vi "Text control 2 v7.4.vi"() -> ()   [LabVIEW 2019]
panel:
  in  "Tab Control":enum32{"Main", "Other parameters"}(tab)
  out "Vdg vs time (Bias Stress)":cluster{"Y data in":dbl[], "X data in":dbl[]}[](graph)
  out "Vp vs Vg (FPP)":cluster{"Y data in":dbl[], "X data in":dbl[]}[](graph)
  out "Vp2":dbl format="%.2e"
  out "Vp1":dbl format="%.2e"
  out "Vp vs time (FPP Bias Stress)":cluster{"Y data in":dbl[], "X data in":dbl[]}[](graph)
  in  "Plot sample extrema vs time":bool
  out "Line running":i32
  out "Total lines":i32
  out "Path":path=path "C:/users/rlp38/09Apr2009LTtesting/test2.txt"
  out "I vs Vg":cluster{"Y data in":dbl[], "X data in":dbl[]}[](graph)
  out "Is max":dbl format="%.2e"
  out "Id max":dbl format="%.2e"
  out "Ig max":dbl format="%.2e"
  out "Imax vs time":cluster{"Y data in":dbl[], "X data in":dbl[]}[](graph)
  out "Imin vs time":cluster{"Y data in":dbl[], "X data in":dbl[]}[](graph)
  out "I vs Vd":cluster{"Y data in":dbl[], "X data in":dbl[]}[](graph)
  in  "Script":string="#pulsedstressV d 0.03 20 0 0.5 0.0827 5\n#\n#itime m\n#gaterangemode a\n#drainrangemode a\n#pulsed on 0.05 0 0.02\n#transfer d -10 40 1 5 40 35\n#transfer d -10 40 1 5 40 35\n#transfer d -10 40 1 5 40 35\n#output d 0 40 20 0 40 1\n#\n#\n#sample 1 0.008 221 6 0.003\n#samplei 400e-6 200 6 0.002 0.1\n#vsu2pulse -10 4\n#\n#stressV 0.016 0.03 2e-4 0.1e-3 11\n#stressI 220e-7 0.08 15\n#transfer s -1 1 0.5 -0.005 0.005 0.005\n#output s 0 0 0 -0.008 0.008 0.002"
  out "Command running:":string
  out "Serial port data":string
  out "Elapsed Time":dbl caption="Elapsed Time (s)"
  in  "Time Units":u16(ring)=1 items=["Seconds", "Minutes", "Hours"]
  in  "Time Offset":dbl caption="Set Start Time (s)"
  in  "Reset":bool
  in  "Auto Reset":bool
  in  "integration time":u32(slide) max=2 step=1 scale=0.0..2.0
  out "Is on":dbl format="%.2e"
  out "Id on":dbl format="%.2e"
  out "Ig on":dbl format="%.2e"
  out "Ion vs time":cluster{"Y data in":dbl[], "X data in":dbl[]}[](graph)
  out "Ioff vs time":cluster{"Y data in":dbl[], "X data in":dbl[]}[](graph)
  out "Ig min":dbl format="%.2e"
  out "Id min":dbl format="%.2e"
  out "Is min":dbl format="%.2e"
  out "Is off":dbl format="%.2e"
  out "Id off":dbl format="%.2e"
  out "Ig off":dbl format="%.2e"
  in  "Integration time (long)":dbl=0.32 min=0.04 max=2.0 step=0.02 format="%.2f"
  in  "Integration time (short)":dbl=0.0019 min=8e-05 max=0.0019 step=8e-05 format="%^.0e"
  in  "Drain: Compliance":dbl=0.001 format="%.8f"
  in  "Gate: Compliance":dbl=0.001 format="%.8f"
  in  "Interrupt scan":bool
  in  "Interrupt program":bool
  in  "Plot output curve extrema vs time":bool
  in  "Plot transfer curve extrema vs time":bool
  out "I vs time (Bias Stress)":cluster{"Y data in":dbl[], "X data in":dbl[]}[](graph)
  in  "Sample I - Probe 4 (Disabled)":u32(ring)=3 items=["SMU1  ", "SMU2  ", "SMU3  ", "SMU4  ", "SMU5  ", "SMU6  ", "VSU1  ", "VSU2  "]
  in  "Sample I - Source/Common":u32(ring) items=["SMU1  ", "SMU2  ", "SMU3  ", "SMU4  ", "SMU5  ", "SMU6  ", "VSU1  ", "VSU2  "]
  in  "Sample I - Probe 3 (Disabled)":u32(ring)=2 items=["SMU1  ", "SMU2  ", "SMU3  ", "SMU4  ", "SMU5  ", "SMU6  ", "VSU1  ", "VSU2  "]
  in  "Sample I - Drain/Gate":u32(ring)=1 items=["SMU1  ", "SMU2  ", "SMU3  ", "SMU4  ", "SMU5  ", "SMU6  ", "VSU1  ", "VSU2  "]
  in  "Sample - Probe 4":u32(ring)=3 items=["SMU1  ", "SMU2  ", "SMU3  ", "SMU4  ", "SMU5  ", "SMU6  ", "VSU1  ", "VSU2  "]
  in  "Sample - Source/Common":u32(ring) items=["SMU1  ", "SMU2  ", "SMU3  ", "SMU4  ", "SMU5  ", "SMU6  ", "VSU1  ", "VSU2  "]
  in  "Sample - Gate":u32(ring)=2 items=["SMU1  ", "SMU2  ", "SMU3  ", "SMU4  ", "SMU5  ", "SMU6  ", "VSU1  ", "VSU2  "]
  in  "Sample - Drain":u32(ring)=1 items=["SMU1  ", "SMU2  ", "SMU3  ", "SMU4  ", "SMU5  ", "SMU6  ", "VSU1  ", "VSU2  "]
  in  "Gate Range\nmode":u16(ring) items=["Auto", "Limited", "Fixed"]
  in  "Gate Range":u8(slide)=3 max=11 scale=0.0..11.0
  in  "Source/Drain\nRange mode":u16(ring) items=["Auto", "Limited", "Fixed"]
  in  "Source/Drain Range":u8(slide)=3 max=11 scale=0.0..11.0
  in  "Panel Controls":T1={"Emergency Stop"=refnum, "TransGraph Max"=1e-05, "Text/Graph (text=false)"=TRUE} {"TransGraph Max" format="%.2e"}
  in  "Panel Controls 2":T2={"Emergency Stop"=refnum, "TransGraph Max"=1e-05, "Text/Graph (text=false)"=TRUE, "TransGraph Min"=1e-11} {"TransGraph Min" format="%.2e"; "TransGraph Max" format="%.2e"}
  out "error out":errorcluster
  in  "Delay before read (ms)":u32=1000
  in  "byte count":u32=64
  in  "Serial End Mode for Reads":u16(ring)=2 items=["None", "LastBit", "TermChar"]
  in  "Timeout (ms)":u32=10000
  in  "Enable Termination\nChar (T)":bool=TRUE
  in  "Termination char\n(0xA = '\\n' = LF)\n(0xD = '\\r' = CR)":u8=13 format="%.0x"
  in  "flow control":u16(ring) items=["None"=0, "XON/XOFF"=1, "RTS/CTS"=2, "DTR/DSR"=4]
  in  "stop bits":u16(ring)=10 items=["1.0"=10, "1.5"=15, "2.0"=20]
  in  "parity":u16(ring) items=["None", "Odd", "Even", "Mark", "Space"]
  in  "data bits":u16=8 min=5 max=8 step=1
  in  "VISA resource name":refnum<visa-resource-name>="COM6"
  in  "baud rate":u32=9600
  out "Timings Indicator":T3
  in  "Timings (overwritten by the Front Panel)":T4={"integration time"=0, "Short/Long integration time"=0.00064, "hold time (sec)"=0.0, "delay time (sec)"=0.0, "Step Time (0 disables)"=0.0, "sweep method"=0, "Pulse period"=0.005, "Base voltage"=0.0, "Pulse width"=0.0005} {"Pulse width" min=0.0005 max=0.1 step=0.0001 format="%.4f"; "Base voltage" format="%^.4e"; "Pulse period" min=0.005 max=1.0 step=0.0001 format="%.4f"; "sweep method" items=["Continuous", "Pulsed"]; "Step Time (0 disables)" format="%.2f"; "delay time (sec)" format="%.4f"; "hold time (sec)" format="%.4f"; "Short/Long integration time" format="%^.0e"; "integration time" scale=0.0..2.0}
  in  "Probe 4":cluster{"on/off":bool, "Voltage":dbl} {"Voltage" min=-100.0 max=100.0 format="%.2f"}
  in  "Full Reset":bool
  in  "Standby":T5
  out "Probe 4 Indicator":cluster{"on/off":bool, "Voltage":dbl} {"Voltage" min=-100.0 max=100.0 format="%.2f"}
  in  "Transfer/Output - Drain":u32(ring)=1 items=["SMU1  ", "SMU2  ", "SMU3  ", "SMU4  ", "SMU5  ", "SMU6  ", "VSU1  ", "VSU2  "]
  in  "Transfer/Output - Gate":u32(ring)=2 items=["SMU1  ", "SMU2  ", "SMU3  ", "SMU4  ", "SMU5  ", "SMU6  ", "VSU1  ", "VSU2  "]
  in  "Transfer/Output - Source/Common":u32(ring) items=["SMU1  ", "SMU2  ", "SMU3  ", "SMU4  ", "SMU5  ", "SMU6  ", "VSU1  ", "VSU2  "]
  in  "Transfer/Output - Probe 4":u32(ring)=3 items=["SMU1  ", "SMU2  ", "SMU3  ", "SMU4  ", "SMU5  ", "SMU6  ", "VSU1  ", "VSU2  "]
  in  "Pulsed Stress V - Probe 4":u32(ring)=3 items=["SMU1  ", "SMU2  ", "SMU3  ", "SMU4  ", "SMU5  ", "SMU6  ", "VSU1  ", "VSU2  "]
  in  "Pulsed Stress V - Vextra":u32(ring)=6 items=["SMU1  ", "SMU2  ", "SMU3  ", "SMU4  ", "SMU5  ", "SMU6  ", "VSU1  ", "VSU2  "]
  in  "Pulsed Stress V - Drain":u32(ring)=1 items=["SMU1  ", "SMU2  ", "SMU3  ", "SMU4  ", "SMU5  ", "SMU6  ", "VSU1  ", "VSU2  "]
  in  "Pulsed Stress V - Source/Common":u32(ring) items=["SMU1  ", "SMU2  ", "SMU3  ", "SMU4  ", "SMU5  ", "SMU6  ", "VSU1  ", "VSU2  "]
  in  "Pulsed Stress V - Gate":u32(ring)=2 items=["SMU1  ", "SMU2  ", "SMU3  ", "SMU4  ", "SMU5  ", "SMU6  ", "VSU1  ", "VSU2  "]
  in  "FPP - Drain":u32(ring)=1 items=["SMU1  ", "SMU2  ", "SMU3  ", "SMU4  ", "SMU5  ", "SMU6  ", "VSU1  ", "VSU2  "]
  in  "FPP - Gate":u32(ring)=2 items=["SMU1  ", "SMU2  ", "SMU3  ", "SMU4  ", "SMU5  ", "SMU6  ", "VSU1  ", "VSU2  "]
  in  "FPP - Probe 1":u32(ring) items=["SMU1  ", "SMU2  ", "SMU3  ", "SMU4  ", "SMU5  ", "SMU6  ", "VSU1  ", "VSU2  "]
  in  "FPP - Probe 2":u32(ring)=3 items=["SMU1  ", "SMU2  ", "SMU3  ", "SMU4  ", "SMU5  ", "SMU6  ", "VSU1  ", "VSU2  "]
  in  "FPP - Source":u32(ring)=6 items=["SMU1  ", "SMU2  ", "SMU3  ", "SMU4  ", "SMU5  ", "SMU6  ", "VSU1  ", "VSU2  "]
  in  "Stress V - Drain":u32(ring)=1 items=["SMU1  ", "SMU2  ", "SMU3  ", "SMU4  ", "SMU5  ", "SMU6  ", "VSU1  ", "VSU2  "]
  in  "Stress V - Gate":u32(ring)=2 items=["SMU1  ", "SMU2  ", "SMU3  ", "SMU4  ", "SMU5  ", "SMU6  ", "VSU1  ", "VSU2  "]
  in  "Stress V - Source/Common":u32(ring) items=["SMU1  ", "SMU2  ", "SMU3  ", "SMU4  ", "SMU5  ", "SMU6  ", "VSU1  ", "VSU2  "]
  in  "Stress I - Drain/Gate":u32(ring)=1 items=["SMU1  ", "SMU2  ", "SMU3  ", "SMU4  ", "SMU5  ", "SMU6  ", "VSU1  ", "VSU2  "]
  in  "Stress I - Source/Common":u32(ring) items=["SMU1  ", "SMU2  ", "SMU3  ", "SMU4  ", "SMU5  ", "SMU6  ", "VSU1  ", "VSU2  "]
  in  "VSU2 Stress - Source/Common":u32(ring) items=["SMU1  ", "SMU2  ", "SMU3  ", "SMU4  ", "SMU5  ", "SMU6  ", "VSU1  "]
  in  "VISA resource name in":refnum<visa-resource-name>="GPIB0::14::INSTR"
  in  "Gate":T6={"Gate Start"=0.0, "Gate Stop"=2.0, "Gate Step (linear only)"=1.0, "Gate Compliance"=0.0001, "Gate PComp"=0.0, "Range mode"=0, "Range"=6} {"Range" max=11 scale=0.0..11.0; "Range mode" items=["Auto", "Limited", "Fixed"]; "Gate PComp" format="%^.2e"; "Gate Compliance" format="%^.2e"; "Gate Step (linear only)" format="%^.4e"; "Gate Stop" format="%^.4e"; "Gate Start" format="%^.4e"}
  in  "Drain 2":T7={"Drain Start"=0.0, "Drain Stop"=2.0, "Drain Compliance"=0.0001, "Drain Step"=1.0, "Drain PComp"=0.0, "Range mode"=0, "Range"=6} {"Range" max=11 scale=0.0..11.0; "Range mode" items=["Auto", "Limited", "Fixed"]; "Drain PComp" format="%^.2e"; "Drain Step" format="%^.4e"; "Drain Compliance" format="%^.2e"; "Drain Stop" format="%^.4e"; "Drain Start" format="%^.4e"}
  # "Time"
  # "Syntax:\nitime [s|m|l] time(sec): [s|m|l] determines the integration time setting (small|medium|long) and time sets the value.\nNOTE: The value of the integration time has to be within the range allowed by its category (s|m|l), otherwise, the closest value will be used. (e.g. if the category is set to short but the time value is very long, the actual value used will be the maximum short integration time.\nIntegration times:\n    Short: Default: 640 us. Range: 8E-5 - 1.92E-3 seconds.\n    Medium: Fixed at 1 NPL cycle (0.02 seconds).\n    Long: Default: 16 NPL cycles (0.32 seconds). Range: 2-100 NPL cycles (0.04 seconds - 2 seconds).\ngaterangemode [a|l|f]\ndrainrangemode [a|l|f]\npulsed [on|off] PulsePeriod(sec) PulseBaseVoltage PulseONWidth(sec)\nstandby [on l off]\nwait NumMilliseconds\nwait-min NumMinutes\n# texthere = comment\nProbe4 [ON|OFF] Voltage\ntransfer [s|d] VgStart VgStop VgStep VdStart VdStop VdStep\noutput [s|d] VgStart VgStop VgStep VdStart VdStop VdStep\nsample Vg Vd NumSamples Time(s) SampleInterval(s)\nsamplei Idg NumSamples Time(s) SampleInterval(s) VDGcompliance\n100 samples is approximately 13 seconds with medium integration\n# if in doubt use SampleInterval(s) = 0.004\n    NOTE: When doing bias stress measurements, it is best to set the Time Units to \"Seconds\", as the \"sample\" command has been configured to give the output to seconds.\nstressV VG VD IGcompliance IDcompliance Duration(sec)\nstressI IDG VDGcompliance Duration(sec)\nvsu2pulse Bias Duration(s)\npulsedstressV [s|d] VEstop VgON VgOFF Period(s) PulseONwidth(s) Vd\nsample-fpp Vg Vd NumSamples Time\nresample-fpp Vg Vd\ntransfer-fpp [s|d] VgStart VgStop VgStep VdStart VdStop VdStep\noutput-fpp [s|d] VgStart VgStop VgStep VdStart VdStop VdStep\nserial SerialPortCommand\nloop(No of iterations){Code}: Iterates the code provided (including nested loops)"
  # "1\n2\n3\n4\n5\n6\n7\n8\n9\n10\n11\n12\n13\n14\n15\n16\n17\n18\n19\n20"
  # "SMUs"
  # "Serial port settings"
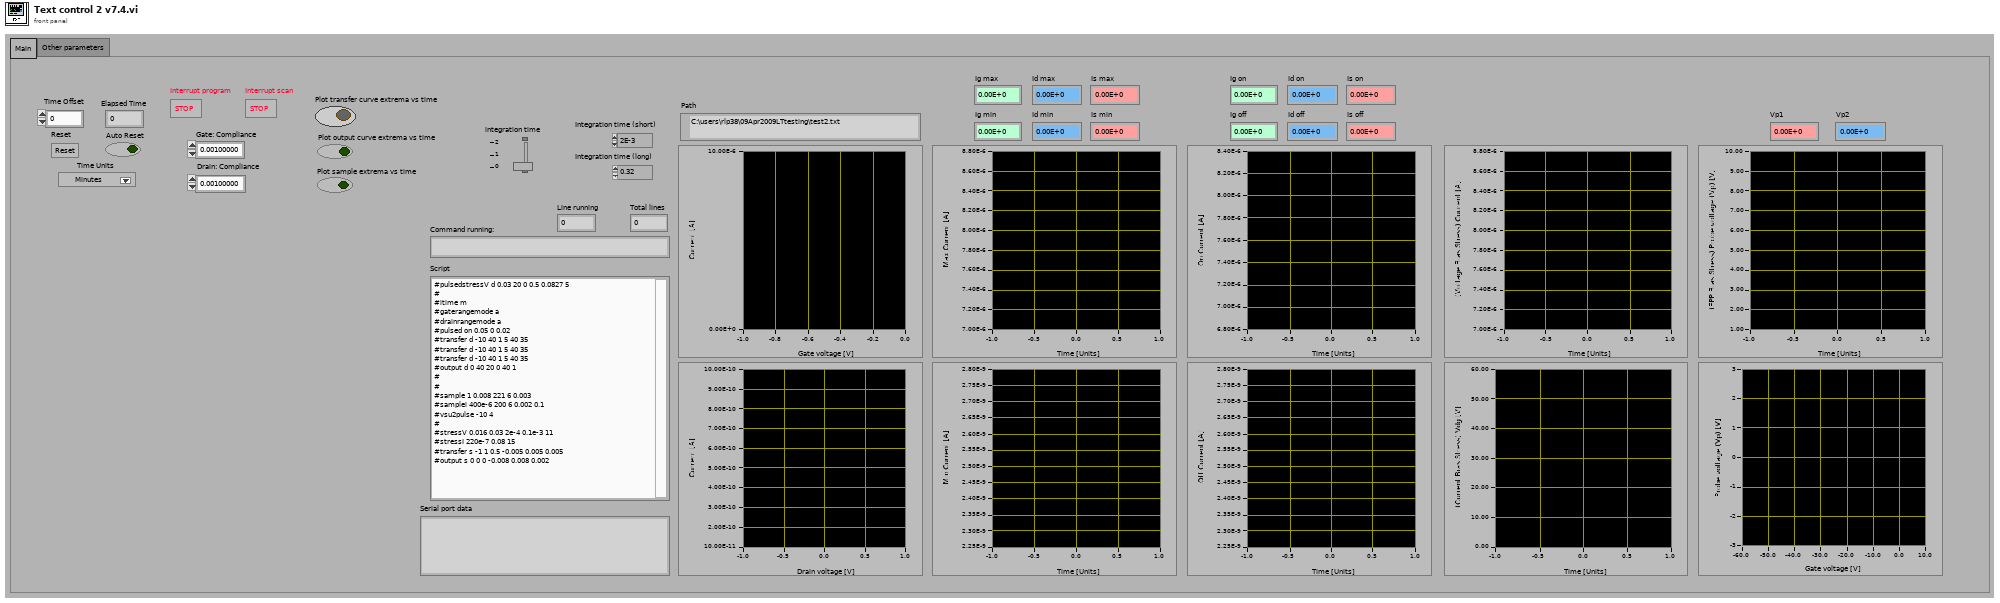
[diagram p1: front panel]
types:
  T1 = cluster{"Emergency Stop":refnum<vi>, "TransGraph Max":dbl, "Text/Graph (text=false)":bool}
  T2 = cluster{"Emergency Stop":refnum<vi>, "TransGraph Max":dbl, "Text/Graph (text=false)":bool, "TransGraph Min":dbl}
  T3 = cluster{"integration time (0:s, 1:m, 2:l)":u32, "Short/Long integration time":dbl, "hold time (sec)":dbl, "delay time (sec)":dbl, "Step Time (0 disables)":dbl, "sweep method":u16, "Pulse period":dbl, "Base voltage":dbl, "Pulse width":dbl}
  T4 = cluster{"integration time":u32, "Short/Long integration time":dbl, "hold time (sec)":dbl, "delay time (sec)":dbl, "Step Time (0 disables)":dbl, "sweep method":u16, "Pulse period":dbl, "Base voltage":dbl, "Pulse width":dbl}
  T5 = cluster{"Gate Standby":bool, "Drain Standby":bool}
  T6 = cluster{"Gate Start":dbl, "Gate Stop":dbl, "Gate Step (linear only)":dbl, "Gate Compliance":dbl, "Gate PComp":dbl, "Range mode":u16, "Range":u8}
  T7 = cluster{"Drain Start":dbl, "Drain Stop":dbl, "Drain Compliance":dbl, "Drain Step":dbl, "Drain PComp":dbl, "Range mode":u16, "Range":u8}
  T8 = enum16{"open", "replace", "create", "open or create", "replace or create", "replace or create with confirmation"}
  T9 = cluster{"V2 Start":dbl, "V2 Step":dbl, "Number of points":i32}
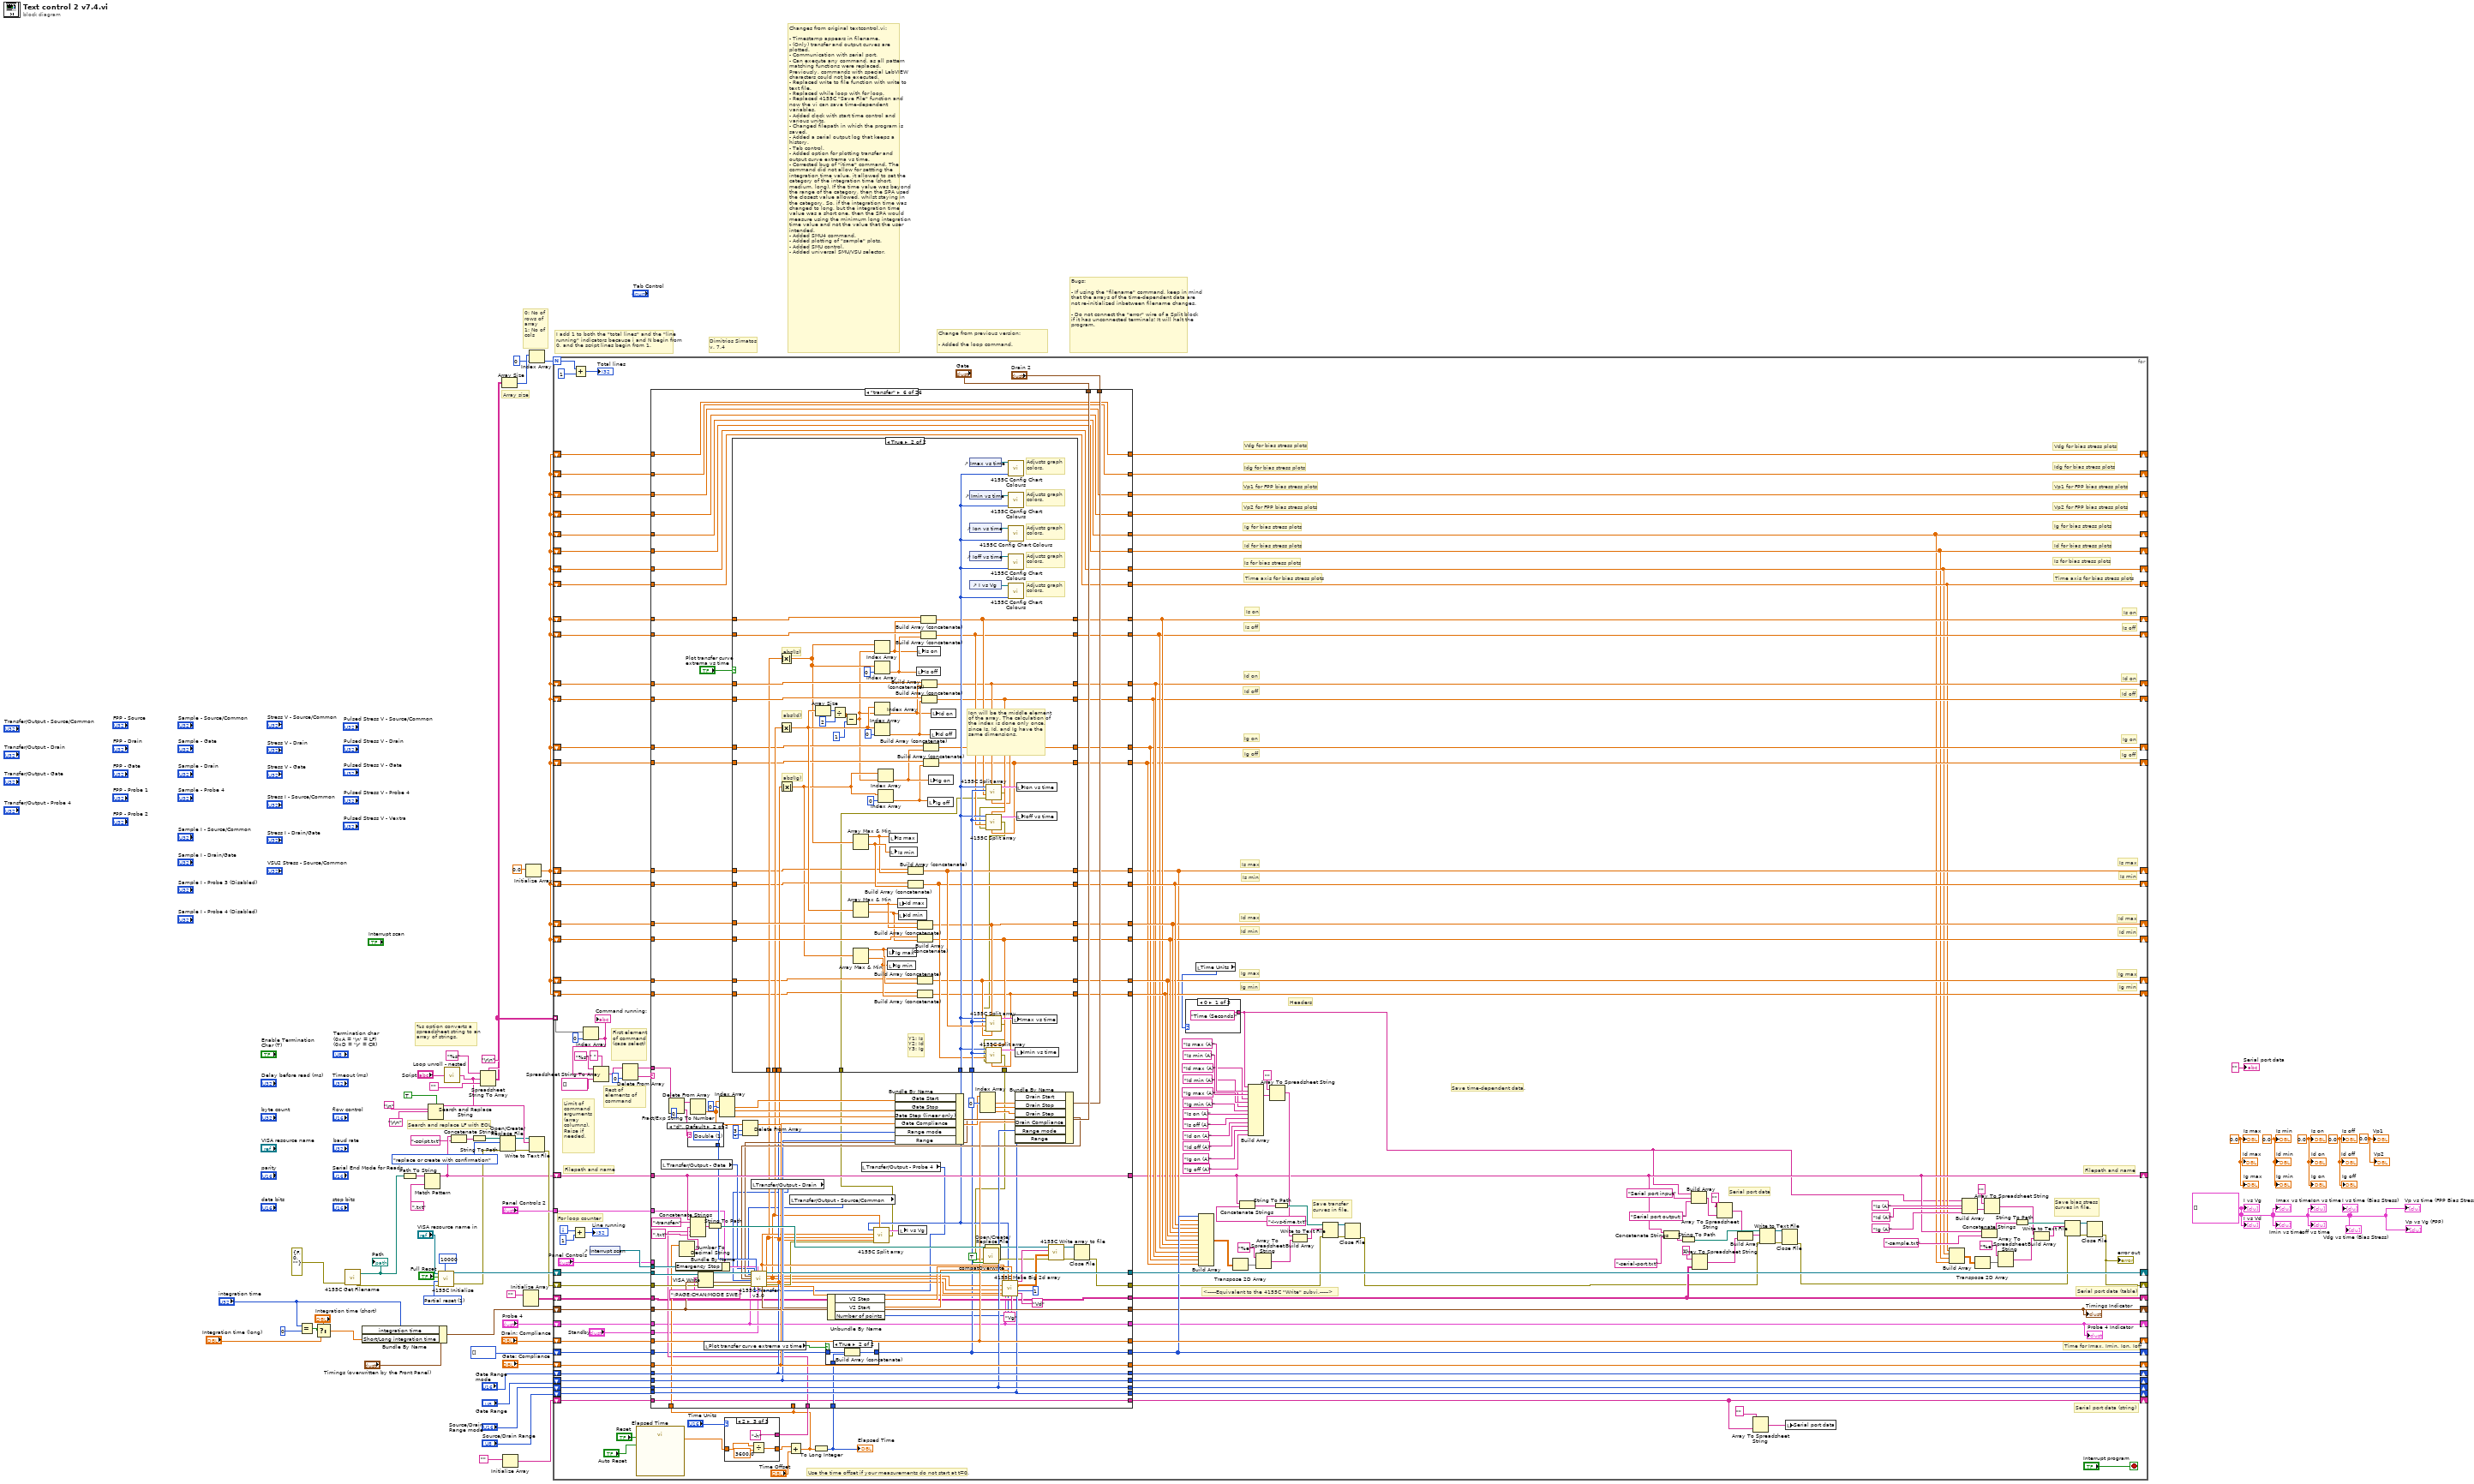
[diagram p0: block diagram]
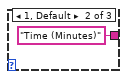
[diagram p2: hidden frame]
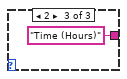
[diagram p3: hidden frame]
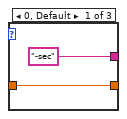
[diagram p4: hidden frame]
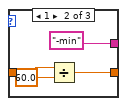
[diagram p5: hidden frame]
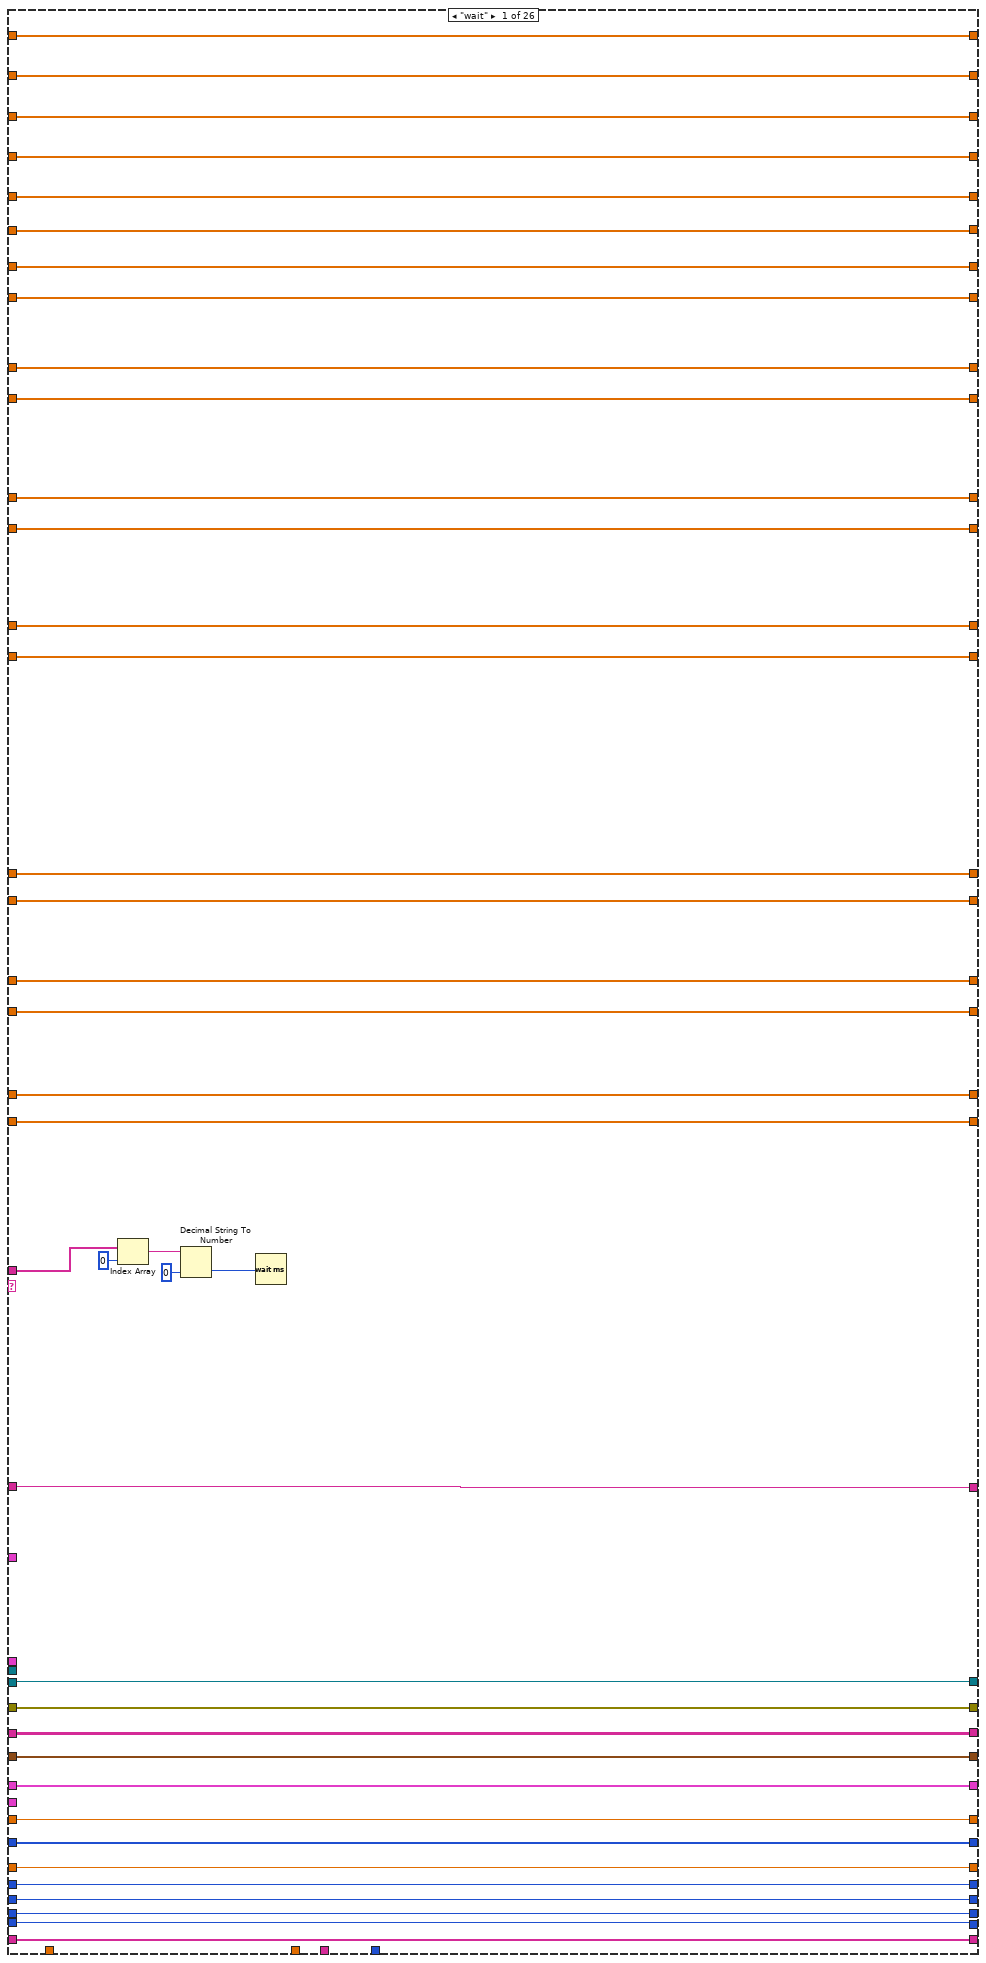
[diagram p6: hidden frame]
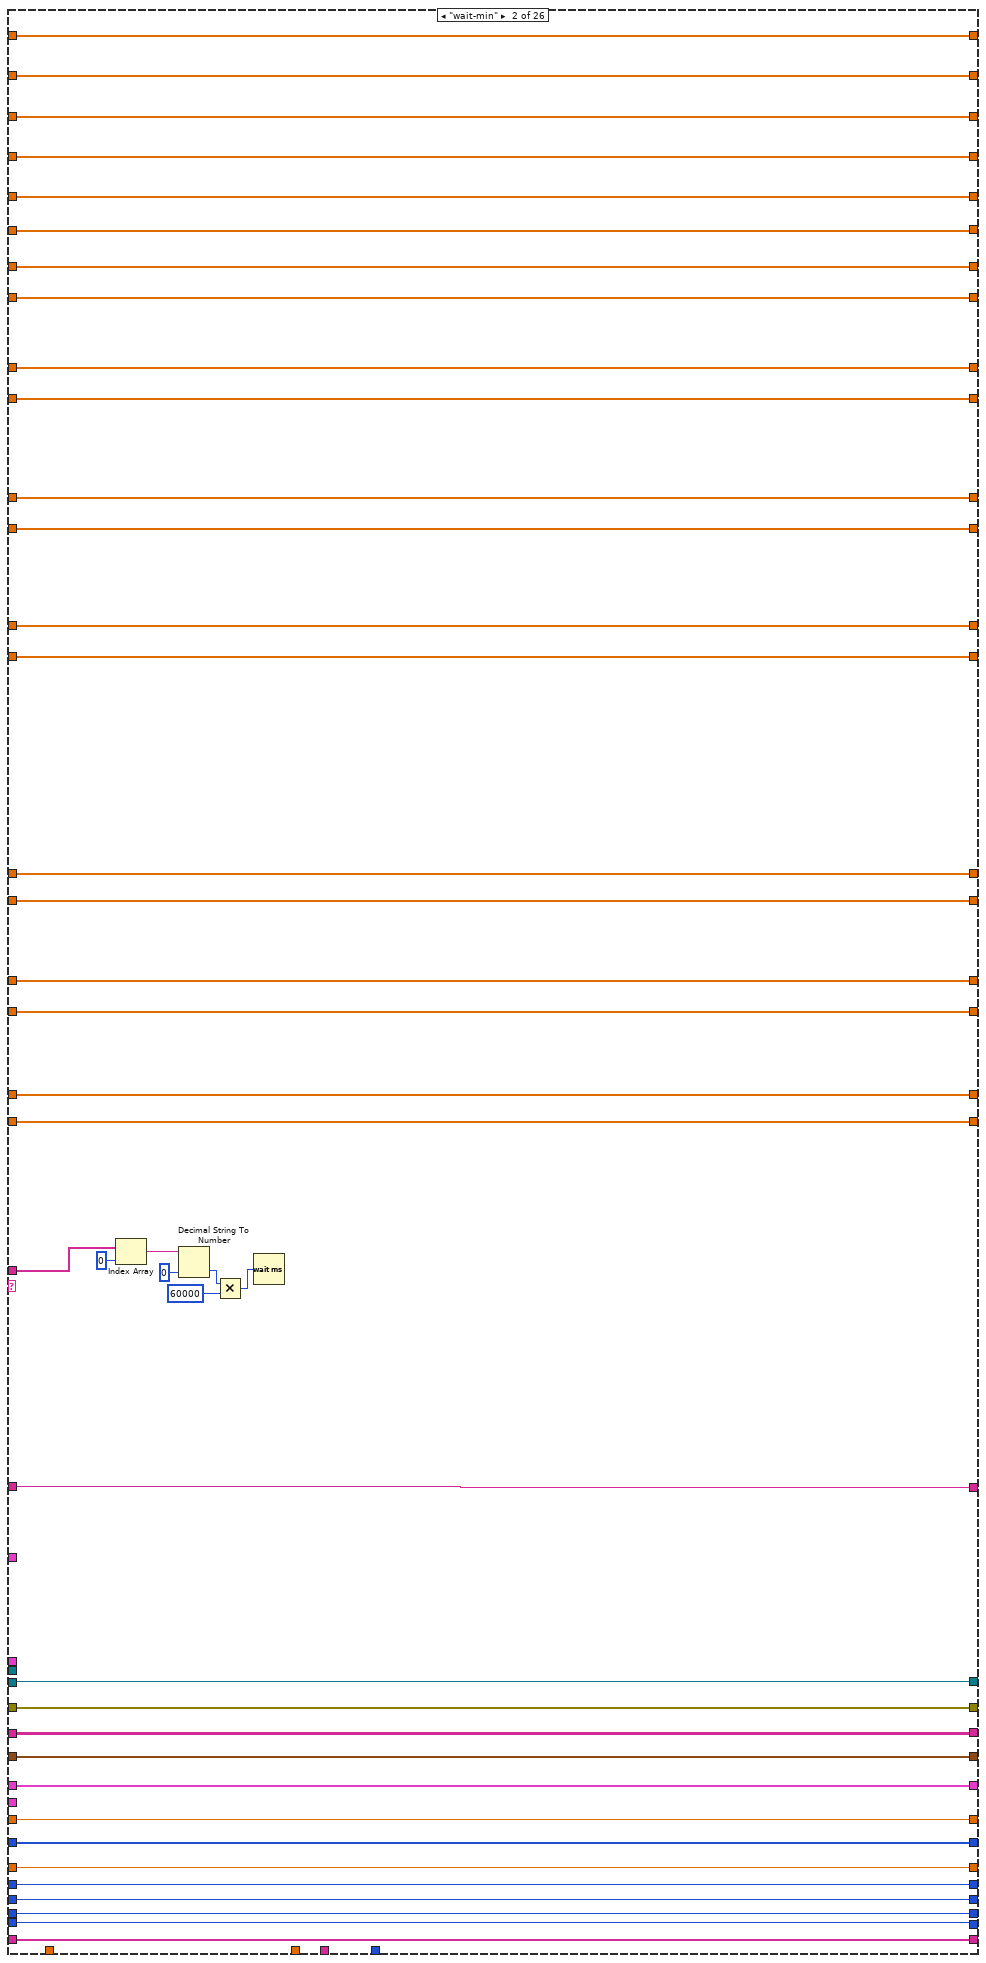
[diagram p7: hidden frame]
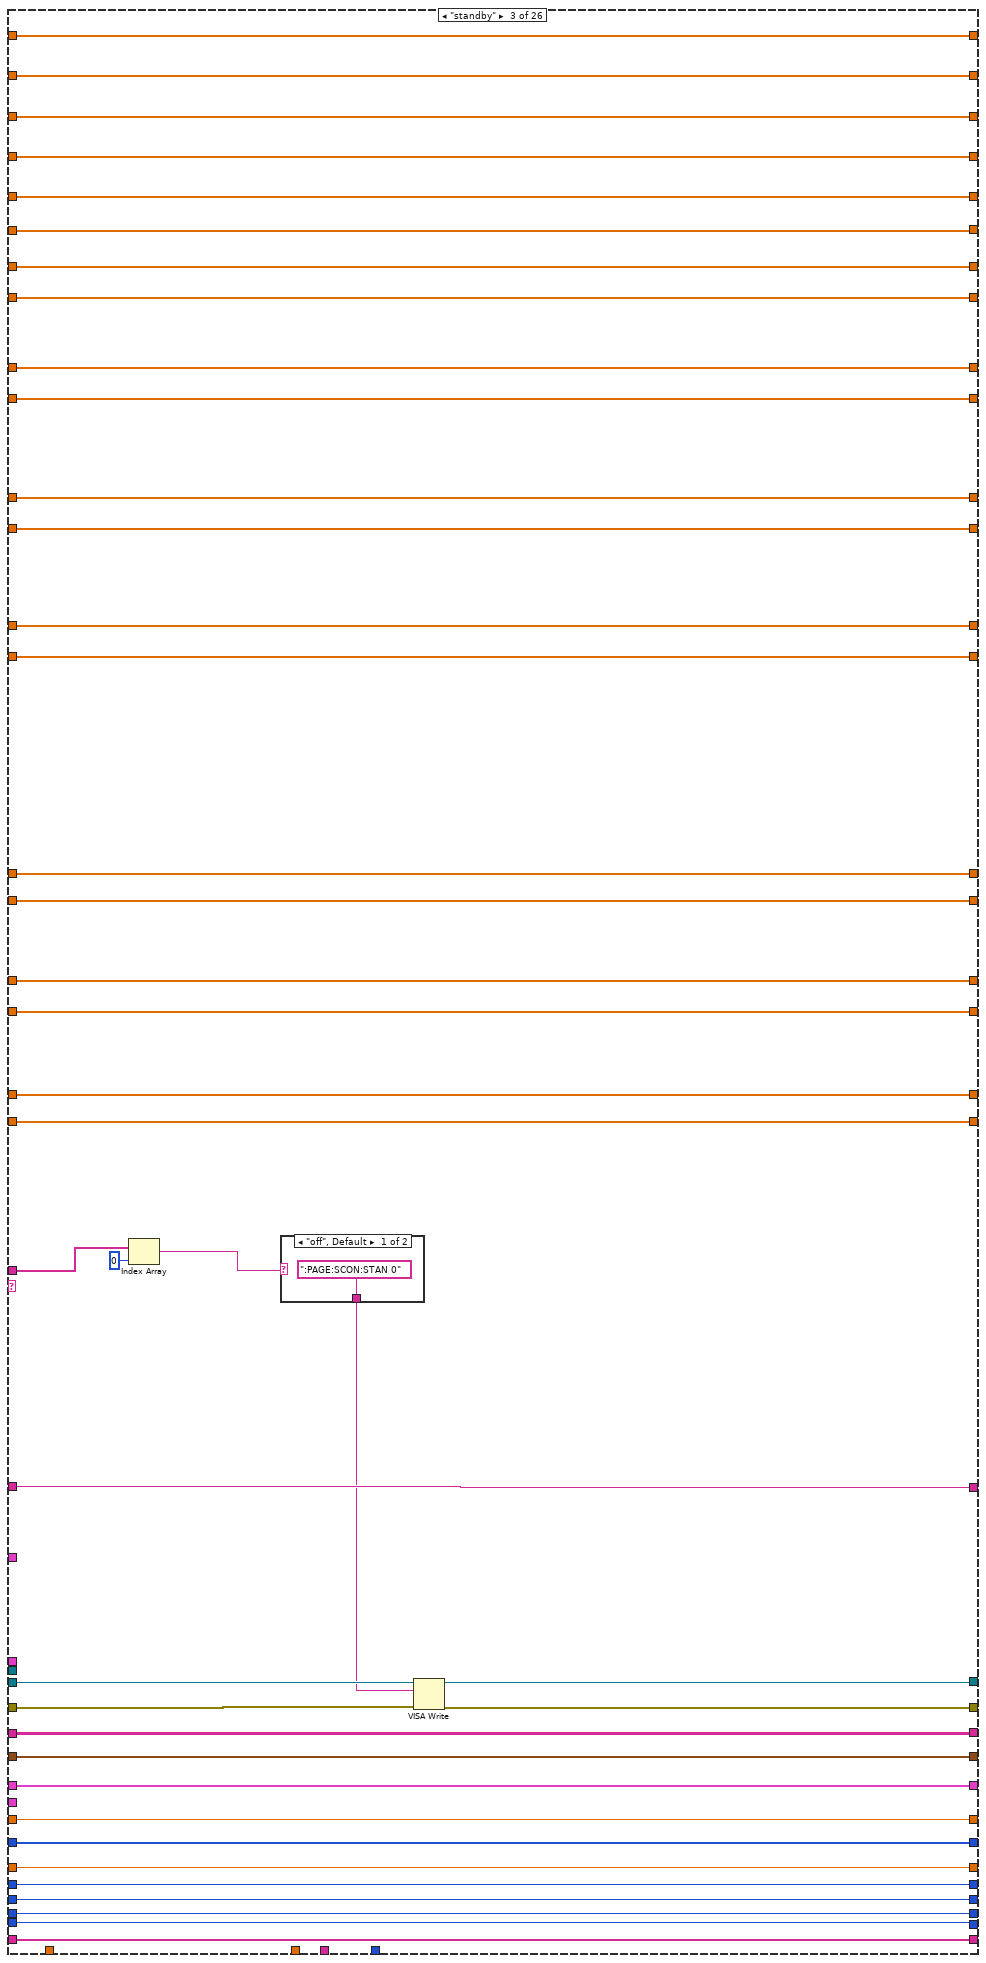
[diagram p8: hidden frame]
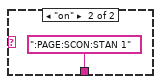
[diagram p9: hidden frame]
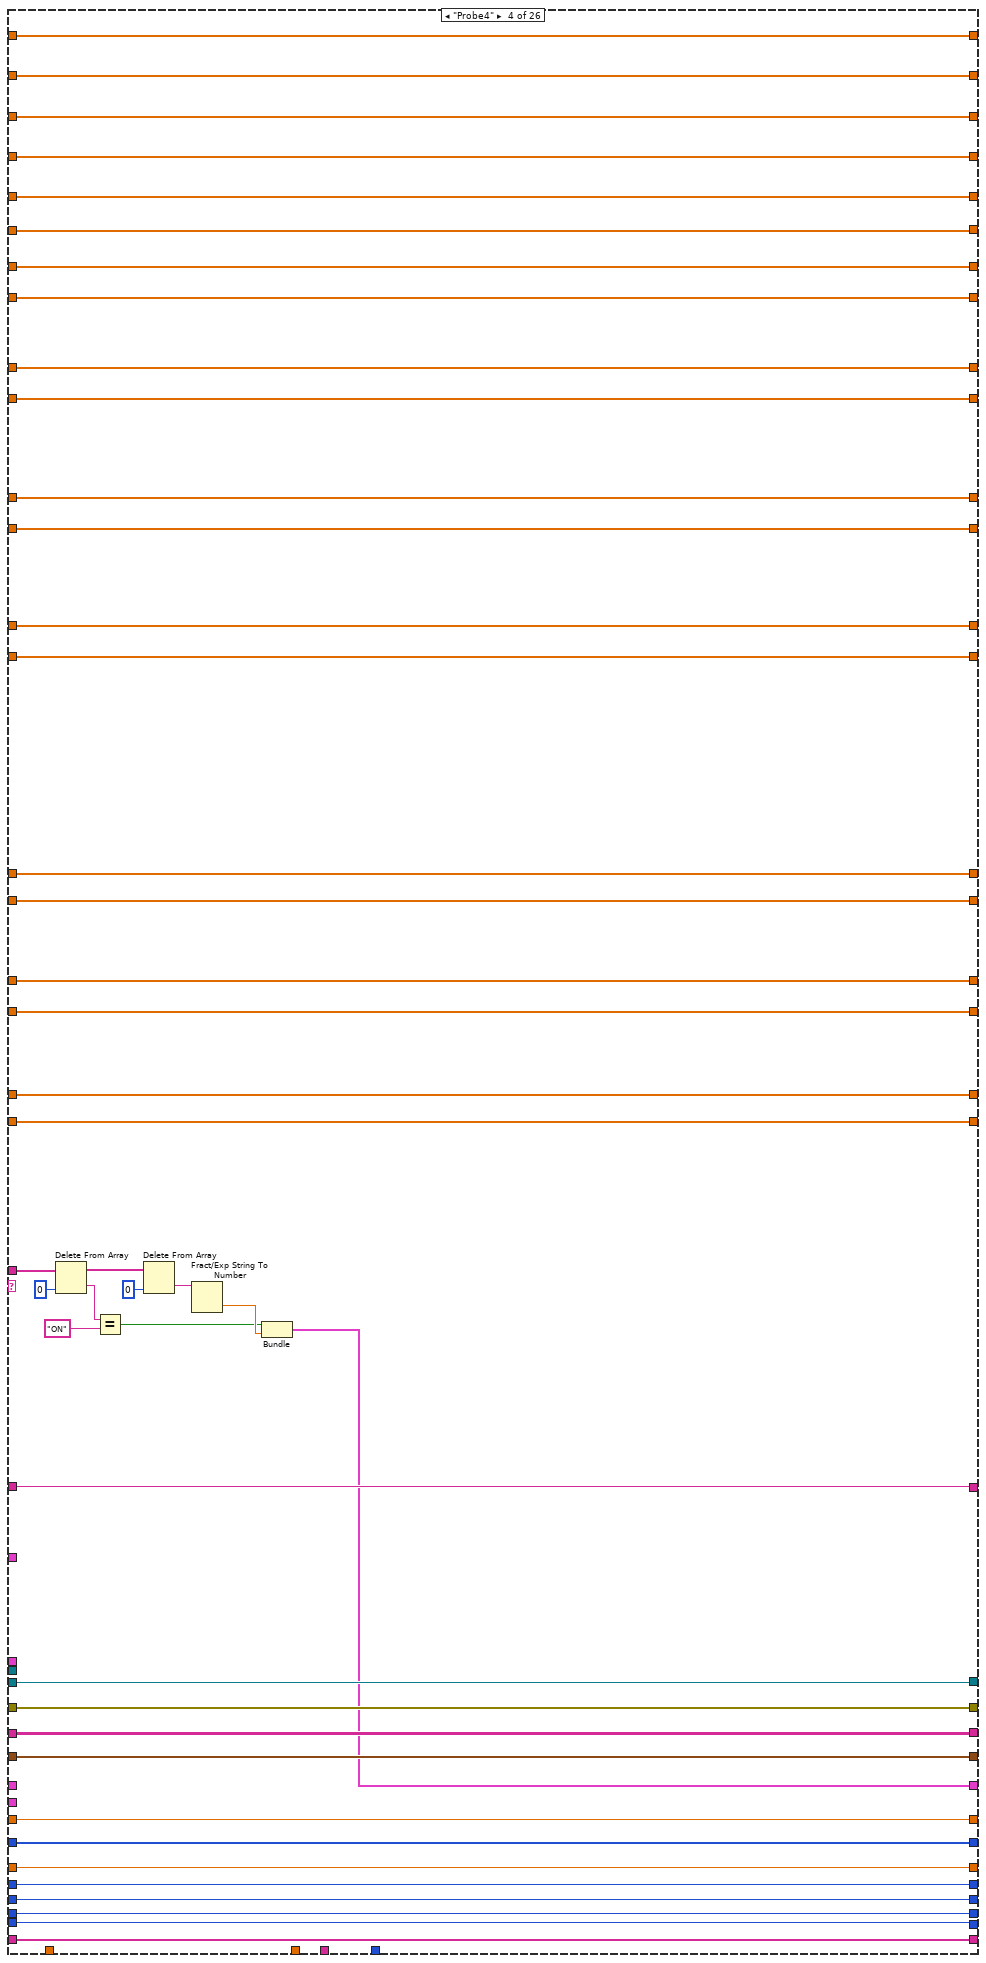
[diagram p10: hidden frame]
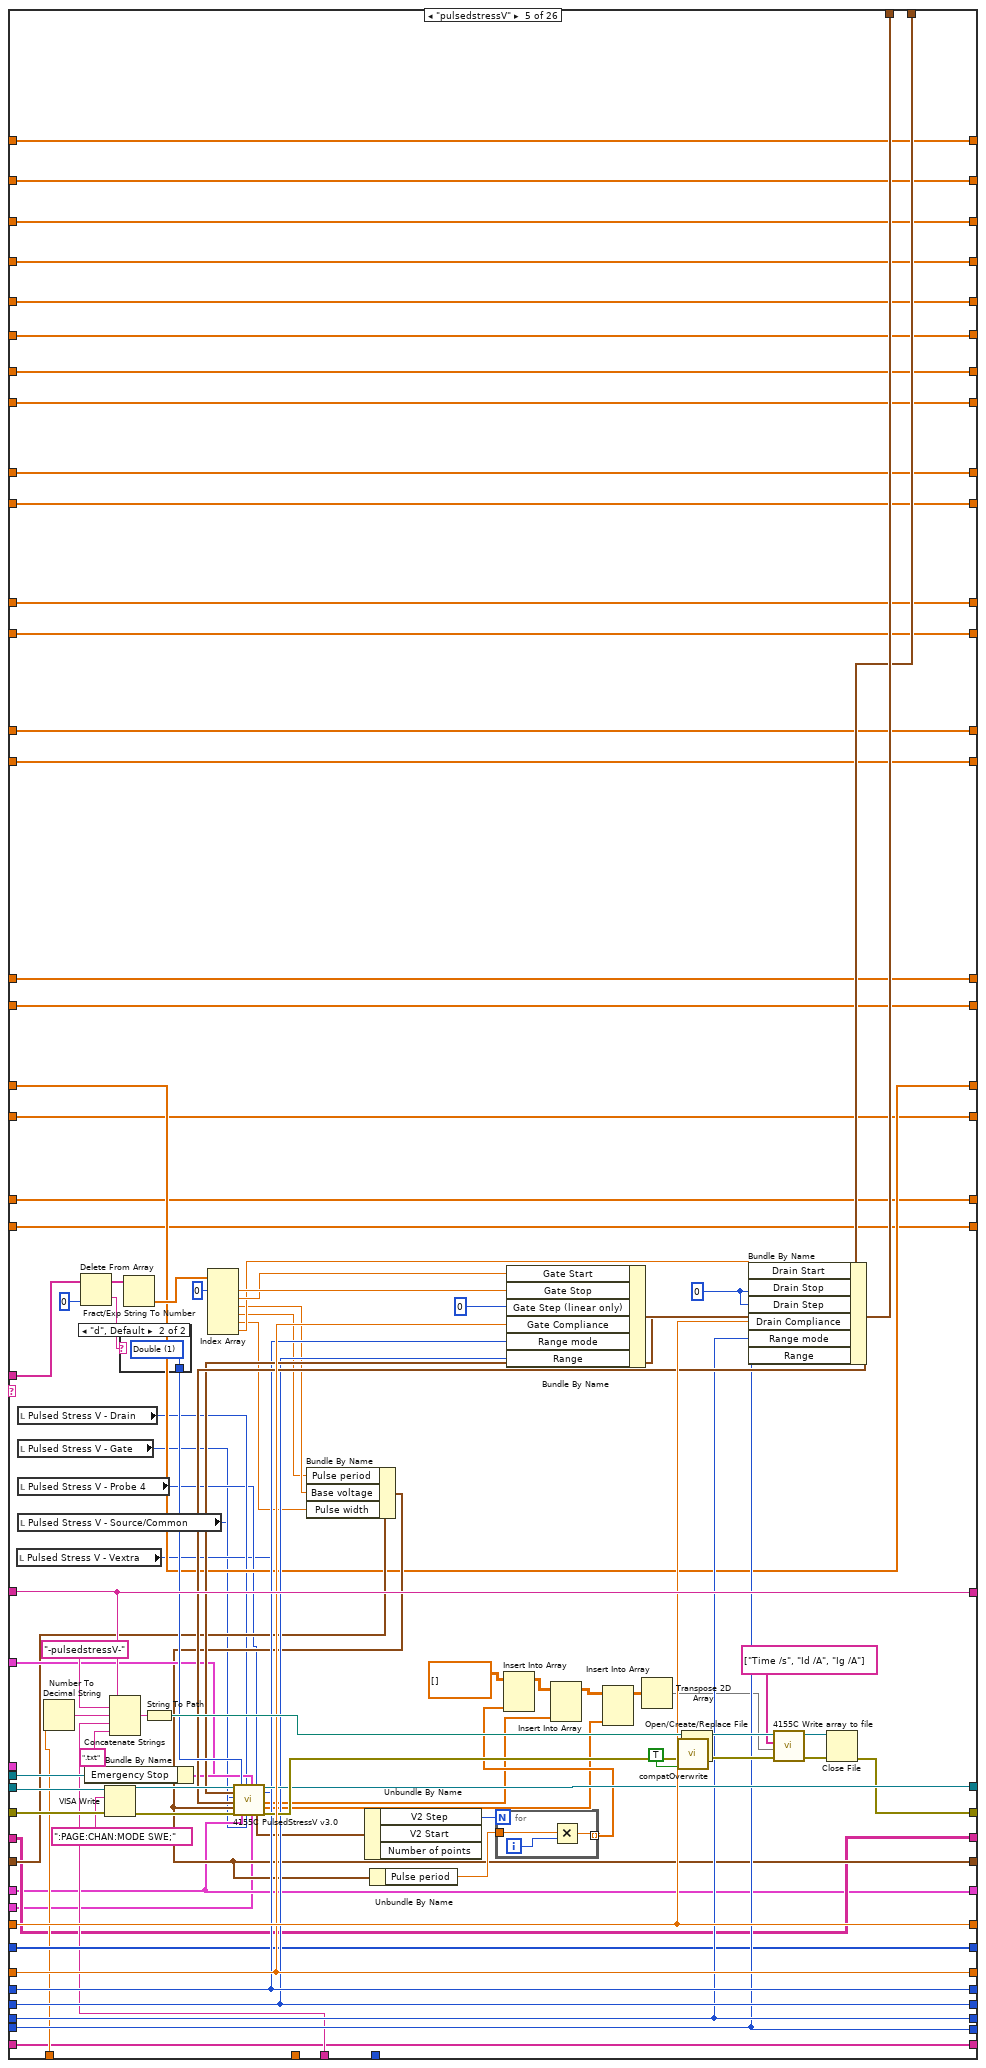
[diagram p11: hidden frame]
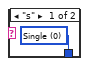
[diagram p12: hidden frame]
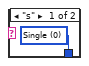
[diagram p15: hidden frame]
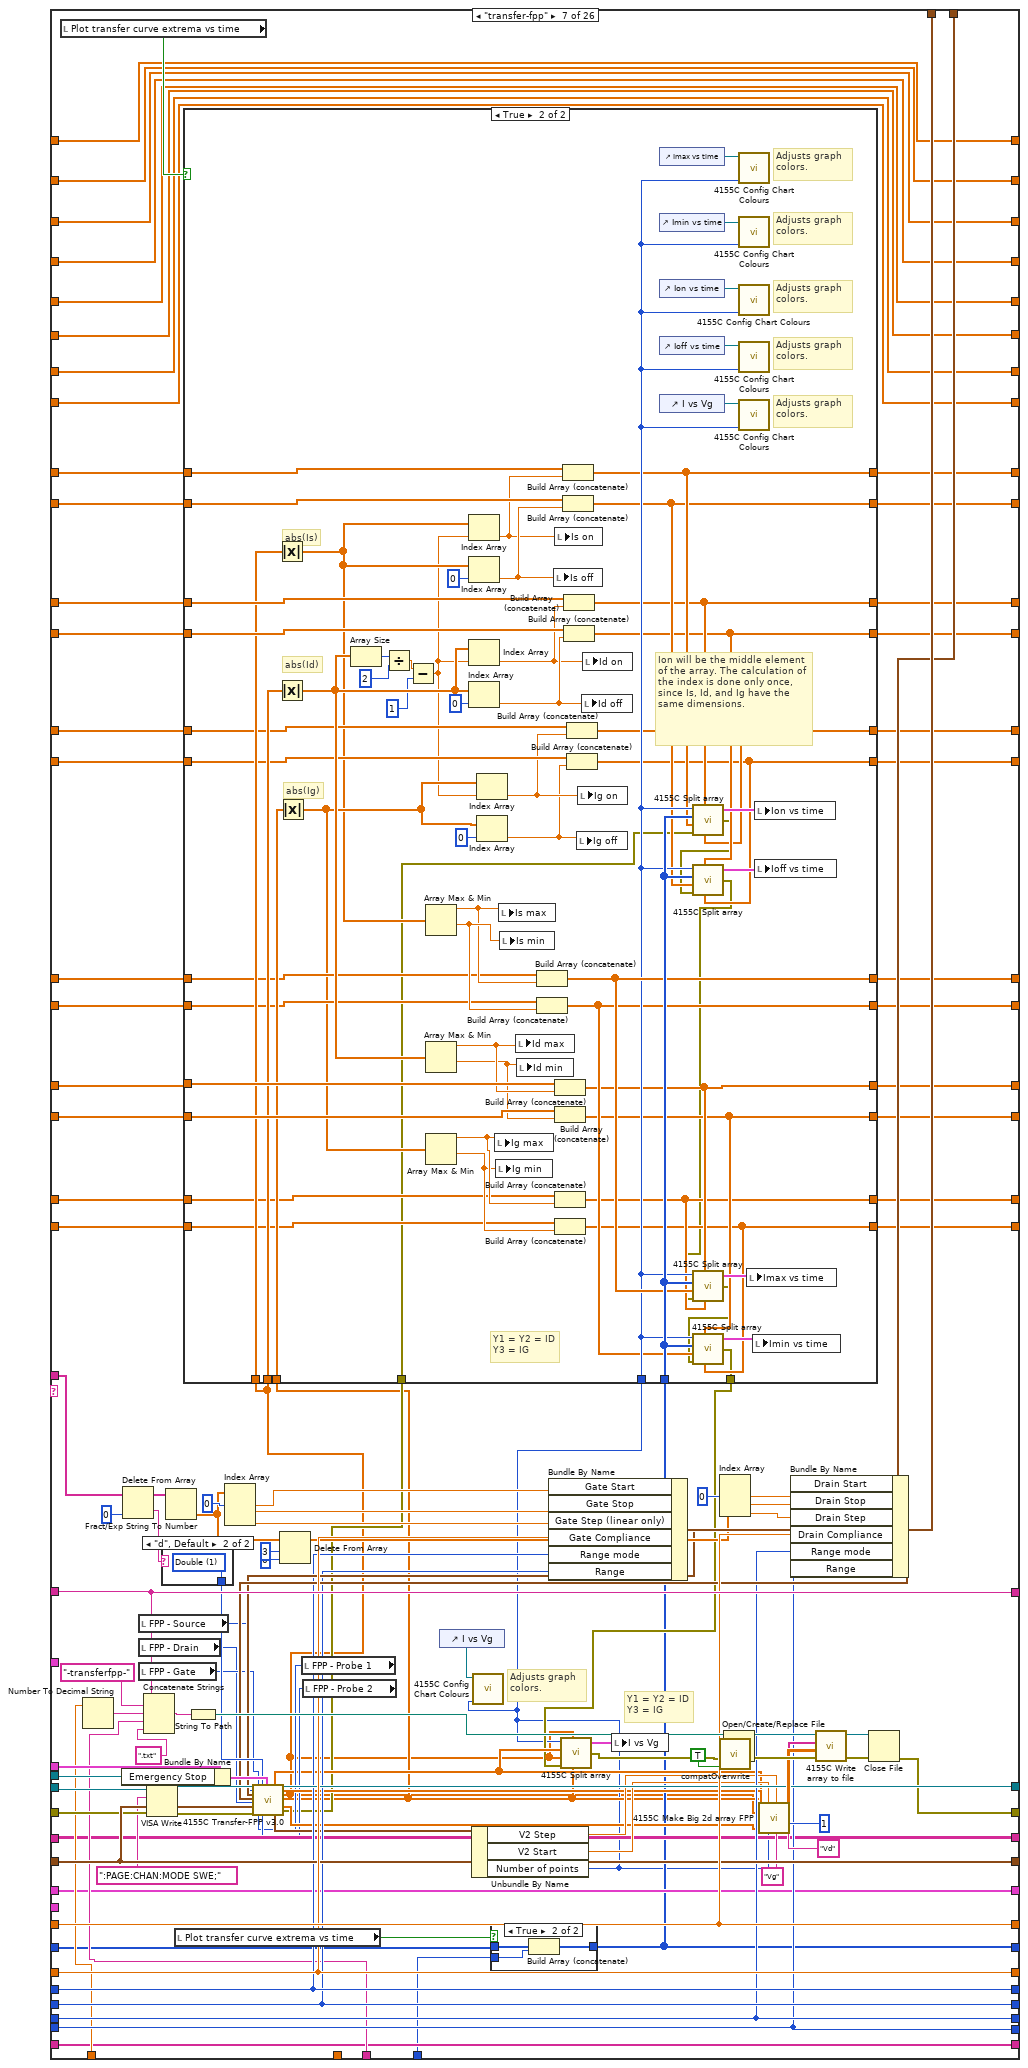
[diagram p16: hidden frame]
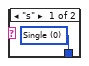
[diagram p19: hidden frame]
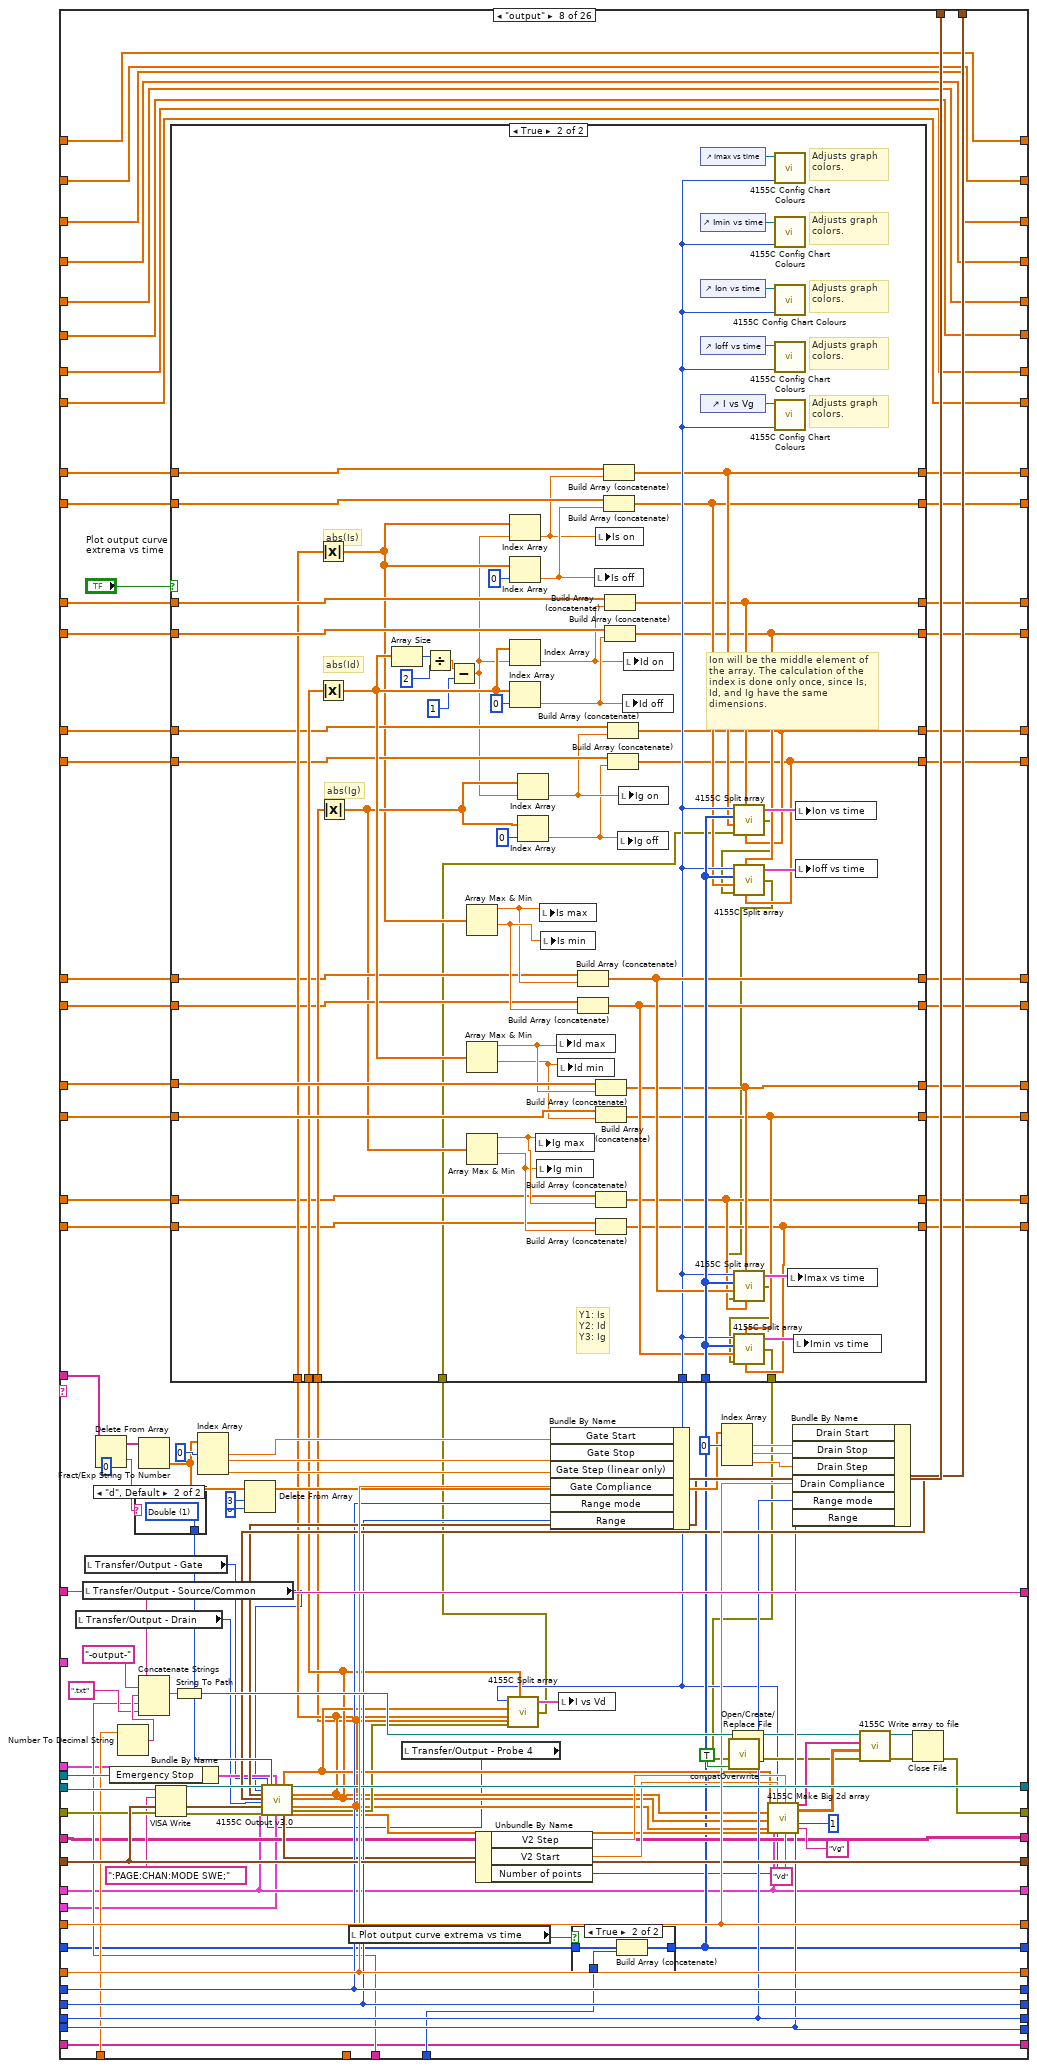
[diagram p20: hidden frame]
diagram:
  w5 = 0.0 ("Is off")
  w4 = cluster{"Y data in":dbl[], "X data in":dbl[]}[] [] ("I vs Vg")
  w12 = 0.0 ("Is off")
  w13 = 0.0 ("Is on")
  w14 = 0.0 ("Is min")
  w15 = 0.0 ("Is max")
  w57 = u16 1 items=["Reset All", "Partial reset"] ("Type of reset")
  # "Change from previous version:\n\n- Added the loop command."
  # "I add 1 to both the \"total lines\" and the \"line running\" indicators because i and N begin from 0, and the script lines begin from 1."
  # "Bugs:\n\n- If using the \"filename\" command, keep in mind that the arrays of the time-dependent data are not re-initialized inbetween filename changes. \n\n- Do not connect the \"error\" wire of a Split block if it has unconnected terminals! It will halt the program."
  # "Array size"
  # "%s option converts a spreadsheet string to an array of strings."
  # "0: No of rows of array\n1: No of cols"
  # "Dimitrios Simatos\nv. 7.4"
  # "Changes from original textcontrol.vi:\n\n- Timestamp appears in filename.\n- (Only) transfer and output curves are plotted.\n- Communication with serial port.\n- Can execute any command, as all pattern matching functions were replaced. Previously, commands with special LabVIEW characters could not be executed.\n- Replaced write to file function with write to text file.\n- Replaced while loop with for loop.\n- Replaced 4155C \"Save File\" function and now the vi can save time-dependent variables.\n- Added clock with start time control and various units.\n- Changed filepath in which the program is saved.\n- Added a serial output log that keeps a history.\n- Tab control.\n- Added option for plotting transfer and output curve extrema vs time.\n- Corrected bug of \"itime\" command. The command did not allow for settting the integration time value, it allowed to set the category of the integration time (short, medium, long). If the time value was beyond the range of the category, then the SPA used the closest value allowed, whilst staying in the category. So, if the integration time was changed to long, but the integration time value was a short one, then the SPA would measure using the minimum long integration time value and not the value that the user intended.\n- Added SMU4 command.\n- Added plotting of \"sample\" plots.\n- Added SMU control.\n- Added universal SMU/VSU selector."
  # "Search and replace LF with EOL"
  n1 = Equal?(x="integration time", y=u32 0) -> (x = y?=w58:bool)
  n2 = Select(t="Integration time (short)", s=w58, f="Integration time (long)") -> (s? t:f=w20:dbl)
  n3 = call "4155C Get Filename.vi"("error in (no error)"=errorcluster {"status"=FALSE, "code"=0, "source"=""}) -> ("error out"=w52:errorcluster, "path"=w28:path)  [unwired: 2 in, 1 out]
  "Path" <- w28
  n4 = Bundle By Name(cluster="Timings (overwritten by the Front Panel)", "integration time"="integration time", "Short/Long integration time"=w20) -> (w50:T4)
  n5 = Path To String(path=w28) -> (string=w29:string)
  n6 = Match Pattern(string=w29, regular expression=".txt") -> (before substring=w18:string)  [unwired: 1 in, 3 out]
  n7 = call "4155C Initialise.vi"("VISA resource name in"="VISA resource name in", "Reset"="Full Reset", "Type of reset"=w57, "error in (no error)"=w52, "VISA Timeout Value"=u32 10000) -> ("VISA Resource Name out"=w51:refnum<visa-resource-name>, "error out"=w10:errorcluster)
  n8 = call "Loop unroll - nested.vi"("Script"="Script") -> ("Output"=w2:string)
  n9 = Search and Replace String(replace all?=TRUE ("replace all? (F)"), input string=w2, search string="\n", replace string="\r\n") -> (result string=w40:string)  [unwired: 4 in, 3 out]
  n10 = Concatenate Strings(w18, "-script.txt" ("string")) -> (w19:string)
  n11 = String To Path(string=w19) -> (path=w8:path)
  n12 = Spreadsheet String To Array(delimiter (Tab)="\r\n", format string="%s", spreadsheet string=w2, array type (2D Dbl)="") -> (array=w31:string[][])
  n13 = Open/Create/Replace File(file path (use dialog)=w8, error in=w10, operation (0:open)=T8."replace or create with confirmation") -> (refnum out=w7:refnum<file>, error out=w9:errorcluster)  [unwired: 3 in, 1 out]
  n14 = Array Size(array=w31) -> (size(s)=w35:i32[])
  n15 = Initialize Array("") -> (w23:string[])  [unwired: 1 in]
  n16 = Initialize Array("") -> (w21:string[][])  [unwired: 2 in]
  n17 = Initialize Array(0.0 ("element")) -> (w3:dbl[])  [unwired: 1 in]
  n18 = Index Array(array=w35, index=0) -> (element=w33:i32)
  n19 = Write to Text File(file (use dialog)=w7, text=w40, error in=w9) -> (error out=w26:errorcluster)  [unwired: 1 in, 2 out]
  n20 = for {
    N: w33 -> [w167]
    shift-left: "Source/Drain Range" -> [w207]
    shift-right: [w203] -> _
    shift-left: "Source/Drain\nRange mode" -> [w208]
    shift-right: [w204] -> _
    shift-left: "Gate Range" -> [w209]
    shift-right: [w205] -> _
    shift-left: "Gate Range\nmode" -> [w210]
    shift-right: [w206] -> _
    shift-left: "Gate: Compliance" -> [w218]
    shift-right: [w215] -> _
    shift-left: "Drain: Compliance" -> [w219]
    shift-right: [w216] -> _
    shift-left: w50 -> [w220]
    shift-right: [w72] -> _
    shift-left: w26 -> [w221]
    shift-right: [w73] -> _
    shift-left: w51 -> [w222]
    shift-right: [w217] -> _
    shift-left: w18 -> [w223]
    shift-right: [w80] -> _
    tunnel: "Panel Controls 2" -> [w201]
    shift-right: [w120] -> _
    shift-left: w3 -> [w200]
    shift-right: [w154] -> _
    shift-left: i32[] [] -> [w196]
    tunnel: w31 -> [w195] mode=indexing
    shift-right: [w119] -> _
    shift-left: w3 -> [w172]
    shift-right: [w149] -> _
    shift-left: w23 -> [w159]
    shift-right: [w150] -> _
    shift-left: w21 -> [w152]
    shift-right: [w113] -> _
    shift-left: w3 -> [w141]
    shift-right: [w114] -> _
    shift-left: w3 -> [w140]
    shift-right: [w118] -> _
    shift-left: w3 -> [w129]
    shift-right: [w117] -> _
    shift-left: w3 -> [w128]
    shift-right: [w111] -> _
    shift-left: w3 -> [w127]
    shift-right: [w121] -> _
    shift-left: w3 -> [w126]
    shift-right: [w112] -> _
    shift-left: w3 -> [w125]
    shift-right: [w110] -> _
    shift-left: w3 -> [w124]
    shift-right: [w116] -> _
    shift-left: w3 -> [w123]
    shift-right: [w115] -> _
    shift-left: w3 -> [w122]
    shift-right: [w71] -> _
    shift-left: "Probe 4" -> [w202]
    shift-right: [w76] -> _
    shift-left: w3 -> [w101]
    shift-right: [w77] -> _
    shift-left: w3 -> [w100]
    shift-right: [w78] -> _
    shift-left: w3 -> [w99]
    shift-right: [w79] -> _
    shift-left: w3 -> [w98]
    shift-right: [w68] -> _
    shift-left: w3 -> [w70]
    shift-right: [w67] -> _
    shift-left: w3 -> [w69]
    shift-right: [w64] -> _
    shift-left: w3 -> [w66]
    shift-right: [w63] -> _
    shift-left: w3 -> [w65]
    i -> [w162]
    stop <- "Interrupt program" stop-if-true
    # "Vdg for bias stress plots"
    # "Idg for bias stress plots"
    # "Vp2 for FPP bias stress plots"
    # "Vp1 for FPP bias stress plots"
    # "Ig for bias stress plots"
    # "Id for bias stress plots"
    # "Is for bias stress plots"
    # "Time axis for bias stress plots"
    # "Vdg for bias stress plots"
    # "Idg for bias stress plots"
    # "Vp2 for FPP bias stress plots"
    # "Vp1 for FPP bias stress plots"
    # "Ig for bias stress plots"
    # "Id for bias stress plots"
    # "Is for bias stress plots"
    # "Time axis for bias stress plots"
    # "Save bias stress curves in file."
    # "Is off"
    # "Is on"
    # "Ig off"
    # "Ig on"
    # "Is min"
    # "Is max"
    # "Ig min"
    # "Ig max"
    # "Id min"
    # "Id max"
    # "Id off"
    # "Id on"
    # "Is off"
    # "Is on"
    # "Ig off"
    # "Ig on"
    # "Is min"
    # "Is max"
    # "Ig min"
    # "Ig max"
    # "Id min"
    # "Id max"
    # "Id off"
    # "Id on"
    # "Filepath and name"
    # "Limit of command arguments (array columns). Raise if needed."
    # "Serial port data (string)"
    # "Serial port data (table)"
    # "Serial port data"
    # "For loop counter"
    # "<-----Equivalent to the 4155C \"Write\" subvi.----->"
    # "Headers"
    # "Save transfer curves in file."
    # "Filepath and name"
    # "Save time-dependent data."
    # "Use the time offset if your measurements do not start at t=0."
    # "Time for Imax, Imin, Ion, Ioff"
    # "Rest of elements of command"
    # "First element of command\n(case select)"
    n21 = Add(x=w162, y=1) -> (x+y=→"Line running":i32)
    n22 = Add(x=w167, y=1) -> (x+y=→"Total lines":i32)
    n23 = Index Array(array=w195, index=0 ("line index")) -> (element=w190:string)
    "Command running:" <- w190
    n24 = control-ref of="Interrupt scan"() -> (w214:refnum<vi>)
    n25 = Spreadsheet String To Array(delimiter (Tab)=" ", format string="%s", spreadsheet string=w190, array type (2D Dbl)=string[] []) -> (array=w188:string[])
    n26 = Delete From Array(array=w188, index=0) -> (deleted portion=w142:string, array with subset deleted=w187:string[])  [unwired: 1 in]
    n27 = call "Elapsed Time"("Reset"="Reset", "Auto Reset"="Auto Reset") -> ("Elapsed Time (s)"=w197:dbl)  [unwired: 10 in, 7 out]
    n28 = case shown="2" "Time Units" {
      tunnel: ["-sec" "-min" "-h"] -> w198
      tunnel: [w227 w231 w234] -> w168
      tunnel: w197 -> [w227 w230 w235]
      frame 0, Default {
      }
      frame 1 {
        n29 = Divide(x=w230, y=60.0) -> (x/y=w231:dbl)
      }
      frame 2 {
        n30 = Divide(x=w235, y=3600.0) -> (x/y=w234:dbl)
      }
    }
    n31 = Add(x=w168, y="Time Offset") -> (x+y=w102:dbl)
    n32 = To Long Integer(number=w102) -> (32bit integer=w103:i32)
    "Elapsed Time" <- w103
    n33 = case shown="\"transfer\"" w142 {
      tunnel: w187 -> [w275 w316 w356 w376 w427 w605 w740 w1006 w1142 w1317 w1394 w1443 w1490 w1533 w1569 _ _ w1767 w1918 _ w2039 w2107 w2172 w2293 w2445 w2531]
      tunnel: w223 -> [w270 w312 w354 w389 w486 w612 w804 w1013 w1206 w1334 w1383 w1435 w1483 w1527 w1562 w1603 w1667 w1748 w1902 w1962 w2026 w2094 w2160 w2287 w2441 w2533]
      tunnel: w222 -> [w269 w311 w345 w388 w471 w583 w775 w984 w1176 w1335 w1384 w1436 w1484 w1528 w1563 w1608 w1669 w1773 w1924 w1966 w2045 w2113 w2178 w2299 w2405 w2537]
      tunnel: w221 -> [w268 w310 w344 w387 w470 w582 w774 w983 w1173 w1336 w1385 w1437 w1485 w1529 w1564 w1607 w1640 w1772 w1923 w1965 w2044 w2112 w2177 w2298 w2404 w2536]
      tunnel: w220 -> [w267 w309 w353 w385 w447 w608 w800 w1009 w1202 w1344 w1393 w1434 w1482 w1526 w1561 w1606 w1664 w1740 w1894 w1971 w2019 w2087 w2153 w2286 w2440 w2538]
      tunnel: w219 -> [w266 w308 w352 w384 w484 w610 w802 w1011 w1204 w1343 w1392 w1442 w1489 w1532 w1568 w1605 w1649 w1771 w1922 w1974 w2043 w2111 w2176 w2297 w2449 w2539]
      tunnel: w218 -> [w265 w307 w351 w382 w483 w609 w801 w1010 w1203 w1342 w1391 w1441 w1488 w1531 w1567 w1604 w1650 w1749 w1903 w1973 w2027 w2095 w2161 w2288 w2442 w2541]
      tunnel: [w269 w311 w343 w388 w481 w607 w799 w1008 w1201 w1335 w1384 w1436 w1484 w1528 w1563 w1608 w1669 w1741 w1876 w1964 w2020 w2088 w2154 w2246 w2407 w2537] -> w217
      tunnel: [w268 w310 w342 w387 w480 w606 w798 w1007 w1200 w1336 w1385 w1437 w1485 w1529 w1564 w1607 w1639 w1750 w1877 w1963 w2028 w2096 w2162 w2245 w2406 w2535] -> w153
      tunnel: [w267 w309 w353 w385 w443 w608 w800 w1009 w1202 w1337 w1386 w1434 w1482 w1526 w1561 w1606 w1664 w1740 w1894 w1971 w2019 w2087 w2153 w2286 w2440 w2538] -> w72
      tunnel: [w266 w308 w352 w384 w484 w610 w802 w1011 w1204 w1343 w1392 w1442 w1489 w1532 w1568 w1605 w1649 w1771 w1922 w1974 w2043 w2111 w2176 w2297 w2449 w2539] -> w216
      tunnel: [w265 w307 w351 w382 w483 w609 w801 w1010 w1203 w1342 w1391 w1441 w1488 w1531 w1567 w1604 w1650 w1749 w1903 w1973 w2027 w2095 w2161 w2288 w2442 w2541] -> w215
      tunnel: [w270 w312 w354 w389 w486 w612 w804 w1013 w1206 w1334 w1383 w1435 w1483 w1527 w1562 w1603 w1667 w1748 w1902 w1962 w2026 w2094 w2160 w2287 w2441 w2533] -> w80
      tunnel: w214 -> [_ _ _ _ w490 w614 w808 w1015 w1210 _ _ _ _ _ _ _ _ w1745 w1899 _ w2025 w2093 w2159 w2265 w2423 _]
      tunnel: "Gate" -> [_ _ _ _ w474 w592 w785 w993 w1187 _ _ _ _ _ _ _ _ _ _ _ _ _ _ _ _ _]
      tunnel: "Drain 2" -> [_ _ _ _ w473 w591 w784 w992 w1186 _ _ _ _ _ _ _ _ _ _ _ _ _ _ _ _ _]
      tunnel: "Panel Controls" -> [_ _ _ _ _ _ w783 w919 w1185 _ _ _ _ _ _ _ _ _ _ _ _ _ _ _ _ _]
      tunnel: w210 -> [w264 w306 w350 w381 w464 w576 w768 w977 w1171 w1341 w1390 _ w1481 w1525 w1560 w1602 w1651 w1736 w1890 w1967 w2015 w2083 w2149 w2282 w2436 w2542]
      tunnel: w209 -> [w263 w305 w349 w380 w463 w575 w767 w976 w1170 w1340 w1389 w1440 _ w1516 w1566 w1601 w1652 w1737 w1891 w1968 w2016 w2084 w2150 w2283 w2437 w2543]
      tunnel: w208 -> [w262 w304 w348 w379 w462 w574 w766 w975 w1169 w1339 w1388 w1439 w1487 w1530 _ w1600 w1653 w1738 w1892 w1969 w2017 w2085 w2151 w2284 w2438 w2544]
      tunnel: w207 -> [w261 w303 w347 w378 w461 w573 w765 w974 w1172 w1338 w1387 w1438 w1486 _ w1565 w1599 w1654 w1739 w1893 w1970 w2018 w2086 w2152 w2285 w2439 w2545]
      tunnel: [w264 w306 w350 w381 w464 w576 w768 w977 w1171 w1341 w1390 w1433 w1481 w1525 w1560 w1602 w1651 w1736 w1890 w1967 w2015 w2083 w2149 w2282 w2436 w2542] -> w206
      tunnel: [w263 w305 w349 w380 w463 w575 w767 w976 w1170 w1340 w1389 w1440 w1473 w1516 w1566 w1601 w1652 w1737 w1891 w1968 w2016 w2084 w2150 w2283 w2437 w2543] -> w205
      tunnel: [w262 w304 w348 w379 w462 w574 w766 w975 w1169 w1339 w1388 w1439 w1487 w1530 w1559 w1600 w1653 w1738 w1892 w1969 w2017 w2085 w2151 w2284 w2438 w2544] -> w204
      tunnel: [w261 w303 w347 w378 w461 w573 w765 w974 w1172 w1338 w1387 w1438 w1486 w1517 w1565 w1599 w1654 w1739 w1893 w1970 w2018 w2086 w2152 w2285 w2439 w2545] -> w203
      tunnel: w202 -> [w245 w284 w325 _ w416 w514 w753 w915 w1159 w1314 w1366 w1417 w1457 w1500 w1543 w1583 w1617 w1723 w1857 w1946 w1986 w2058 w2125 w2232 w2389 w2502]
      tunnel: w201 -> [_ _ _ _ w458 w567 _ _ _ _ _ _ _ _ _ _ _ _ _ _ _ _ _ _ _ _]
      tunnel: [w260 w299 w340 w393 w435 w529 w725 w931 w1125 w1333 w1381 w1432 w1472 w1515 w1558 w1598 w1635 w1713 w1861 w1961 w2004 w2076 w2143 w2207 w2368 w2534] -> w120
      tunnel: w200 -> [w260 w299 w340 w393 w435 w564 w701 w966 w1137 w1333 w1381 w1432 w1472 w1515 w1558 w1598 w1635 w1719 w1861 w1961 w2004 w2076 w2143 w2213 w2374 w2534]
      tunnel: w102 -> [_ _ _ _ w432 w563 w758 w965 w1163 _ _ _ _ _ _ _ w1633 w1728 w1873 _ w2001 w2073 w2140 w2242 w2398 _]
      tunnel: w198 -> [_ _ _ _ w431 w560 w756 w962 w1162 _ _ _ _ _ _ _ w1631 w1726 w1872 _ w2000 w2072 w2139 w2241 w2399 _]
      tunnel: w103 -> [_ _ _ _ _ w556 w741 w958 w1145 _ _ _ _ _ _ _ _ _ _ _ _ _ _ _ _ _]
      tunnel: [w259 w298 w339 w383 w434 w533 w705 w935 w1104 w1332 w1380 w1431 w1471 w1514 w1557 w1597 w1634 w1698 w1845 w1960 w2003 w2075 w2142 w2201 w2363 w2540] -> w154
      tunnel: w196 -> [w259 w298 w339 w383 w434 w559 w742 w961 w1144 w1332 w1380 w1431 w1471 w1514 w1557 w1597 w1634 w1700 w1846 w1960 w2003 w2075 w2142 w2202 w2365 w2540]
      tunnel: [w258 w297 w338 w392 w430 w528 w726 w930 w1126 w1331 w1379 w1430 w1470 w1513 w1556 w1596 w1630 w1712 w1860 w1959 w1999 w2071 w2138 w2206 w2367 w2529] -> w119
      tunnel: w172 -> [w258 w297 w338 w392 w430 w555 w731 w957 w1138 w1331 w1379 w1430 w1470 w1513 w1556 w1596 w1630 w1718 w1860 w1959 w1999 w2071 w2138 w2212 w2373 w2529]
      tunnel: [w257 w296 w337 w377 w429 w548 w755 w950 w1161 w1330 w1378 w1429 w1469 w1512 w1555 w1595 w1629 w1725 w1871 w1958 w1998 w2070 w2137 w2240 w2397 w2528] -> w149
      tunnel: w159 -> [w257 w296 w337 w377 w429 w548 w755 w950 w1161 w1330 w1378 w1429 w1469 w1512 w1555 w1595 w1629 w1725 w1871 w1958 w1998 w2070 w2137 w2240 w2397 w2527]
      tunnel: [w256 w295 w336 w386 w428 w547 w754 w949 w1160 w1329 w1377 w1428 w1468 w1511 w1554 w1594 w1628 w1724 w1870 w1957 w1997 w2069 w2136 w2239 w2396 w2513] -> w150
      tunnel: w152 -> [w256 w295 w336 w386 w428 w547 w754 w949 w1160 w1329 w1377 w1428 w1468 w1511 w1554 w1594 w1628 w1724 w1870 w1957 w1997 w2069 w2136 w2239 w2396 w2513]
      tunnel: [w254 w293 w334 w398 w425 w522 w717 w924 w1120 w1327 w1376 w1427 w1466 w1509 w1552 w1592 w1626 w1706 w1869 w1956 w1996 w2068 w2134 w2238 w2395 w2512] -> w113
      tunnel: w141 -> [w254 w293 w334 w398 w425 w546 w736 w948 w1132 w1327 w1376 w1427 w1466 w1509 w1552 w1592 w1626 w1706 w1869 w1956 w1996 w2068 w2134 w2238 w2395 w2512]
      tunnel: [w255 w294 w335 w399 w426 w523 w718 w925 w1119 w1328 w1375 w1426 w1467 w1510 w1553 w1593 w1627 w1707 w1868 w1955 w1995 w2067 w2135 w2237 w2394 w2511] -> w114
      tunnel: w140 -> [w255 w294 w335 w399 w426 w545 w737 w947 w1131 w1328 w1375 w1426 w1467 w1510 w1553 w1593 w1627 w1707 w1868 w1955 w1995 w2067 w2135 w2237 w2394 w2511]
      tunnel: [w247 w286 w327 w391 w422 w527 w727 w929 w1127 w1320 w1373 w1424 w1464 w1507 w1550 w1590 w1619 w1711 w1859 w1954 w1988 w2060 w2127 w2205 w2370 w2504] -> w118
      tunnel: w129 -> [w247 w286 w327 w391 w422 w541 w732 w943 w1139 w1320 w1373 w1424 w1464 w1507 w1550 w1590 w1619 w1717 w1859 w1954 w1988 w2060 w2127 w2211 w2372 w2504]
      tunnel: [w246 w285 w326 w390 w423 w526 w728 w928 w1128 w1319 w1374 w1425 w1465 w1508 w1551 w1591 w1618 w1710 w1858 w1953 w1987 w2059 w2126 w2204 w2369 w2503] -> w117
      tunnel: w128 -> [w246 w285 w326 w390 w423 w540 w733 w942 w1140 w1319 w1374 w1425 w1465 w1508 w1551 w1591 w1618 w1716 w1858 w1953 w1987 w2059 w2126 w2210 w2371 w2503]
      tunnel: [w249 w288 w329 w395 w421 w532 w723 w934 w1123 w1325 w1371 w1422 w1462 w1505 w1548 w1588 w1621 w1715 w1863 w1948 w1990 w2062 w2129 w2209 w2376 w2508] -> w111
      tunnel: w127 -> [w249 w288 w329 w395 w421 w539 w729 w941 w1135 w1325 w1371 w1422 w1462 w1505 w1548 w1588 w1621 w1721 w1863 w1948 w1990 w2062 w2129 w2215 w2378 w2508]
      tunnel: [w248 w287 w328 w394 w424 w530 w724 w932 w1124 w1326 w1372 w1423 w1463 w1506 w1549 w1589 w1620 w1714 w1862 w1947 w1989 w2061 w2128 w2208 w2366 w2507] -> w121
      tunnel: w126 -> [w248 w287 w328 w394 w424 w538 w730 w940 w1136 w1326 w1372 w1423 w1463 w1506 w1549 w1589 w1620 w1720 w1862 w1947 w1989 w2061 w2128 w2214 w2375 w2507]
      tunnel: [w251 w290 w331 w397 w420 w521 w721 w923 w1121 w1323 w1369 w1420 w1460 w1503 w1546 w1586 w1623 w1705 w1865 w1950 w1992 w2064 w2131 w2234 w2391 w2510] -> w112
      tunnel: w125 -> [w251 w290 w331 w397 w420 w537 w735 w939 w1133 w1323 w1369 w1420 w1460 w1503 w1546 w1586 w1623 w1705 w1865 w1950 w1992 w2064 w2131 w2234 w2391 w2510]
      tunnel: [w250 w289 w330 w396 w419 w520 w722 w922 w1122 w1324 w1370 w1421 w1461 w1504 w1547 w1587 w1622 w1704 w1864 w1949 w1991 w2063 w2130 w2233 w2390 w2509] -> w110
      tunnel: w124 -> [w250 w289 w330 w396 w419 w536 w734 w938 w1134 w1324 w1370 w1421 w1461 w1504 w1547 w1587 w1622 w1704 w1864 w1949 w1991 w2063 w2130 w2233 w2390 w2509]
      tunnel: [w253 w292 w333 w401 w418 w525 w720 w927 w1117 w1321 w1367 w1418 w1458 w1501 w1544 w1584 w1625 w1709 w1867 w1952 w1994 w2066 w2133 w2236 w2393 w2506] -> w116
      tunnel: w123 -> [w253 w292 w333 w401 w418 w535 w739 w937 w1129 w1321 w1367 w1418 w1458 w1501 w1544 w1584 w1625 w1709 w1867 w1952 w1994 w2066 w2133 w2236 w2393 w2506]
      tunnel: [w252 w291 w332 w400 w417 w524 w719 w926 w1118 w1322 w1368 w1419 w1459 w1502 w1545 w1585 w1624 w1708 w1866 w1951 w1993 w2065 w2132 w2235 w2392 w2505] -> w115
      tunnel: w122 -> [w252 w291 w332 w400 w417 w534 w738 w936 w1130 w1322 w1368 w1419 w1459 w1502 w1545 w1585 w1624 w1708 w1866 w1951 w1993 w2065 w2132 w2235 w2392 w2505]
      tunnel: [w245 w284 w325 w367 w416 w514 w753 w915 w1159 w1314 w1366 w1417 w1457 w1500 w1543 w1583 w1617 w1723 w1857 w1946 w1986 w2058 w2125 w2232 w2389 w2502] -> w71
      tunnel: w102 -> [_ _ _ _ _ _ _ _ _ _ _ _ _ _ _ _ _ w1675 w1841 _ _ _ _ w2216 w2382 _]
      tunnel: [w244 w283 w324 w366 w415 w513 w712 w914 w1110 w1313 w1365 w1416 w1456 w1499 w1542 w1582 w1616 w1687 w1856 w1945 w1985 w2057 w2124 w2222 w2385 w2501] -> w76
      tunnel: [w243 w282 w323 w365 w414 w512 w713 w913 w1111 w1312 w1364 w1415 w1455 w1498 w1541 w1581 w1615 w1684 w1855 w1944 w1984 w2056 w2123 w2183 w2346 w2500] -> w77
      tunnel: [w242 w281 w322 w364 w413 w511 w714 w912 w1112 w1311 w1363 w1414 w1454 w1497 w1540 w1580 w1614 w1685 w1828 w1943 w1983 w2055 w2122 w2195 w2358 w2499] -> w78
      tunnel: [w241 w280 w321 w363 w412 w510 w715 w911 w1113 w1310 w1362 w1413 w1453 w1496 w1539 w1579 w1613 w1686 w1835 w1942 w1982 w2054 w2121 w2191 w2354 w2498] -> w79
      tunnel: w101 -> [w244 w283 w324 w366 w415 w513 w712 w914 w1110 w1313 w1365 w1416 w1456 w1499 w1542 w1582 w1616 w1691 w1856 w1945 w1985 w2057 w2124 w2225 w2388 w2501]
      tunnel: w100 -> [w243 w282 w323 w365 w414 w512 w713 w913 w1111 w1312 w1364 w1415 w1455 w1498 w1541 w1581 w1615 w1690 w1855 w1944 w1984 w2056 w2123 w2224 w2387 w2500]
      tunnel: w99 -> [w242 w281 w322 w364 w413 w511 w714 w912 w1112 w1311 w1363 w1414 w1454 w1497 w1540 w1580 w1614 w1689 w1829 w1943 w1983 w2055 w2122 w2195 w2358 w2499]
      tunnel: w98 -> [w241 w280 w321 w363 w412 w510 w715 w911 w1113 w1310 w1362 w1413 w1453 w1496 w1539 w1579 w1613 w1688 w1837 w1942 w1982 w2054 w2121 w2223 w2386 w2498]
      tunnel: "Standby" -> [_ _ _ _ w411 w509 _ w910 _ _ _ _ _ _ _ _ _ w1682 w1854 _ _ _ _ w2231 _ _]
      tunnel: w70 -> [w240 w279 w320 w362 w405 w504 w710 w904 w1108 w1309 w1361 w1412 w1452 w1495 w1538 w1578 w1612 w1673 w1849 w1941 w1978 w2051 w2119 w2189 w2352 w2497]
      tunnel: w69 -> [w239 w278 w319 w361 w404 w503 w711 w905 w1109 w1308 w1360 w1411 w1451 w1494 w1537 w1577 w1611 w1672 w1848 w1940 w1977 w2050 w2118 w2188 w2351 w2496]
      tunnel: [w240 w279 w320 w362 w405 w504 w710 w904 w1108 w1309 w1361 w1412 w1452 w1495 w1538 w1578 w1612 w1673 w1849 w1941 w1978 w2051 w2119 w2184 w2347 w2497] -> w68
      tunnel: [w239 w278 w319 w361 w404 w503 w711 w905 w1109 w1308 w1360 w1411 w1451 w1494 w1537 w1577 w1611 w1672 w1848 w1940 w1977 w2050 w2118 w2187 w2350 w2496] -> w67
      tunnel: w66 -> [w238 w277 w318 w360 w402 w501 w708 w902 w1106 w1306 w1358 w1409 w1449 w1492 w1535 w1575 w1609 w1671 w1834 w1939 w1976 w2049 w2117 w2182 w2345 w2495]
      tunnel: w65 -> [w237 w276 w317 w359 w403 w502 w709 w903 w1107 w1307 w1359 w1410 w1450 w1493 w1536 w1576 w1610 w1670 w1833 w1938 w1975 w2048 w2116 w2181 w2344 w2494]
      tunnel: [w238 w277 w318 w360 w402 w501 w708 w902 w1106 w1306 w1358 w1409 w1449 w1492 w1535 w1575 w1609 w1671 w1826 w1939 w1976 w2049 w2117 w2182 w2345 w2495] -> w64
      tunnel: [w237 w276 w317 w359 w403 w502 w709 w903 w1107 w1307 w1359 w1410 w1450 w1493 w1536 w1576 w1610 w1670 w1832 w1938 w1975 w2048 w2116 w2181 w2344 w2494] -> w63
      frame "wait" {
        n34 = Index Array(array=w275, index=0 ("Index")) -> (element=w273:string)
        n35 = Decimal String To Number(string=w273, default (0L)=u32 0) -> (number=w272:u32)  [unwired: 1 in, 1 out]
        n36 = Wait (ms)(milliseconds to wait=w272) -> ()  [unwired: 1 out]
      }
      frame "wait-min" {
        n37 = Index Array(array=w316, index=0 ("Index")) -> (element=w314:string)
        n38 = Decimal String To Number(string=w314, default (0L)=u32 0) -> (number=w302:u32)  [unwired: 1 in, 1 out]
        n39 = Multiply(x=w302, y=u32 60000) -> (x*y=w301:u32)
        n40 = Wait (ms)(milliseconds to wait=w301) -> ()  [unwired: 1 out]
      }
      frame "standby" {
        n41 = Index Array(array=w356, index=0 ("Index")) -> (element=w346:string)
        n42 = case shown="\"off\", Default" w346 {
          tunnel: [":PAGE:SCON:STAN 0" ":PAGE:SCON:STAN 1"] -> w341
          frame "off", Default {
          }
          frame "on" {
          }
        }
        n43 = VISA Write(VISA resource name=w345, write buffer=w341, error in (no error)=w344) -> (VISA resource name out=w343:refnum<visa-resource-name>, error out=w342:errorcluster)  [unwired: 1 out]
      }
      frame "Probe4" {
        n44 = Delete From Array(array=w376, index=0) -> (deleted portion=w370:string, array with subset deleted=w373:string[])  [unwired: 1 in]
        n45 = Equal?(x=w370, y="ON") -> (x = y?=w368:bool)
        n46 = Delete From Array(array=w373, index=0) -> (deleted portion=w372:string)  [unwired: 1 in, 1 out]
        n47 = Fract/Exp String To Number(string=w372) -> (number=w369:dbl)  [unwired: 3 in, 1 out]
        n48 = Bundle(w368, w369) -> (w367:cluster{bool, dbl})  [unwired: 1 in]
      }
      frame "pulsedstressV" {
        w441 = 0
        n49 = local read "Pulsed Stress V - Vextra"() -> (w408:u32)
        n50 = local read "Pulsed Stress V - Drain"() -> (w410:u32)
        n51 = local read "Pulsed Stress V - Gate"() -> (w407:u32)
        n52 = local read "Pulsed Stress V - Probe 4"() -> (w409:u32)
        n53 = local read "Pulsed Stress V - Source/Common"() -> (w406:u32)
        n54 = Number To Decimal String(number=w432) -> (decimal integer string=w487:string)  [unwired: 1 in]
        n55 = Delete From Array(array=w427, index=0 ("Index")) -> (deleted portion=w478:string, array with subset deleted=w477:string[])  [unwired: 1 in]
        n56 = Bundle By Name(cluster=w458, "Emergency Stop"=w490) -> (w459:T2)
        n57 = VISA Write(VISA resource name=w471, write buffer=":PAGE:CHAN:MODE SWE;" ("write buffer (\"\")"), error in (no error)=w470) -> (VISA resource name out=w468:refnum<visa-resource-name>, error out=w469:errorcluster)  [unwired: 1 out]
        n58 = Concatenate Strings(w486, "-pulsedstressV-" ("Substring"), w487, w431, ".txt" ("Substring")) -> (w489:string)
        n59 = case shown="\"d\", Default" w478 {
          tunnel: [w499 w500] -> w476
          frame "s" {
            w499 = u16 0 items=["Single", "Double"] ("sweep mode")
          }
          frame "d", Default {
            w500 = u16 1 items=["Single", "Double"] ("sweep mode")
          }
        }
        n60 = Fract/Exp String To Number(string=w477) -> (number=w472:dbl[])  [unwired: 3 in, 1 out]
        n61 = String To Path(string=w489) -> (path=w485:path)
        n62 = Index Array(array=w472, index #1=0 ("Index")) -> (element #1=w450:dbl, element #2=w449:dbl, element #3=w446:dbl, element #4=w445:dbl, element #5=w444:dbl, element #6=w448:dbl)  [unwired: 5 in]
        n63 = Bundle By Name(cluster=w447, "Pulse period"=w445, "Base voltage"=w446, "Pulse width"=w444) -> (w443:T4)
        n64 = Unbundle By Name(w443) -> ("Pulse period"=w451:dbl)
        n65 = Bundle By Name(cluster=w474, "Gate Start"=w449, "Gate Stop"=w450, "Gate Step (linear only)"=0, "Gate Compliance"=w483, "Range mode"=w464, "Range"=w463) -> (w465:T6)
        n66 = call <vilib>:"compatOverwrite.vi"("overwrite (F)"=TRUE) -> ("overwrite?"=w436:T8)
        n67 = Bundle By Name(cluster=w473, "Drain Start"=w448, "Drain Stop"=w441, "Drain Step"=w441, "Drain Compliance"=w484, "Range mode"=w462, "Range"=w461) -> (w466:T7)
        n68 = call "4155C PulsedStressV v3.0.vi"("VISA resource name in"=w468, "Gate"=w465, "Pulsed Stress V - Source/Common"=w406, "Drain"=w466, "Timings"=w443, "error in (no error)"=w469, "sweep mode"=w476, "Probe 4"=w416, "Pulsed Stress V - Drain"=w410, "Pulsed Stress V - Gate"=w407, "Panel Controls"=w459, "Standby"=w411, "Pulsed Stress V - Probe 4"=w409, "Pulsed Stress V - Vextra"=w408) -> ("Outparams"=w460:T9, "VISA Resource Name out"=w481:refnum<visa-resource-name>, "ID"=w439:dbl[], "IG"=w437:dbl[], "error out"=w482:errorcluster)  [unwired: 1 in]
        n69 = Unbundle By Name(w460) -> ("Number of points"=w438:i32)  [unwired: 2 out]
        n70 = for {
          N: w438 -> [_]
          tunnel: [w496] -> w440 mode=indexing
          tunnel: w451 -> [w498]
          i -> [w497]
          n71 = Multiply(x=w498, y=w497) -> (x*y=w496:dbl)
        }
        n72 = Insert Into Array(array=dbl[][] [] ("Input Array"), new element=w440) -> (w452:dbl[][])  [unwired: 2 in]
        n73 = Insert Into Array(array=w452, new element=w439) -> (w457:dbl[][])  [unwired: 2 in]
        n74 = Insert Into Array(array=w457, new element=w437) -> (w456:dbl[][])  [unwired: 2 in]
        n75 = Transpose 2D Array(2D array=w456) -> (transposed array=w455:dbl[][])
        n76 = Open/Create/Replace File(file path (use dialog)=w485, error in=w482, operation (0:open)=w436) -> (refnum out=w493:refnum<file>, error out=w494:errorcluster)  [unwired: 3 in, 1 out]
        n77 = call "4155C Write array to file.vi"("Byte Stream File Refnum"=w493, "Header"=string[] ["Time /s", "Id /A", "Ig /A"], "Data Array"=w455, "error in (no error)"=w494) -> ("dup refnum"=w491:refnum<file>, "error out"=w492:errorcluster)  [unwired: 1 in]
        n78 = Close File(refnum=w491, error in=w492) -> (error out=w480:errorcluster)  [unwired: 1 out]
      }
      frame "transfer" {
        n79 = local read "Transfer/Output - Gate"() -> (w508:u32)
        n80 = Delete From Array(array=w605, index=0 ("Index")) -> (deleted portion=w603:string, array with subset deleted=w602:string[])  [unwired: 1 in]
        n81 = Bundle By Name(cluster=w567, "Emergency Stop"=w614) -> (w568:T2)
        n82 = Number To Decimal String(number=w563) -> (decimal integer string=w562:string)  [unwired: 1 in]
        n83 = case shown="\"d\", Default" w603 {
          tunnel: [w699 w700] -> w601
          frame "s" {
            w699 = u16 0 items=["Single", "Double"] ("sweep mode")
          }
          frame "d", Default {
            w700 = u16 1 items=["Single", "Double"] ("sweep mode")
          }
        }
        n84 = Fract/Exp String To Number(string=w602) -> (number=w587:dbl[])  [unwired: 3 in, 1 out]
        n85 = Concatenate Strings(w612, "-transfer-" ("Prefix"), w562, w560, ".txt" ("Suffix (transfer)")) -> (w613:string)
        n86 = VISA Write(VISA resource name=w583, write buffer=":PAGE:CHAN:MODE SWE;" ("write buffer (\"\")"), error in (no error)=w582) -> (VISA resource name out=w580:refnum<visa-resource-name>, error out=w581:errorcluster)  [unwired: 1 out]
        n87 = local read "Plot transfer curve extrema vs time"() -> (w515:bool)
        n88 = String To Path(string=w613) -> (path=w611:path)
        n89 = Index Array(array=w587, index #1=0 ("Index")) -> (element #1=w600:dbl, element #2=w599:dbl, element #3=w598:dbl)  [unwired: 2 in]
        n90 = Delete From Array(array=w587, length=3 ("Length"), index=0 ("Index")) -> (array with subset deleted=w585:dbl[])  [unwired: 1 out]
        n91 = local read "Transfer/Output - Drain"() -> (w505:u32)
        n92 = local read "Transfer/Output - Source/Common"() -> (w507:u32)
        n93 = case shown="True" w515 {
          tunnel: w559 -> [w616 w619]
          tunnel: w556 -> [_ w618]
          tunnel: [w616 w617] -> w533
          frame False {
          }
          frame True {
            n94 = Build Array (concatenate)(w619, w618) -> (w617:i32[])
          }
        }
        n95 = local read "Transfer/Output - Probe 4"() -> (w506:u32)
        n96 = Bundle By Name(cluster=w592, "Gate Start"=w600, "Gate Stop"=w599, "Gate Step (linear only)"=w598, "Gate Compliance"=w609, "Range mode"=w576, "Range"=w575) -> (w577:T6)
        n97 = Index Array(array=w585, index #1=0 ("Index")) -> (element #1=w595:dbl, element #2=w594:dbl, element #3=w593:dbl)  [unwired: 2 in]
        n98 = call <vilib>:"compatOverwrite.vi"("overwrite (F)"=TRUE) -> ("overwrite?"=w566:T8)
        n99 = Bundle By Name(cluster=w591, "Drain Start"=w595, "Drain Stop"=w594, "Drain Step"=w593, "Drain Compliance"=w610, "Range mode"=w574, "Range"=w573) -> (w578:T7)
        n100 = call "4155C Transfer v3.0.vi"("VISA resource name in"=w580, "Source/Common"=w507, 2:"Gate"=w577, 3:"Drain"=w578, 4:"Drain"=w505, "Timings"=w608, "error in (no error)"=w581, 7:"Probe 4"=w514, 8:"Gate"=w508, 9:"Probe 4"=w506, "sweep mode"=w601, "Panel Controls"=w568, "Standby"=w509) -> ("VG"=w565:dbl[], "Outparams"=w572:T9, "VISA Resource Name out"=w607:refnum<visa-resource-name>, "IS"=w543:dbl[], "ID"=w544:dbl[], "IG"=w542:dbl[], "error out"=w557:errorcluster, "Probe 4"=w569:dbl[])  [unwired: 7 in]
        n101 = Unbundle By Name(w572) -> ("V2 Step"=w571:dbl, "V2 Start"=w570:dbl, "Number of points"=w531:i32)
        n102 = call "4155C Split array.vi"("Number of VAR2 steps"=w531, "Y2 data in"=w544, "X data in"=w565, "Y1 data in"=w543, "Y3 data in"=w542, "error in (no error)"=w557) -> ("Array of clusters"=w558:cluster{"Y data in":dbl[], "X data in":dbl[]}[], "error out"=w519:errorcluster)  [unwired: 1 in]
        n103 = case shown="True" "Plot transfer curve extrema vs time" {
          tunnel: w564 -> [w622 w698]
          tunnel: w555 -> [w623 w693]
          tunnel: w546 -> [w629 w689]
          tunnel: w545 -> [w630 w688]
          tunnel: w544 -> [_ w685]
          tunnel: w543 -> [_ w683]
          tunnel: w542 -> [_ w682]
          tunnel: w541 -> [w624 w678]
          tunnel: w540 -> [w626 w677]
          tunnel: w539 -> [w620 w674]
          tunnel: w538 -> [w621 w673]
          tunnel: w537 -> [w628 w670]
          tunnel: w536 -> [w627 w669]
          tunnel: w535 -> [w632 w666]
          tunnel: w534 -> [w631 w665]
          tunnel: w533 -> [_ w658]
          tunnel: [w620 w653] -> w532
          tunnel: w531 -> [_ w652]
          tunnel: [w621 w651] -> w530
          tunnel: [w622 w650] -> w529
          tunnel: [w623 w649] -> w528
          tunnel: [w624 w648] -> w527
          tunnel: [w626 w647] -> w526
          tunnel: [w632 w646] -> w525
          tunnel: [w631 w645] -> w524
          tunnel: [w630 w644] -> w523
          tunnel: [w629 w643] -> w522
          tunnel: [w628 w642] -> w521
          tunnel: [w627 w641] -> w520
          tunnel: w519 -> [w625 w640]
          tunnel: [w625 w636] -> w518
          frame False {
          }
          frame True {
            # "Adjusts graph colors."
            # "Adjusts graph colors."
            # "Ion will be the middle element of the array. The calculation of the index is done only once, since Is, Id, and Ig have the same dimensions."
            # "abs(Ig)"
            # "abs(Is)"
            # "Y1: Is\nY2: Id\nY3: Ig"
            # "abs(Id)"
            # "Adjusts graph colors."
            # "Adjusts graph colors."
            # "Adjusts graph colors."
            n104 = Absolute Value(x=w683) -> (abs(x)=w668:dbl[])
            n105 = Absolute Value(x=w685) -> (abs(x)=w684:dbl[])
            n106 = Absolute Value(x=w682) -> (abs(x)=w671:dbl[])
            n107 = Array Size(array=w684) -> (size(s)=w692:i32)
            n108 = Divide(x=w692, y=2) -> (x/y=w635:dbl)
            n109 = Subtract(x=w635, y=1) -> (x-y=w634:dbl)
            n110 = Array Max & Min(array=w668) -> (max value=w675:dbl, min value=w676:dbl)  [unwired: 2 out]
            n111 = Array Max & Min(array=w684) -> (max value=w697:dbl, min value=w681:dbl)  [unwired: 2 out]
            n112 = Array Max & Min(array=w671) -> (max value=w680:dbl, min value=w679:dbl)  [unwired: 2 out]
            n113 = Index Array(array=w668, index=w634) -> (element=w659:dbl)
            n114 = Index Array(array=w668, index=0) -> (element=w660:dbl)
            n115 = Index Array(array=w684, index=w634) -> (element=w661:dbl)
            n116 = Index Array(array=w684, index=0) -> (element=w662:dbl)
            n117 = Index Array(array=w671, index=w634) -> (element=w664:dbl)
            n118 = Index Array(array=w671, index=0) -> (element=w663:dbl)
            n119 = local write "Ig max"(w680) -> ()
            n120 = local write "Ig min"(w679) -> ()
            n121 = local write "Is max"(w675) -> ()
            n122 = local write "Is min"(w676) -> ()
            n123 = local write "Id max"(w697) -> ()
            n124 = local write "Id min"(w681) -> ()
            n125 = Build Array (concatenate)(w674, w675) -> (w653:dbl[])
            n126 = Build Array (concatenate)(w673, w676) -> (w651:dbl[])
            n127 = local write "Is off"(w660) -> ()
            n128 = local write "Is on"(w659) -> ()
            n129 = Build Array (concatenate)(w698, w697) -> (w650:dbl[])
            n130 = Build Array (concatenate)(w693, w681) -> (w649:dbl[])
            n131 = Build Array (concatenate)(w678, w680) -> (w648:dbl[])
            n132 = Build Array (concatenate)(w677, w679) -> (w647:dbl[])
            n133 = Build Array (concatenate)(w666, w659) -> (w646:dbl[])
            n134 = Build Array (concatenate)(w665, w660) -> (w645:dbl[])
            n135 = Build Array (concatenate)(w688, w661) -> (w644:dbl[])
            n136 = Build Array (concatenate)(w689, w662) -> (w643:dbl[])
            n137 = Build Array (concatenate)(w670, w664) -> (w642:dbl[])
            n138 = Build Array (concatenate)(w669, w663) -> (w641:dbl[])
            n139 = local write "Ig off"(w663) -> ()
            n140 = local write "Ig on"(w664) -> ()
            n141 = local write "Id off"(w662) -> ()
            n142 = local write "Id on"(w661) -> ()
            n143 = control-ref of="Imax vs time"() -> (w687:refnum<vi>)
            n144 = control-ref of="Imin vs time"() -> (w686:refnum<vi>)
            n145 = control-ref of="Ion vs time"() -> (w655:refnum<vi>)
            n146 = control-ref of="Ioff vs time"() -> (w654:refnum<vi>)
            n147 = control-ref of="I vs Vg"() -> (w696:refnum<vi>)
            n148 = call "4155C Split array.vi"("Number of VAR2 steps"=w652, "Y2 data in"=w644, "X data in"=w658, "Y1 data in"=w646, "Y3 data in"=w642, "error in (no error)"=w640) -> ("Array of clusters"=w656:cluster{"Y data in":dbl[], "X data in":dbl[]}[], "error out"=w639:errorcluster)  [unwired: 1 in]
            n149 = call "4155C Split array.vi"("Number of VAR2 steps"=w652, "Y2 data in"=w643, "X data in"=w658, "Y1 data in"=w645, "Y3 data in"=w641, "error in (no error)"=w639) -> ("Array of clusters"=w657:cluster{"Y data in":dbl[], "X data in":dbl[]}[], "error out"=w638:errorcluster)  [unwired: 1 in]
            n150 = call "4155C Split array.vi"("Number of VAR2 steps"=w652, "Y2 data in"=w650, "X data in"=w658, "Y1 data in"=w653, "Y3 data in"=w648, "error in (no error)"=w638) -> ("Array of clusters"=w695:cluster{"Y data in":dbl[], "X data in":dbl[]}[], "error out"=w637:errorcluster)  [unwired: 1 in]
            n151 = call "4155C Split array.vi"("Number of VAR2 steps"=w652, "Y2 data in"=w649, "X data in"=w658, "Y1 data in"=w651, "Y3 data in"=w647, "error in (no error)"=w637) -> ("Array of clusters"=w694:cluster{"Y data in":dbl[], "X data in":dbl[]}[], "error out"=w636:errorcluster)  [unwired: 1 in]
            n152 = call "4155C Config Chart Colours.vi"("Numeric"=w652, "XY Graph 2"=w687) -> ()  [unwired: 6 in]
            n153 = call "4155C Config Chart Colours.vi"("Numeric"=w652, "XY Graph 2"=w686) -> ()  [unwired: 6 in]
            n154 = call "4155C Config Chart Colours.vi"("Numeric"=w652, "XY Graph 2"=w655) -> ()  [unwired: 6 in]
            n155 = call "4155C Config Chart Colours.vi"("Numeric"=w652, "XY Graph 2"=w654) -> ()  [unwired: 6 in]
            n156 = call "4155C Config Chart Colours.vi"("Numeric"=w652, "XY Graph 2"=w696) -> ()  [unwired: 6 in]
            n157 = local write "Imax vs time"(w695) -> ()
            n158 = local write "Imin vs time"(w694) -> ()
            n159 = local write "Ion vs time"(w656) -> ()
            n160 = local write "Ioff vs time"(w657) -> ()
          }
        }
        n161 = local write "I vs Vg"(w558) -> ()
        n162 = Open/Create/Replace File(file path (use dialog)=w611, error in=w518, operation (0:open)=w566) -> (refnum out=w553:refnum<file>, error out=w551:errorcluster)  [unwired: 3 in, 1 out]
        n163 = call "4155C Make Big 2d array.vi"("1D Var1"=w565, "1d IS"=w543, "1d ID"=w544, "1d IG"=w542, "1d SMU4"=w569, "SMU4"=w514, "VAR2 START"=w570, "Number of VAR2 steps"=w531, "VAR2 STEP"=w571, "VAR1 Name"="Vg", "Decimal places in header"=i8 1, "VAR2 Name"="Vd") -> ("Header array"=w554:string[], "Data array"=w552:dbl[][])  [unwired: 14 in]
        n164 = call "4155C Write array to file.vi"("Byte Stream File Refnum"=w553, "Header"=w554, "Data Array"=w552, "error in (no error)"=w551) -> ("dup refnum"=w550:refnum<file>, "error out"=w549:errorcluster)  [unwired: 1 in]
        n165 = Close File(refnum=w550, error in=w549) -> (error out=w606:errorcluster)  [unwired: 1 out]
      }
      frame "transfer-fpp" {
        # "Adjusts graph colors."
        # "Y1 = Y2 = ID\nY3 = IG"
        n166 = local read "Plot transfer curve extrema vs time"() -> (w716:bool)
        n167 = Number To Decimal String(number=w758) -> (decimal integer string=w805:string)  [unwired: 1 in]
        n168 = Bundle By Name(cluster=w783, "Emergency Stop"=w808) -> (w816:T1)
        n169 = Delete From Array(array=w740, index=0 ("Index")) -> (deleted portion=w796:string, array with subset deleted=w795:string[])  [unwired: 1 in]
        n170 = local read "FPP - Source"() -> (w752:u32)
        n171 = local read "FPP - Drain"() -> (w750:u32)
        n172 = local read "FPP - Gate"() -> (w751:u32)
        n173 = Concatenate Strings(w804, "-transferfpp-" ("Substring"), w805, w756, ".txt" ("Substring")) -> (w807:string)
        n174 = VISA Write(VISA resource name=w775, write buffer=":PAGE:CHAN:MODE SWE;" ("write buffer (\"\")"), error in (no error)=w774) -> (VISA resource name out=w772:refnum<visa-resource-name>, error out=w773:errorcluster)  [unwired: 1 out]
        n175 = case shown="\"d\", Default" w796 {
          tunnel: [w900 w901] -> w794
          frame "s" {
            w900 = u16 0 items=["Single", "Double"] ("sweep mode")
          }
          frame "d", Default {
            w901 = u16 1 items=["Single", "Double"] ("sweep mode")
          }
        }
        n176 = Fract/Exp String To Number(string=w795) -> (number=w779:dbl[])  [unwired: 3 in, 1 out]
        n177 = local read "Plot transfer curve extrema vs time"() -> (w743:bool)
        n178 = String To Path(string=w807) -> (path=w803:path)
        n179 = Index Array(array=w779, index #1=0 ("Index")) -> (element #1=w793:dbl, element #2=w792:dbl, element #3=w791:dbl)  [unwired: 2 in]
        n180 = Delete From Array(array=w779, length=3 ("Length"), index=0 ("Index")) -> (array with subset deleted=w777:dbl[])  [unwired: 1 out]
        n181 = local read "FPP - Probe 1"() -> (w748:u32)
        n182 = local read "FPP - Probe 2"() -> (w749:u32)
        n183 = control-ref of="I vs Vg"() -> (w744:refnum<vi>)
        n184 = case shown="True" w743 {
          tunnel: w742 -> [w896 w899]
          tunnel: [w896 w898] -> w705
          tunnel: w741 -> [_ w897]
          frame False {
          }
          frame True {
            n185 = Build Array (concatenate)(w899, w897) -> (w898:i32[])
          }
        }
        n186 = Bundle By Name(cluster=w785, "Gate Start"=w793, "Gate Stop"=w792, "Gate Step (linear only)"=w791, "Gate Compliance"=w801, "Range mode"=w768, "Range"=w767) -> (w769:T6)
        n187 = Index Array(array=w777, index #1=0 ("Index")) -> (element #1=w788:dbl, element #2=w787:dbl, element #3=w786:dbl)  [unwired: 2 in]
        n188 = call <vilib>:"compatOverwrite.vi"("overwrite (F)"=TRUE) -> ("overwrite?"=w759:T8)
        n189 = Bundle By Name(cluster=w784, "Drain Start"=w788, "Drain Stop"=w787, "Drain Step"=w786, "Drain Compliance"=w802, "Range mode"=w766, "Range"=w765) -> (w770:T7)
        n190 = call "4155C Transfer-FPP v3.0.vi"("VISA resource name in"=w772, "FPP - Source"=w752, "Gate"=w769, "Drain"=w770, "FPP - Drain"=w750, "Timings"=w800, "error in (no error)"=w773, "FPP - Gate"=w751, "FPP - Probe 1"=w748, "sweep mode"=w794, "FPP - Probe 2"=w749, "Panel Controls"=w816) -> ("VG"=w746:dbl[], "Outparams"=w764:T9, "VISA Resource Name out"=w799:refnum<visa-resource-name>, "Vprobe2"=w761:dbl[], "ID"=w702:dbl[], "IG"=w704:dbl[], "Vprobe1"=w760:dbl[], "error out"=w707:errorcluster)  [unwired: 8 in]
        n191 = Unbundle By Name(w764) -> ("V2 Step"=w763:dbl, "V2 Start"=w762:dbl, "Number of points"=w703:i32)
        n192 = case shown="True" w716 {
          tunnel: w701 -> [w819 w895]
          tunnel: w731 -> [w820 w890]
          tunnel: w736 -> [w826 w886]
          tunnel: w737 -> [w827 w885]
          tunnel: w702 -> [_ w882]
          tunnel: w702 -> [_ w880]
          tunnel: w704 -> [_ w879]
          tunnel: w732 -> [w821 w875]
          tunnel: w733 -> [w823 w874]
          tunnel: w729 -> [w817 w871]
          tunnel: w730 -> [w818 w870]
          tunnel: w735 -> [w825 w867]
          tunnel: w734 -> [w824 w866]
          tunnel: w739 -> [w829 w863]
          tunnel: w738 -> [w828 w862]
          tunnel: w705 -> [_ w855]
          tunnel: [w817 w850] -> w723
          tunnel: w703 -> [_ w849]
          tunnel: [w818 w848] -> w724
          tunnel: [w819 w847] -> w725
          tunnel: [w820 w846] -> w726
          tunnel: [w821 w845] -> w727
          tunnel: [w823 w844] -> w728
          tunnel: [w829 w843] -> w720
          tunnel: [w828 w842] -> w719
          tunnel: [w827 w841] -> w718
          tunnel: [w826 w840] -> w717
          tunnel: [w825 w839] -> w721
          tunnel: [w824 w838] -> w722
          tunnel: w707 -> [w822 w837]
          tunnel: [w822 w833] -> w706
          frame False {
          }
          frame True {
            # "Y1 = Y2 = ID\nY3 = IG"
            # "Adjusts graph colors."
            # "Adjusts graph colors."
            # "Ion will be the middle element of the array. The calculation of the index is done only once, since Is, Id, and Ig have the same dimensions."
            # "abs(Ig)"
            # "abs(Is)"
            # "abs(Id)"
            # "Adjusts graph colors."
            # "Adjusts graph colors."
            # "Adjusts graph colors."
            n193 = Absolute Value(x=w880) -> (abs(x)=w865:dbl[])
            n194 = Absolute Value(x=w882) -> (abs(x)=w881:dbl[])
            n195 = Absolute Value(x=w879) -> (abs(x)=w868:dbl[])
            n196 = Array Size(array=w881) -> (size(s)=w889:i32)
            n197 = Divide(x=w889, y=2) -> (x/y=w832:dbl)
            n198 = Subtract(x=w832, y=1) -> (x-y=w831:dbl)
            n199 = Array Max & Min(array=w865) -> (max value=w872:dbl, min value=w873:dbl)  [unwired: 2 out]
            n200 = Array Max & Min(array=w881) -> (max value=w894:dbl, min value=w878:dbl)  [unwired: 2 out]
            n201 = Array Max & Min(array=w868) -> (max value=w877:dbl, min value=w876:dbl)  [unwired: 2 out]
            n202 = Index Array(array=w865, index=w831) -> (element=w856:dbl)
            n203 = Index Array(array=w865, index=0) -> (element=w857:dbl)
            n204 = Index Array(array=w881, index=w831) -> (element=w858:dbl)
            n205 = Index Array(array=w881, index=0) -> (element=w859:dbl)
            n206 = Index Array(array=w868, index=w831) -> (element=w861:dbl)
            n207 = Index Array(array=w868, index=0) -> (element=w860:dbl)
            n208 = local write "Ig max"(w877) -> ()
            n209 = local write "Ig min"(w876) -> ()
            n210 = local write "Is max"(w872) -> ()
            n211 = local write "Is min"(w873) -> ()
            n212 = local write "Id max"(w894) -> ()
            n213 = local write "Id min"(w878) -> ()
            n214 = Build Array (concatenate)(w871, w872) -> (w850:dbl[])
            n215 = Build Array (concatenate)(w870, w873) -> (w848:dbl[])
            n216 = local write "Is off"(w857) -> ()
            n217 = local write "Is on"(w856) -> ()
            n218 = Build Array (concatenate)(w895, w894) -> (w847:dbl[])
            n219 = Build Array (concatenate)(w890, w878) -> (w846:dbl[])
            n220 = Build Array (concatenate)(w875, w877) -> (w845:dbl[])
            n221 = Build Array (concatenate)(w874, w876) -> (w844:dbl[])
            n222 = Build Array (concatenate)(w863, w856) -> (w843:dbl[])
            n223 = Build Array (concatenate)(w862, w857) -> (w842:dbl[])
            n224 = Build Array (concatenate)(w885, w858) -> (w841:dbl[])
            n225 = Build Array (concatenate)(w886, w859) -> (w840:dbl[])
            n226 = Build Array (concatenate)(w867, w861) -> (w839:dbl[])
            n227 = Build Array (concatenate)(w866, w860) -> (w838:dbl[])
            n228 = local write "Ig off"(w860) -> ()
            n229 = local write "Ig on"(w861) -> ()
            n230 = local write "Id off"(w859) -> ()
            n231 = local write "Id on"(w858) -> ()
            n232 = control-ref of="Imax vs time"() -> (w884:refnum<vi>)
            n233 = control-ref of="Imin vs time"() -> (w883:refnum<vi>)
            n234 = control-ref of="Ion vs time"() -> (w852:refnum<vi>)
            n235 = control-ref of="Ioff vs time"() -> (w851:refnum<vi>)
            n236 = control-ref of="I vs Vg"() -> (w893:refnum<vi>)
            n237 = call "4155C Split array.vi"("Number of VAR2 steps"=w849, "Y2 data in"=w841, "X data in"=w855, "Y1 data in"=w843, "Y3 data in"=w839, "error in (no error)"=w837) -> ("Array of clusters"=w853:cluster{"Y data in":dbl[], "X data in":dbl[]}[], "error out"=w836:errorcluster)  [unwired: 1 in]
            n238 = call "4155C Split array.vi"("Number of VAR2 steps"=w849, "Y2 data in"=w840, "X data in"=w855, "Y1 data in"=w842, "Y3 data in"=w838, "error in (no error)"=w836) -> ("Array of clusters"=w854:cluster{"Y data in":dbl[], "X data in":dbl[]}[], "error out"=w835:errorcluster)  [unwired: 1 in]
            n239 = call "4155C Split array.vi"("Number of VAR2 steps"=w849, "Y2 data in"=w847, "X data in"=w855, "Y1 data in"=w850, "Y3 data in"=w845, "error in (no error)"=w835) -> ("Array of clusters"=w892:cluster{"Y data in":dbl[], "X data in":dbl[]}[], "error out"=w834:errorcluster)  [unwired: 1 in]
            n240 = call "4155C Split array.vi"("Number of VAR2 steps"=w849, "Y2 data in"=w846, "X data in"=w855, "Y1 data in"=w848, "Y3 data in"=w844, "error in (no error)"=w834) -> ("Array of clusters"=w891:cluster{"Y data in":dbl[], "X data in":dbl[]}[], "error out"=w833:errorcluster)  [unwired: 1 in]
            n241 = call "4155C Config Chart Colours.vi"("Numeric"=w849, "XY Graph 2"=w884) -> ()  [unwired: 6 in]
            n242 = call "4155C Config Chart Colours.vi"("Numeric"=w849, "XY Graph 2"=w883) -> ()  [unwired: 6 in]
            n243 = call "4155C Config Chart Colours.vi"("Numeric"=w849, "XY Graph 2"=w852) -> ()  [unwired: 6 in]
            n244 = call "4155C Config Chart Colours.vi"("Numeric"=w849, "XY Graph 2"=w851) -> ()  [unwired: 6 in]
            n245 = call "4155C Config Chart Colours.vi"("Numeric"=w849, "XY Graph 2"=w893) -> ()  [unwired: 6 in]
            n246 = local write "Imax vs time"(w892) -> ()
            n247 = local write "Imin vs time"(w891) -> ()
            n248 = local write "Ion vs time"(w853) -> ()
            n249 = local write "Ioff vs time"(w854) -> ()
          }
        }
        n250 = call "4155C Config Chart Colours.vi"("Numeric"=w703, "XY Graph 2"=w744) -> ()  [unwired: 6 in]
        n251 = call "4155C Split array.vi"("Number of VAR2 steps"=w703, "Y2 data in"=w702, "X data in"=w746, "Y1 data in"=w702, "Y3 data in"=w704, "error in (no error)"=w706) -> ("Array of clusters"=w747:cluster{"Y data in":dbl[], "X data in":dbl[]}[], "error out"=w745:errorcluster)  [unwired: 1 in]
        n252 = local write "I vs Vg"(w747) -> ()
        n253 = Open/Create/Replace File(file path (use dialog)=w803, error in=w745, operation (0:open)=w759) -> (refnum out=w813:refnum<file>, error out=w814:errorcluster)  [unwired: 3 in, 1 out]
        n254 = call "4155C Make Big 2d array FPP.vi"("1D Var1"=w746, "1d ID"=w702, "1d Vp2"=w761, "1d IG"=w704, "1d Vp1"=w760, "VAR2 START"=w762, "Number of VAR2 steps"=w703, "VAR2 STEP"=w763, "VAR1 Name"="Vg", "Decimal places in header"=i8 1, "VAR2 Name"="Vd") -> ("Header array"=w809:string[], "Data array"=w810:dbl[][])  [unwired: 15 in]
        n255 = call "4155C Write array to file.vi"("Byte Stream File Refnum"=w813, "Header"=w809, "Data Array"=w810, "error in (no error)"=w814) -> ("dup refnum"=w811:refnum<file>, "error out"=w812:errorcluster)  [unwired: 1 in]
        n256 = Close File(refnum=w811, error in=w812) -> (error out=w798:errorcluster)  [unwired: 1 out]
      }
      frame "output" {
        n257 = local read "Transfer/Output - Drain"() -> (w907:u32)
        n258 = local read "Transfer/Output - Source/Common"() -> (w906:u32)
        n259 = local read "Transfer/Output - Gate"() -> (w908:u32)
        n260 = Delete From Array(array=w1006, index=0 ("Index")) -> (deleted portion=w1004:string, array with subset deleted=w1003:string[])  [unwired: 1 in]
        n261 = Bundle By Name(cluster=w919, "Emergency Stop"=w1015) -> (w969:T1)
        n262 = Number To Decimal String(number=w965) -> (decimal integer string=w964:string)  [unwired: 1 in]
        n263 = case shown="\"d\", Default" w1004 {
          tunnel: [w1100 w1101] -> w1002
          frame "s" {
            w1100 = u16 0 items=["Single", "Double"] ("sweep mode")
          }
          frame "d", Default {
            w1101 = u16 1 items=["Single", "Double"] ("sweep mode")
          }
        }
        n264 = Fract/Exp String To Number(string=w1003) -> (number=w988:dbl[])  [unwired: 3 in, 1 out]
        n265 = Concatenate Strings(w1013, "-output-" ("Substring"), w964, w962, ".txt" ("Suffix (transfer)")) -> (w1014:string)
        n266 = VISA Write(VISA resource name=w984, write buffer=":PAGE:CHAN:MODE SWE;" ("write buffer (\"\")"), error in (no error)=w983) -> (VISA resource name out=w981:refnum<visa-resource-name>, error out=w982:errorcluster)  [unwired: 1 out]
        n267 = String To Path(string=w1014) -> (path=w1012:path)
        n268 = Index Array(array=w988, index #1=0 ("Index")) -> (element #1=w1001:dbl, element #2=w1000:dbl, element #3=w999:dbl)  [unwired: 2 in]
        n269 = Delete From Array(array=w988, length=3 ("Length"), index=0 ("Index")) -> (array with subset deleted=w986:dbl[])  [unwired: 1 out]
        n270 = local read "Plot output curve extrema vs time"() -> (w916:bool)
        n271 = local read "Transfer/Output - Probe 4"() -> (w909:u32)
        n272 = Bundle By Name(cluster=w993, "Gate Start"=w1001, "Gate Stop"=w1000, "Gate Step (linear only)"=w999, "Gate Compliance"=w1010, "Range mode"=w977, "Range"=w976) -> (w978:T6)
        n273 = case shown="True" w916 {
          tunnel: w961 -> [w1017 w1020]
          tunnel: w958 -> [_ w1019]
          tunnel: [w1017 w1018] -> w935
          frame False {
          }
          frame True {
            n274 = Build Array (concatenate)(w1020, w1019) -> (w1018:i32[])
          }
        }
        n275 = Index Array(array=w986, index #1=0 ("Index")) -> (element #1=w996:dbl, element #2=w995:dbl, element #3=w994:dbl)  [unwired: 2 in]
        n276 = call <vilib>:"compatOverwrite.vi"("overwrite (F)"=TRUE) -> ("overwrite?"=w968:T8)
        n277 = Bundle By Name(cluster=w992, "Drain Start"=w996, "Drain Stop"=w995, "Drain Step"=w994, "Drain Compliance"=w1011, "Range mode"=w975, "Range"=w974) -> (w979:T7)
        n278 = call "4155C Output v3.0.vi"("VISA resource name in"=w981, "Source/Common"=w906, 2:"Gate"=w978, 3:"Drain"=w979, 4:"Drain"=w907, "Timings"=w1009, "error in (no error)"=w982, 7:"Probe 4"=w915, 8:"Gate"=w908, 9:"Probe 4"=w909, "sweep mode"=w1002, "Panel controls"=w969, "Standby"=w910) -> ("VD"=w967:dbl[], "Outparams"=w973:T9, "VISA Resource Name out"=w1008:refnum<visa-resource-name>, "IS"=w945:dbl[], "ID"=w946:dbl[], "IG"=w944:dbl[], "error out"=w959:errorcluster, "Probe 4"=w970:dbl[])  [unwired: 7 in]
        n279 = Unbundle By Name(w973) -> ("V2 Step"=w972:dbl, "V2 Start"=w971:dbl, "Number of points"=w933:i32)
        n280 = call "4155C Split array.vi"("Number of VAR2 steps"=w933, "Y2 data in"=w946, "X data in"=w967, "Y1 data in"=w945, "Y3 data in"=w944, "error in (no error)"=w959) -> ("Array of clusters"=w960:cluster{"Y data in":dbl[], "X data in":dbl[]}[], "error out"=w921:errorcluster)  [unwired: 1 in]
        n281 = case shown="True" "Plot output curve extrema vs time" {
          tunnel: w966 -> [w1029 w1099]
          tunnel: w957 -> [w1030 w1094]
          tunnel: w948 -> [w1024 w1090]
          tunnel: w947 -> [w1023 w1089]
          tunnel: w946 -> [_ w1086]
          tunnel: w945 -> [_ w1084]
          tunnel: w944 -> [_ w1083]
          tunnel: w943 -> [w1031 w1079]
          tunnel: w942 -> [w1032 w1078]
          tunnel: w941 -> [w1027 w1075]
          tunnel: w940 -> [w1028 w1074]
          tunnel: w939 -> [w1025 w1071]
          tunnel: w938 -> [w1026 w1070]
          tunnel: w937 -> [w1021 w1067]
          tunnel: w936 -> [w1022 w1066]
          tunnel: w935 -> [_ w1059]
          tunnel: [w1027 w1054] -> w934
          tunnel: w933 -> [_ w1053]
          tunnel: [w1028 w1052] -> w932
          tunnel: [w1029 w1051] -> w931
          tunnel: [w1030 w1050] -> w930
          tunnel: [w1031 w1049] -> w929
          tunnel: [w1032 w1048] -> w928
          tunnel: [w1021 w1047] -> w927
          tunnel: [w1022 w1046] -> w926
          tunnel: [w1023 w1045] -> w925
          tunnel: [w1024 w1044] -> w924
          tunnel: [w1025 w1043] -> w923
          tunnel: [w1026 w1042] -> w922
          tunnel: w921 -> [w1033 w1041]
          tunnel: [w1033 w1037] -> w920
          frame False {
          }
          frame True {
            # "Adjusts graph colors."
            # "Adjusts graph colors."
            # "Ion will be the middle element of the array. The calculation of the index is done only once, since Is, Id, and Ig have the same dimensions."
            # "abs(Ig)"
            # "abs(Is)"
            # "Y1: Is\nY2: Id\nY3: Ig"
            # "abs(Id)"
            # "Adjusts graph colors."
            # "Adjusts graph colors."
            # "Adjusts graph colors."
            n282 = Absolute Value(x=w1084) -> (abs(x)=w1069:dbl[])
            n283 = Absolute Value(x=w1086) -> (abs(x)=w1085:dbl[])
            n284 = Absolute Value(x=w1083) -> (abs(x)=w1072:dbl[])
            n285 = Array Size(array=w1085) -> (size(s)=w1093:i32)
            n286 = Divide(x=w1093, y=2) -> (x/y=w1036:dbl)
            n287 = Subtract(x=w1036, y=1) -> (x-y=w1035:dbl)
            n288 = Array Max & Min(array=w1069) -> (max value=w1076:dbl, min value=w1077:dbl)  [unwired: 2 out]
            n289 = Array Max & Min(array=w1085) -> (max value=w1098:dbl, min value=w1082:dbl)  [unwired: 2 out]
            n290 = Array Max & Min(array=w1072) -> (max value=w1081:dbl, min value=w1080:dbl)  [unwired: 2 out]
            n291 = Index Array(array=w1069, index=w1035) -> (element=w1060:dbl)
            n292 = Index Array(array=w1069, index=0) -> (element=w1061:dbl)
            n293 = Index Array(array=w1085, index=w1035) -> (element=w1062:dbl)
            n294 = Index Array(array=w1085, index=0) -> (element=w1063:dbl)
            n295 = Index Array(array=w1072, index=w1035) -> (element=w1065:dbl)
            n296 = Index Array(array=w1072, index=0) -> (element=w1064:dbl)
            n297 = local write "Ig max"(w1081) -> ()
            n298 = local write "Ig min"(w1080) -> ()
            n299 = local write "Is max"(w1076) -> ()
            n300 = local write "Is min"(w1077) -> ()
            n301 = local write "Id max"(w1098) -> ()
            n302 = local write "Id min"(w1082) -> ()
            n303 = Build Array (concatenate)(w1075, w1076) -> (w1054:dbl[])
            n304 = Build Array (concatenate)(w1074, w1077) -> (w1052:dbl[])
            n305 = local write "Is off"(w1061) -> ()
            n306 = local write "Is on"(w1060) -> ()
            n307 = Build Array (concatenate)(w1099, w1098) -> (w1051:dbl[])
            n308 = Build Array (concatenate)(w1094, w1082) -> (w1050:dbl[])
            n309 = Build Array (concatenate)(w1079, w1081) -> (w1049:dbl[])
            n310 = Build Array (concatenate)(w1078, w1080) -> (w1048:dbl[])
            n311 = Build Array (concatenate)(w1067, w1060) -> (w1047:dbl[])
            n312 = Build Array (concatenate)(w1066, w1061) -> (w1046:dbl[])
            n313 = Build Array (concatenate)(w1089, w1062) -> (w1045:dbl[])
            n314 = Build Array (concatenate)(w1090, w1063) -> (w1044:dbl[])
            n315 = Build Array (concatenate)(w1071, w1065) -> (w1043:dbl[])
            n316 = Build Array (concatenate)(w1070, w1064) -> (w1042:dbl[])
            n317 = local write "Ig off"(w1064) -> ()
            n318 = local write "Ig on"(w1065) -> ()
            n319 = local write "Id off"(w1063) -> ()
            n320 = local write "Id on"(w1062) -> ()
            n321 = control-ref of="Imax vs time"() -> (w1088:refnum<vi>)
            n322 = control-ref of="Imin vs time"() -> (w1087:refnum<vi>)
            n323 = control-ref of="Ion vs time"() -> (w1056:refnum<vi>)
            n324 = control-ref of="Ioff vs time"() -> (w1055:refnum<vi>)
            n325 = control-ref of="I vs Vg"() -> (w1097:refnum<vi>)
            n326 = call "4155C Split array.vi"("Number of VAR2 steps"=w1053, "Y2 data in"=w1045, "X data in"=w1059, "Y1 data in"=w1047, "Y3 data in"=w1043, "error in (no error)"=w1041) -> ("Array of clusters"=w1057:cluster{"Y data in":dbl[], "X data in":dbl[]}[], "error out"=w1040:errorcluster)  [unwired: 1 in]
            n327 = call "4155C Split array.vi"("Number of VAR2 steps"=w1053, "Y2 data in"=w1044, "X data in"=w1059, "Y1 data in"=w1046, "Y3 data in"=w1042, "error in (no error)"=w1040) -> ("Array of clusters"=w1058:cluster{"Y data in":dbl[], "X data in":dbl[]}[], "error out"=w1039:errorcluster)  [unwired: 1 in]
            n328 = call "4155C Split array.vi"("Number of VAR2 steps"=w1053, "Y2 data in"=w1051, "X data in"=w1059, "Y1 data in"=w1054, "Y3 data in"=w1049, "error in (no error)"=w1039) -> ("Array of clusters"=w1096:cluster{"Y data in":dbl[], "X data in":dbl[]}[], "error out"=w1038:errorcluster)  [unwired: 1 in]
            n329 = call "4155C Split array.vi"("Number of VAR2 steps"=w1053, "Y2 data in"=w1050, "X data in"=w1059, "Y1 data in"=w1052, "Y3 data in"=w1048, "error in (no error)"=w1038) -> ("Array of clusters"=w1095:cluster{"Y data in":dbl[], "X data in":dbl[]}[], "error out"=w1037:errorcluster)  [unwired: 1 in]
            n330 = call "4155C Config Chart Colours.vi"("Numeric"=w1053, "XY Graph 2"=w1088) -> ()  [unwired: 6 in]
            n331 = call "4155C Config Chart Colours.vi"("Numeric"=w1053, "XY Graph 2"=w1087) -> ()  [unwired: 6 in]
            n332 = call "4155C Config Chart Colours.vi"("Numeric"=w1053, "XY Graph 2"=w1056) -> ()  [unwired: 6 in]
            n333 = call "4155C Config Chart Colours.vi"("Numeric"=w1053, "XY Graph 2"=w1055) -> ()  [unwired: 6 in]
            n334 = call "4155C Config Chart Colours.vi"("Numeric"=w1053, "XY Graph 2"=w1097) -> ()  [unwired: 6 in]
            n335 = local write "Imax vs time"(w1096) -> ()
            n336 = local write "Imin vs time"(w1095) -> ()
            n337 = local write "Ion vs time"(w1057) -> ()
            n338 = local write "Ioff vs time"(w1058) -> ()
          }
        }
        n339 = local write "I vs Vd"(w960) -> ()
        n340 = Open/Create/Replace File(file path (use dialog)=w1012, error in=w920, operation (0:open)=w968) -> (refnum out=w955:refnum<file>, error out=w953:errorcluster)  [unwired: 3 in, 1 out]
        n341 = call "4155C Make Big 2d array.vi"("1D Var1"=w967, "1d IS"=w945, "1d ID"=w946, "1d IG"=w944, "1d SMU4"=w970, "SMU4"=w915, "VAR2 START"=w971, "Number of VAR2 steps"=w933, "VAR2 STEP"=w972, "VAR1 Name"="Vd", "Decimal places in header"=i8 1, "VAR2 Name"="Vg") -> ("Header array"=w956:string[], "Data array"=w954:dbl[][])  [unwired: 14 in]
        n342 = call "4155C Write array to file.vi"("Byte Stream File Refnum"=w955, "Header"=w956, "Data Array"=w954, "error in (no error)"=w953) -> ("dup refnum"=w952:refnum<file>, "error out"=w951:errorcluster)  [unwired: 1 in]
        n343 = Close File(refnum=w952, error in=w951) -> (error out=w1007:errorcluster)  [unwired: 1 out]
      }
      frame "output-fpp" {
        # "Y1 = Y2 = ID\nY3 = IG"
        # "Adjusts graph colors."
        # "Adjusts graph colors."
        # "Y1 = Vp2\nY2 = Y3 = Vp1"
        n344 = local read "Plot output curve extrema vs time"() -> (w1141:bool)
        n345 = Number To Decimal String(number=w1163) -> (decimal integer string=w1207:string)  [unwired: 1 in]
        n346 = Bundle By Name(cluster=w1185, "Emergency Stop"=w1210) -> (w1220:T1)
        n347 = local read "Plot output curve extrema vs time"() -> (w1143:bool)
        n348 = local read "FPP - Source"() -> (w1156:u32)
        n349 = Delete From Array(array=w1142, index=0 ("Index")) -> (deleted portion=w1198:string, array with subset deleted=w1197:string[])  [unwired: 1 in]
        n350 = local read "FPP - Drain"() -> (w1157:u32)
        n351 = local read "FPP - Gate"() -> (w1158:u32)
        n352 = VISA Write(VISA resource name=w1176, write buffer=":PAGE:CHAN:MODE SWE;" ("write buffer (\"\")"), error in (no error)=w1173) -> (VISA resource name out=w1175:refnum<visa-resource-name>, error out=w1174:errorcluster)  [unwired: 1 out]
        n353 = Concatenate Strings(w1206, "-outputfpp-" ("Substring"), w1207, w1162, ".txt" ("Substring")) -> (w1209:string)
        n354 = case shown="\"d\", Default" w1198 {
          tunnel: [w1304 w1305] -> w1196
          frame "s" {
            w1304 = u16 0 items=["Single", "Double"] ("sweep mode")
          }
          frame "d", Default {
            w1305 = u16 1 items=["Single", "Double"] ("sweep mode")
          }
        }
        n355 = Fract/Exp String To Number(string=w1197) -> (number=w1179:dbl[])  [unwired: 3 in, 1 out]
        n356 = String To Path(string=w1209) -> (path=w1205:path)
        n357 = Index Array(array=w1179, index #1=0 ("Index")) -> (element #1=w1195:dbl, element #2=w1194:dbl, element #3=w1193:dbl)  [unwired: 2 in]
        n358 = Delete From Array(array=w1179, length=3 ("Length"), index=0 ("Index")) -> (array with subset deleted=w1178:dbl[])  [unwired: 1 out]
        n359 = local read "FPP - Probe 1"() -> (w1154:u32)
        n360 = local read "FPP - Probe 2"() -> (w1155:u32)
        n361 = case shown="True" w1143 {
          tunnel: w1144 -> [w1300 w1303]
          tunnel: w1145 -> [_ w1302]
          tunnel: [w1300 w1301] -> w1104
          frame False {
          }
          frame True {
            n362 = Build Array (concatenate)(w1303, w1302) -> (w1301:i32[])
          }
        }
        n363 = Bundle By Name(cluster=w1187, "Gate Start"=w1195, "Gate Stop"=w1194, "Gate Step (linear only)"=w1193, "Gate Compliance"=w1203, "Range mode"=w1171, "Range"=w1170) -> (w1219:T6)
        n364 = Index Array(array=w1178, index #1=0 ("Index")) -> (element #1=w1190:dbl, element #2=w1189:dbl, element #3=w1188:dbl)  [unwired: 2 in]
        n365 = call <vilib>:"compatOverwrite.vi"("overwrite (F)"=TRUE) -> ("overwrite?"=w1165:T8)
        n366 = Bundle By Name(cluster=w1186, "Drain Start"=w1190, "Drain Stop"=w1189, "Drain Step"=w1188, "Drain Compliance"=w1204, "Range mode"=w1169, "Range"=w1172) -> (w1218:T7)
        n367 = call "4155C Output-FPP v3.0.vi"("VISA resource name in"=w1175, "FPP - Source"=w1156, "Gate"=w1219, "Drain"=w1218, "FPP - Drain"=w1157, "Timings"=w1202, "error in (no error)"=w1174, "FPP - Gate"=w1158, "FPP - Probe 1"=w1154, "sweep mode"=w1196, "FPP - Probe 2"=w1155, "Panel controls"=w1220) -> ("VD"=w1150:dbl[], "Outparams"=w1167:T9, "VISA Resource Name out"=w1201:refnum<visa-resource-name>, "Vprobe2"=w1149:dbl[], "ID"=w1103:dbl[], "IG"=w1102:dbl[], "Vprobe1"=w1148:dbl[], "error out"=w1116:errorcluster)  [unwired: 8 in]
        n368 = Unbundle By Name(w1167) -> ("V2 Step"=w1168:dbl, "V2 Start"=w1166:dbl, "Number of points"=w1105:i32)
        n369 = case shown="True" w1141 {
          tunnel: w1137 -> [w1229 w1299]
          tunnel: w1138 -> [w1230 w1294]
          tunnel: w1132 -> [w1224 w1290]
          tunnel: w1131 -> [w1223 w1289]
          tunnel: w1103 -> [_ w1286]
          tunnel: w1103 -> [_ w1284]
          tunnel: w1102 -> [_ w1283]
          tunnel: w1139 -> [w1231 w1279]
          tunnel: w1140 -> [w1232 w1278]
          tunnel: w1135 -> [w1227 w1275]
          tunnel: w1136 -> [w1228 w1274]
          tunnel: w1133 -> [w1225 w1271]
          tunnel: w1134 -> [w1226 w1270]
          tunnel: w1129 -> [w1221 w1267]
          tunnel: w1130 -> [w1222 w1266]
          tunnel: w1104 -> [_ w1259]
          tunnel: [w1227 w1254] -> w1123
          tunnel: w1105 -> [_ w1253]
          tunnel: [w1228 w1252] -> w1124
          tunnel: [w1229 w1251] -> w1125
          tunnel: [w1230 w1250] -> w1126
          tunnel: [w1231 w1249] -> w1127
          tunnel: [w1232 w1248] -> w1128
          tunnel: [w1221 w1247] -> w1117
          tunnel: [w1222 w1246] -> w1118
          tunnel: [w1223 w1245] -> w1119
          tunnel: [w1224 w1244] -> w1120
          tunnel: [w1225 w1243] -> w1121
          tunnel: [w1226 w1242] -> w1122
          tunnel: w1116 -> [w1233 w1241]
          tunnel: [w1233 w1237] -> w1115
          frame False {
          }
          frame True {
            # "Y1 = Y2 = ID\nY3 = IG"
            # "Adjusts graph colors."
            # "Adjusts graph colors."
            # "Ion will be the middle element of the array. The calculation of the index is done only once, since Is, Id, and Ig have the same dimensions."
            # "abs(Ig)"
            # "abs(Is)"
            # "abs(Id)"
            # "Adjusts graph colors."
            # "Adjusts graph colors."
            # "Adjusts graph colors."
            n370 = Absolute Value(x=w1284) -> (abs(x)=w1269:dbl[])
            n371 = Absolute Value(x=w1286) -> (abs(x)=w1285:dbl[])
            n372 = Absolute Value(x=w1283) -> (abs(x)=w1272:dbl[])
            n373 = Array Size(array=w1285) -> (size(s)=w1293:i32)
            n374 = Divide(x=w1293, y=2) -> (x/y=w1236:dbl)
            n375 = Subtract(x=w1236, y=1) -> (x-y=w1235:dbl)
            n376 = Array Max & Min(array=w1269) -> (max value=w1276:dbl, min value=w1277:dbl)  [unwired: 2 out]
            n377 = Array Max & Min(array=w1285) -> (max value=w1298:dbl, min value=w1282:dbl)  [unwired: 2 out]
            n378 = Array Max & Min(array=w1272) -> (max value=w1281:dbl, min value=w1280:dbl)  [unwired: 2 out]
            n379 = Index Array(array=w1269, index=w1235) -> (element=w1260:dbl)
            n380 = Index Array(array=w1269, index=0) -> (element=w1261:dbl)
            n381 = Index Array(array=w1285, index=w1235) -> (element=w1262:dbl)
            n382 = Index Array(array=w1285, index=0) -> (element=w1263:dbl)
            n383 = Index Array(array=w1272, index=w1235) -> (element=w1265:dbl)
            n384 = Index Array(array=w1272, index=0) -> (element=w1264:dbl)
            n385 = local write "Ig max"(w1281) -> ()
            n386 = local write "Ig min"(w1280) -> ()
            n387 = local write "Is max"(w1276) -> ()
            n388 = local write "Is min"(w1277) -> ()
            n389 = local write "Id max"(w1298) -> ()
            n390 = local write "Id min"(w1282) -> ()
            n391 = Build Array (concatenate)(w1275, w1276) -> (w1254:dbl[])
            n392 = Build Array (concatenate)(w1274, w1277) -> (w1252:dbl[])
            n393 = local write "Is off"(w1261) -> ()
            n394 = local write "Is on"(w1260) -> ()
            n395 = Build Array (concatenate)(w1299, w1298) -> (w1251:dbl[])
            n396 = Build Array (concatenate)(w1294, w1282) -> (w1250:dbl[])
            n397 = Build Array (concatenate)(w1279, w1281) -> (w1249:dbl[])
            n398 = Build Array (concatenate)(w1278, w1280) -> (w1248:dbl[])
            n399 = Build Array (concatenate)(w1267, w1260) -> (w1247:dbl[])
            n400 = Build Array (concatenate)(w1266, w1261) -> (w1246:dbl[])
            n401 = Build Array (concatenate)(w1289, w1262) -> (w1245:dbl[])
            n402 = Build Array (concatenate)(w1290, w1263) -> (w1244:dbl[])
            n403 = Build Array (concatenate)(w1271, w1265) -> (w1243:dbl[])
            n404 = Build Array (concatenate)(w1270, w1264) -> (w1242:dbl[])
            n405 = local write "Ig off"(w1264) -> ()
            n406 = local write "Ig on"(w1265) -> ()
            n407 = local write "Id off"(w1263) -> ()
            n408 = local write "Id on"(w1262) -> ()
            n409 = control-ref of="Imax vs time"() -> (w1288:refnum<vi>)
            n410 = control-ref of="Imin vs time"() -> (w1287:refnum<vi>)
            n411 = control-ref of="Ion vs time"() -> (w1256:refnum<vi>)
            n412 = control-ref of="Ioff vs time"() -> (w1255:refnum<vi>)
            n413 = control-ref of="I vs Vg"() -> (w1297:refnum<vi>)
            n414 = call "4155C Split array.vi"("Number of VAR2 steps"=w1253, "Y2 data in"=w1245, "X data in"=w1259, "Y1 data in"=w1247, "Y3 data in"=w1243, "error in (no error)"=w1241) -> ("Array of clusters"=w1257:cluster{"Y data in":dbl[], "X data in":dbl[]}[], "error out"=w1240:errorcluster)  [unwired: 1 in]
            n415 = call "4155C Split array.vi"("Number of VAR2 steps"=w1253, "Y2 data in"=w1244, "X data in"=w1259, "Y1 data in"=w1246, "Y3 data in"=w1242, "error in (no error)"=w1240) -> ("Array of clusters"=w1258:cluster{"Y data in":dbl[], "X data in":dbl[]}[], "error out"=w1239:errorcluster)  [unwired: 1 in]
            n416 = call "4155C Split array.vi"("Number of VAR2 steps"=w1253, "Y2 data in"=w1251, "X data in"=w1259, "Y1 data in"=w1254, "Y3 data in"=w1249, "error in (no error)"=w1239) -> ("Array of clusters"=w1296:cluster{"Y data in":dbl[], "X data in":dbl[]}[], "error out"=w1238:errorcluster)  [unwired: 1 in]
            n417 = call "4155C Split array.vi"("Number of VAR2 steps"=w1253, "Y2 data in"=w1250, "X data in"=w1259, "Y1 data in"=w1252, "Y3 data in"=w1248, "error in (no error)"=w1238) -> ("Array of clusters"=w1295:cluster{"Y data in":dbl[], "X data in":dbl[]}[], "error out"=w1237:errorcluster)  [unwired: 1 in]
            n418 = call "4155C Config Chart Colours.vi"("Numeric"=w1253, "XY Graph 2"=w1288) -> ()  [unwired: 6 in]
            n419 = call "4155C Config Chart Colours.vi"("Numeric"=w1253, "XY Graph 2"=w1287) -> ()  [unwired: 6 in]
            n420 = call "4155C Config Chart Colours.vi"("Numeric"=w1253, "XY Graph 2"=w1256) -> ()  [unwired: 6 in]
            n421 = call "4155C Config Chart Colours.vi"("Numeric"=w1253, "XY Graph 2"=w1255) -> ()  [unwired: 6 in]
            n422 = call "4155C Config Chart Colours.vi"("Numeric"=w1253, "XY Graph 2"=w1297) -> ()  [unwired: 6 in]
            n423 = local write "Imax vs time"(w1296) -> ()
            n424 = local write "Imin vs time"(w1295) -> ()
            n425 = local write "Ion vs time"(w1257) -> ()
            n426 = local write "Ioff vs time"(w1258) -> ()
          }
        }
        n427 = call "4155C Split array.vi"("Number of VAR2 steps"=w1105, "Y2 data in"=w1148, "X data in"=w1150, "Y1 data in"=w1149, "Y3 data in"=w1148, "error in (no error)"=w1115) -> ("Array of clusters"=w1151:cluster{"Y data in":dbl[], "X data in":dbl[]}[], "error out"=w1114:errorcluster)  [unwired: 1 in]
        n428 = call "4155C Split array.vi"("Number of VAR2 steps"=w1105, "Y2 data in"=w1103, "X data in"=w1150, "Y1 data in"=w1103, "Y3 data in"=w1102, "error in (no error)"=w1114) -> ("Array of clusters"=w1153:cluster{"Y data in":dbl[], "X data in":dbl[]}[], "error out"=w1152:errorcluster)  [unwired: 1 in]
        n429 = local write "I vs Vd"(w1153) -> ()
        n430 = local write "Vp vs Vg (FPP)"(w1151) -> ()
        n431 = Open/Create/Replace File(file path (use dialog)=w1205, error in=w1152, operation (0:open)=w1165) -> (refnum out=w1215:refnum<file>, error out=w1216:errorcluster)  [unwired: 3 in, 1 out]
        n432 = call "4155C Make Big 2d array FPP.vi"("1D Var1"=w1150, "1d ID"=w1103, "1d Vp2"=w1149, "1d IG"=w1102, "1d Vp1"=w1148, "VAR2 START"=w1166, "Number of VAR2 steps"=w1105, "VAR2 STEP"=w1168, "VAR1 Name"="Vd", "Decimal places in header"=i8 1, "VAR2 Name"="Vg") -> ("Header array"=w1211:string[], "Data array"=w1212:dbl[][])  [unwired: 15 in]
        n433 = control-ref of="I vs Vd"() -> (w1147:refnum<vi>)
        n434 = control-ref of="Vp vs Vg (FPP)"() -> (w1146:refnum<vi>)
        n435 = call "4155C Write array to file.vi"("Byte Stream File Refnum"=w1215, "Header"=w1211, "Data Array"=w1212, "error in (no error)"=w1216) -> ("dup refnum"=w1213:refnum<file>, "error out"=w1214:errorcluster)  [unwired: 1 in]
        n436 = Close File(refnum=w1213, error in=w1214) -> (error out=w1200:errorcluster)  [unwired: 1 out]
        n437 = call "4155C Config Chart Colours.vi"("Numeric"=w1105, "XY Graph 2"=w1147) -> ()  [unwired: 6 in]
        n438 = call "4155C Config Chart Colours.vi"("Numeric"=w1105, "XY Graph 2"=w1146) -> ()  [unwired: 6 in]
      }
      frame "itime" {
        n439 = Delete From Array(array=w1317, index=1) -> (deleted portion=w1316:string)  [unwired: 1 in, 1 out]
        n440 = Delete From Array(array=w1317, index=0 ("Index")) -> (deleted portion=w1345:string)  [unwired: 1 in, 1 out]
        n441 = Fract/Exp String To Number(string=w1316) -> (number=w1315:dbl)  [unwired: 3 in, 1 out]
        n442 = case shown="\"l\"" w1345 {
          tunnel: w1344 -> [w1350 w1352 w1356]
          tunnel: [w1349 w1351 w1355] -> w1337
          tunnel: w1315 -> [w1347 _ w1354]
          frame "s" {
            w1348 = u32 0 items=["short  ", "medium  ", "long  "] ("integration time 2")
            n443 = Bundle By Name(cluster=w1350, "integration time"=w1348, "Short/Long integration time"=w1347) -> (w1349:T4)
          }
          frame "m", Default {
            w1353 = u32 1 items=["short  ", "medium  ", "long  "] ("integration time 2")
            n444 = Bundle By Name(cluster=w1352, "integration time"=w1353) -> (w1351:T4)
          }
          frame "l" {
            w1357 = u32 2 items=["short  ", "medium  ", "long  "] ("integration time 2")
            n445 = Bundle By Name(cluster=w1356, "integration time"=w1357, "Short/Long integration time"=w1354) -> (w1355:T4)
          }
        }
      }
      frame "pulsed" {
        n446 = Delete From Array(array=w1394, index=0 ("Index")) -> (deleted portion=w1395:string, array with subset deleted=w1382:string[])  [unwired: 1 in]
        n447 = case shown="\"on\", Default" w1395 {
          tunnel: w1393 -> [w1405 w1408]
          tunnel: [w1404 w1407] -> w1386
          tunnel: w1382 -> [w1402 _]
          frame "on", Default {
            w1403 = u16 1 items=["Continuous", "Pulsed"] ("sweep method")
            n448 = Fract/Exp String To Number(string=w1402) -> (number=w1400:dbl[])  [unwired: 3 in, 1 out]
            n449 = Index Array(array=w1400, index #1=0 ("Index")) -> (element #1=w1399:dbl, element #2=w1398:dbl, element #3=w1397:dbl)  [unwired: 2 in]
            n450 = Bundle By Name(cluster=w1405, "sweep method"=w1403, "Pulse period"=w1399, "Base voltage"=w1398, "Pulse width"=w1397) -> (w1404:T4)
          }
          frame "off" {
            w1406 = u16 0 items=["Continuous", "Pulsed"] ("sweep method")
            n451 = Bundle By Name(cluster=w1408, "sweep method"=w1406) -> (w1407:T4)
          }
        }
      }
      frame "gaterangemode" {
        n452 = Delete From Array(array=w1443, index=0 ("Index")) -> (deleted portion=w1444:string)  [unwired: 1 in, 1 out]
        n453 = case shown="\"f\"" w1444 {
          tunnel: [w1446 w1447 w1448] -> w1433
          frame "a", Default {
            w1446 = u16 0 items=["Auto", "Limited", "Fixed"] ("Gate Range\nmode 2")
          }
          frame "f" {
            w1447 = u16 2 items=["Auto", "Limited", "Fixed"] ("Gate Range\nmode 2")
          }
          frame "l" {
            w1448 = u16 1 items=["Auto", "Limited", "Fixed"] ("Gate Range\nmode 2")
          }
        }
      }
      frame "gaterange" {
        (unwired) u8 11 items=["10fA  ", "100fA  ", "1nA  ", "10nA", "100nA", "1uA", "10uA", "100uA", "1mA", "10mA", "100mA", "1A"] ("Gate Range 2")
        n454 = Delete From Array(array=w1490, index=0 ("Index")) -> (deleted portion=w1480:string)  [unwired: 1 in, 1 out]
        n455 = Scan Value(string=w1480, format string="") -> (value=w1478:dbl)  [unwired: 1 in, 1 out]
        n456 = Logarithm Base 10(1:w1478) -> (0:w1477:dbl)
        n457 = Round To Nearest(number=w1477) -> (nearest integer value=w1476:dbl)
        n458 = Add(x=w1476, y=11.0) -> (x+y=w1474:dbl)
        n459 = To Unsigned Byte Integer(number=w1474) -> (unsigned 8bit integer=w1473:u8)
      }
      frame "drainrange" {
        (unwired) u8 11 items=["10fA  ", "100fA  ", "1nA  ", "10nA", "100nA", "1uA", "10uA", "100uA", "1mA", "10mA", "100mA", "1A"] ("Gate Range 2")
        n460 = Delete From Array(array=w1533, index=0 ("Index")) -> (deleted portion=w1524:string)  [unwired: 1 in, 1 out]
        n461 = Scan Value(string=w1524, format string="") -> (value=w1522:dbl)  [unwired: 1 in, 1 out]
        n462 = Logarithm Base 10(1:w1522) -> (0:w1521:dbl)
        n463 = Round To Nearest(number=w1521) -> (nearest integer value=w1520:dbl)
        n464 = Add(x=w1520, y=11.0) -> (x+y=w1518:dbl)
        n465 = To Unsigned Byte Integer(number=w1518) -> (unsigned 8bit integer=w1517:u8)
      }
      frame "drainrangemode" {
        n466 = Delete From Array(array=w1569, index=0 ("Index")) -> (deleted portion=w1570:string)  [unwired: 1 in, 1 out]
        n467 = case shown="\"f\"" w1570 {
          tunnel: [w1572 w1573 w1574] -> w1559
          frame "a", Default {
            w1572 = u16 0 items=["Auto", "Limited", "Fixed"] ("Gate Range\nmode 2")
          }
          frame "f" {
            w1573 = u16 2 items=["Auto", "Limited", "Fixed"] ("Gate Range\nmode 2")
          }
          frame "l" {
            w1574 = u16 1 items=["Auto", "Limited", "Fixed"] ("Gate Range\nmode 2")
          }
        }
      }
      frame "Error", Default {
      }
      frame "logfile" {
        n468 = Number To Decimal String(number=w1633) -> (decimal integer string=w1668:string)  [unwired: 1 in]
        n469 = Concatenate Strings(w1667, "logfile" ("Substring"), w1668, w1631, ".txt" ("Substring")) -> (w1665:string)
        n470 = String To Path(string=w1665) -> (path=w1638:path)
        n471 = Unbundle(w1664) -> ("integration time"=w1663:u32, "Short/Long integration time"=w1662:dbl, "hold time (sec)"=w1661:dbl, "delay time (sec)"=w1660:dbl, "Step Time (0 disables)"=w1659:dbl, "sweep method"=w1658:u16, "Pulse period"=w1657:dbl, "Base voltage"=w1656:dbl, "Pulse width"=w1655:dbl)
        n472 = Build Array(w1663, w1662, w1661, w1660, w1659, w1658, w1657, w1656, w1655, w1649, w1650, w1651, w1652, w1653, w1654) -> (w1642:dbl[])
        n473 = Insert Into Array(array=dbl[][] [] ("Input Array"), new element=w1642) -> (w1641:dbl[][])  [unwired: 2 in]
        n474 = call <vilib>:"compatOverwrite.vi"("overwrite (F)"=TRUE) -> ("overwrite?"=w1636:T8)
        n475 = Open/Create/Replace File(file path (use dialog)=w1638, error in=w1640, operation (0:open)=w1636) -> (refnum out=w1646:refnum<file>, error out=w1645:errorcluster)  [unwired: 3 in, 1 out]
        n476 = call "4155C Write array to file.vi"("Byte Stream File Refnum"=w1646, "Header"=string[] ["Int Time", "Short/Long Itime", "Hold time", "Delay time", "Step time", "Sweep method", "Pulse period", "Base Voltage", "Pulse width", "Drain compliance", "Gate compliance", "Gate range mode", "Gate range", "S/D range mode", "S/D range"], "Data Array"=w1641, "error in (no error)"=w1645) -> ("dup refnum"=w1648:refnum<file>, "error out"=w1647:errorcluster)  [unwired: 1 in]
        n477 = Close File(refnum=w1648, error in=w1647) -> (error out=w1639:errorcluster)  [unwired: 1 out]
      }
      frame "sample" {
        w1696 = 1
        # "Add a time offset (elapsed time) to the time axis."
        # "Adjusts graph colors."
        n478 = Number To Decimal String(number=w1728) -> (decimal integer string=w1770:string)  [unwired: 1 in]
        n479 = Fract/Exp String To Number(string=w1767) -> (number=w1732:dbl[])  [unwired: 3 in, 1 out]
        n480 = local read "Sample - Probe 4"() -> (w1678:u32)
        n481 = Concatenate Strings(w1748, "-sample-" ("Substring"), w1770, w1726, ".txt" ("Substring")) -> (w1768:string)
        n482 = local read "Sample - Drain"() -> (w1679:u32)
        n483 = Index Array(array=w1732, index=0 ("Index")) -> (element=w1765:dbl)
        n484 = String To Path(string=w1768) -> (path=w1752:path)
        n485 = Index Array(array=w1732, index=2 ("Index")) -> (element=w1761:dbl)
        n486 = Index Array(array=w1732, index=3 ("Index")) -> (element=w1734:dbl)
        n487 = Index Array(array=w1732, index=4 ("Index")) -> (element=w1731:dbl)
        n488 = Index Array(array=w1732, index=1 ("Index")) -> (element=w1762:dbl)
        n489 = local read "Plot sample extrema vs time"() -> (w1699:bool)
        n490 = local read "Time Units"() -> (w1674:u16)
        n491 = local read "Sample - Gate"() -> (w1681:u32)
        n492 = local read "Sample - Source/Common"() -> (w1680:u32)
        n493 = call "4155C Config Sampling Measurements v3.0.vi"("VISA session"=w1773, "Num Points"=w1761, "Sample - Drain"=w1679, "Display on/off"=TRUE, "Gate Compliance"=w1749, "Sampling interval"=w1731, "Sample - Source/Common"=w1680, "Sample - Probe 4"=w1678, "Drain Compliance"=w1771, "Standby"=w1682, "error in (no error)"=w1772, "Timings"=w1740, "Sample - Gate"=w1681, "Sample time"=w1734) -> ("dup VISA resource name"=w1775:refnum<visa-resource-name>, "error out"=w1774:errorcluster)
        n494 = call "4155C Take Sample v3.0.vi"("VISA resource name in"=w1775, "Emergency Stop"=w1745, "Sample - Gate"=w1681, "Vg"=w1765, "Sample - Drain"=w1679, "Vd"=w1762, "error in (no error)"=w1774) -> ("Time"=w1676:dbl[], "VISA Resource Name out"=w1742:refnum<visa-resource-name>, "Ig"=w1692:dbl[], "Id"=w1693:dbl[], "Is"=w1694:dbl[], "error out"=w1697:errorcluster)  [unwired: 3 in]
        n495 = case shown="0, Default" w1674 {
          tunnel: [w1778 w1779 w1782] -> w1677
          tunnel: w1676 -> [w1777 w1779 w1781]
          frame 2 {
            n496 = Divide(x=w1777, y=3600.0) -> (x/y=w1778:dbl[])
          }
          frame 0, Default {
          }
          frame 1 {
            n497 = Divide(x=w1781, y=60.0) -> (x/y=w1782:dbl[])
          }
        }
        n498 = Insert Into Array(array=w1690, new element=w1693) -> (w1684:dbl[])  [unwired: 1 in]
        n499 = Add(x=w1677, y=w1675) -> (x+y=w1695:dbl[])
        n500 = Insert Into Array(array=w1689, new element=w1694) -> (w1685:dbl[])  [unwired: 1 in]
        n501 = Insert Into Array(array=w1691, new element=w1692) -> (w1687:dbl[])  [unwired: 1 in]
        n502 = case shown="True" w1699 {
          tunnel: w1700 -> [w1783 w1785]
          tunnel: [w1783 w1786] -> w1698
          tunnel: w1695 -> [_ w1784]
          frame False {
          }
          frame True {
            n503 = Insert Into Array(array=w1785, new element=w1784) -> (w1786:i32[])  [unwired: 1 in]
          }
        }
        n504 = case shown="True" "Plot sample extrema vs time" {
          tunnel: w1694 -> [_ w1814]
          tunnel: w1693 -> [_ w1815]
          tunnel: w1692 -> [_ w1816]
          tunnel: [w1793 w1803] -> w1683
          tunnel: w1697 -> [w1793 w1807]
          tunnel: w1721 -> [w1792 w1819]
          tunnel: w1720 -> [w1791 w1818]
          tunnel: w1719 -> [w1790 w1820]
          tunnel: w1718 -> [w1789 w1817]
          tunnel: w1717 -> [w1788 w1822]
          tunnel: w1716 -> [w1787 w1821]
          tunnel: [w1792 w1805] -> w1715
          tunnel: [w1791 w1798] -> w1714
          tunnel: [w1790 w1799] -> w1713
          tunnel: [w1789 w1823] -> w1712
          tunnel: [w1788 w1806] -> w1711
          tunnel: [w1787 w1800] -> w1710
          tunnel: w1698 -> [_ w1794]
          frame False {
          }
          frame True {
            w1801 = 1
            # "Number of VAR2 steps is 1."
            # "abs(Ig)"
            # "abs(Is)"
            # "abs(Id)"
            # "Adjusts graph colors."
            n505 = Absolute Value(x=w1816) -> (abs(x)=w1795:dbl[])
            n506 = Absolute Value(x=w1815) -> (abs(x)=w1796:dbl[])
            n507 = Absolute Value(x=w1814) -> (abs(x)=w1797:dbl[])
            n508 = Array Max & Min(array=w1797) -> (max value=w1813:dbl, min value=w1810:dbl)  [unwired: 2 out]
            n509 = Array Max & Min(array=w1796) -> (max value=w1812:dbl, min value=w1809:dbl)  [unwired: 2 out]
            n510 = Array Max & Min(array=w1795) -> (max value=w1811:dbl, min value=w1808:dbl)  [unwired: 2 out]
            n511 = local write "Id max"(w1812) -> ()
            n512 = local write "Id min"(w1809) -> ()
            n513 = local write "Ig max"(w1811) -> ()
            n514 = local write "Ig min"(w1808) -> ()
            n515 = Insert Into Array(array=w1822, new element=w1795) -> (w1806:dbl[])  [unwired: 1 in]
            n516 = Insert Into Array(array=w1821, new element=w1795) -> (w1800:dbl[])  [unwired: 1 in]
            n517 = local write "Is max"(w1813) -> ()
            n518 = local write "Is min"(w1810) -> ()
            n519 = Insert Into Array(array=w1820, new element=w1796) -> (w1799:dbl[])  [unwired: 1 in]
            n520 = Insert Into Array(array=w1817, new element=w1796) -> (w1823:dbl[])  [unwired: 1 in]
            n521 = Insert Into Array(array=w1819, new element=w1797) -> (w1805:dbl[])  [unwired: 1 in]
            n522 = Insert Into Array(array=w1818, new element=w1797) -> (w1798:dbl[])  [unwired: 1 in]
            n523 = control-ref of="Imax vs time"() -> (w1824:refnum<vi>)
            n524 = call "4155C Config Chart Colours.vi"("Numeric"=w1801, "XY Graph 2"=w1824) -> ()  [unwired: 6 in]
            n525 = call "4155C Split array.vi"("Number of VAR2 steps"=w1801, "Y2 data in"=w1799, "X data in"=w1794, "Y1 data in"=w1805, "Y3 data in"=w1806, "error in (no error)"=w1807) -> ("Array of clusters"=w1825:cluster{"Y data in":dbl[], "X data in":dbl[]}[], "error out"=w1804:errorcluster)  [unwired: 1 in]
            n526 = call "4155C Split array.vi"("Number of VAR2 steps"=w1801, "Y2 data in"=w1799, "X data in"=w1794, "Y1 data in"=w1798, "Y3 data in"=w1800, "error in (no error)"=w1804) -> ("Array of clusters"=w1802:cluster{"Y data in":dbl[], "X data in":dbl[]}[], "error out"=w1803:errorcluster)  [unwired: 1 in]
            n527 = local write "Imax vs time"(w1825) -> ()
            n528 = local write "Imin vs time"(w1802) -> ()
          }
        }
        n529 = Insert Into Array(array=w1688, new element=w1695) -> (w1686:dbl[])  [unwired: 1 in]
        n530 = control-ref of="I vs time (Bias Stress)"() -> (w1703:refnum<vi>)
        n531 = call "4155C Split array.vi"("Number of VAR2 steps"=w1696, "Y2 data in"=w1684, "X data in"=w1686, "Y1 data in"=w1685, "Y3 data in"=w1687) -> ("Array of clusters"=w1702:cluster{"Y data in":dbl[], "X data in":dbl[]}[])  [unwired: 2 in, 1 out]
        n532 = call "4155C Config Chart Colours.vi"("Numeric"=w1696, "XY Graph 2"=w1703) -> ()  [unwired: 6 in]
        n533 = local write "I vs time (Bias Stress)"(w1702) -> ()
        n534 = Insert Into Array(array=dbl[][] [] ("Input Array"), new element=w1695) -> (w1701:dbl[][])  [unwired: 2 in]
        n535 = Insert Into Array(array=w1701, new element=w1692) -> (w1755:dbl[][])  [unwired: 2 in]
        n536 = VISA Write(VISA resource name=w1742, write buffer=":DISP ON" ("write buffer (\"\")"), error in (no error)=w1683) -> (VISA resource name out=w1741:refnum<visa-resource-name>, error out=w1743:errorcluster)  [unwired: 1 out]
        n537 = Insert Into Array(array=w1755, new element=w1693) -> (w1754:dbl[][])  [unwired: 2 in]
        n538 = Insert Into Array(array=w1754, new element=w1694) -> (w1747:dbl[][])  [unwired: 2 in]
        n539 = Transpose 2D Array(2D array=w1747) -> (transposed array=w1746:dbl[][])
        n540 = call <vilib>:"compatOverwrite.vi"("overwrite (F)"=TRUE) -> ("overwrite?"=w1729:T8)
        n541 = Open/Create/Replace File(file path (use dialog)=w1752, error in=w1743, operation (0:open)=w1729) -> (refnum out=w1758:refnum<file>, error out=w1757:errorcluster)  [unwired: 3 in, 1 out]
        n542 = call "4155C Write array to file.vi"("Byte Stream File Refnum"=w1758, "Header"=string[] ["Time /Units", "Ig /A", "Id /A", "Is /A"], "Data Array"=w1746, "error in (no error)"=w1757) -> ("dup refnum"=w1760:refnum<file>, "error out"=w1759:errorcluster)  [unwired: 1 in]
        n543 = Close File(refnum=w1760, error in=w1759) -> (error out=w1750:errorcluster)  [unwired: 1 out]
      }
      frame "samplei" {
        w1838 = 1
        # "Adjusts graph colors."
        # "Add a time offset (elapsed time) to the time axis."
        n544 = local read "Sample I - Source/Common"() -> (w1850:u32)
        n545 = Number To Decimal String(number=w1873) -> (decimal integer string=w1921:string)  [unwired: 1 in]
        n546 = local read "Sample I - Probe 4 (Disabled)"() -> (w1853:u32)
        n547 = Concatenate Strings(w1902, "-samplei-" ("Substring"), w1921, w1872, ".txt" ("Substring")) -> (w1919:string)
        n548 = Fract/Exp String To Number(string=w1918) -> (number=w1887:dbl[])  [unwired: 3 in, 1 out]
        n549 = String To Path(string=w1919) -> (path=w1905:path)
        n550 = local read "Sample I - Probe 3 (Disabled)"() -> (w1852:u32)
        n551 = Index Array(array=w1887, index=4 ("Index")) -> (element=w1881:dbl)
        n552 = Index Array(array=w1887, index=3 ("Index")) -> (element=w1882:dbl)
        n553 = Index Array(array=w1887, index=1 ("Index")) -> (element=w1884:dbl)
        n554 = Index Array(array=w1887, index=0 ("Index")) -> (element=w1885:dbl)
        n555 = Index Array(array=w1887, index=2 ("Index")) -> (element=w1883:dbl)
        n556 = local read "Sample I - Drain/Gate"() -> (w1851:u32)
        n557 = call "4155C Config SamplingI Measurements v3.0.vi"("VISA session"=w1924, "Num Points"=w1884, "Sample I - Probe 3 (Disabled)"=w1852, "Display on/off"=TRUE, "Sample I - Source/Common"=w1850, "Sample I - Drain/Gate"=w1851, "Sampling interval"=w1882, "Standby"=w1854, "error in (no error)"=w1923, "Timings"=w1894, "Sample I - Probe 4 (Disabled)"=w1853, "Sample time"=w1883) -> ("dup VISA resource name"=w1926:refnum<visa-resource-name>, "error out"=w1925:errorcluster)  [unwired: 2 in]
        n558 = local read "Plot sample extrema vs time"() -> (w1847:bool)
        n559 = local read "Time Units"() -> (w1843:u16)
        n560 = call "4155C Take SampleI v3.0.vi"("Sample I - Drain/Gate"=w1851, "Emergency Stop"=w1899, "error in (no error)"=w1925, "Idg 2"=w1885, "Vdg compliance 2"=w1881, "VISA resource name in"=w1926) -> ("error out"=w1897:errorcluster, "Idg"=w1830:dbl[], "Vdg"=w1831:dbl[], "VISA Resource Name out"=w1895:refnum<visa-resource-name>, "Is"=w1827:dbl[], "Time"=w1842:dbl[])
        n561 = case shown="0, Default" w1843 {
          tunnel: [w1929 w1930 w1933] -> w1844
          tunnel: w1842 -> [w1928 w1930 w1932]
          frame 2 {
            n562 = Divide(x=w1928, y=3600.0) -> (x/y=w1929:dbl[])
          }
          frame 0, Default {
          }
          frame 1 {
            n563 = Divide(x=w1932, y=60.0) -> (x/y=w1933:dbl[])
          }
        }
        n564 = Add(x=w1844, y=w1841) -> (x+y=w1836:dbl[])
        n565 = Insert Into Array(array=w1837, new element=w1836) -> (w1835:dbl[])  [unwired: 1 in]
        n566 = case shown="True" w1847 {
          tunnel: w1846 -> [w1934 w1936]
          tunnel: [w1934 w1937] -> w1845
          tunnel: w1836 -> [_ w1935]
          frame False {
          }
          frame True {
            n567 = Insert Into Array(array=w1936, new element=w1935) -> (w1937:i32[])  [unwired: 1 in]
          }
        }
        n568 = control-ref of="Vdg vs time (Bias Stress)"() -> (w1840:refnum<vi>)
        n569 = Insert Into Array(array=dbl[][] [] ("Input Array"), new element=w1836) -> (w1909:dbl[][])  [unwired: 2 in]
        n570 = call "4155C Config Chart Colours.vi"("Numeric"=w1838, "XY Graph 2"=w1840) -> ()  [unwired: 6 in]
        n571 = Insert Into Array(array=w1834, new element=w1831) -> (w1826:dbl[])  [unwired: 1 in]
        n572 = call "4155C Split array.vi"("Number of VAR2 steps"=w1838, "X data in"=w1835, "Y1 data in"=w1826) -> ("Array of clusters"=w1839:cluster{"Y data in":dbl[], "X data in":dbl[]}[])  [unwired: 4 in, 1 out]
        n573 = local write "Vdg vs time (Bias Stress)"(w1839) -> ()
        n574 = Insert Into Array(array=w1833, new element=w1830) -> (w1832:dbl[])  [unwired: 1 in]
        n575 = Insert Into Array(array=w1909, new element=w1831) -> (w1908:dbl[][])  [unwired: 2 in]
        n576 = Insert Into Array(array=w1829, new element=w1827) -> (w1828:dbl[])  [unwired: 1 in]
        n577 = Insert Into Array(array=w1908, new element=w1830) -> (w1907:dbl[][])  [unwired: 2 in]
        n578 = VISA Write(VISA resource name=w1895, write buffer=":DISP ON" ("write buffer (\"\")"), error in (no error)=w1897) -> (VISA resource name out=w1880:refnum<visa-resource-name>, error out=w1896:errorcluster)  [unwired: 1 out]
        n579 = Insert Into Array(array=w1907, new element=w1827) -> (w1901:dbl[][])  [unwired: 2 in]
        n580 = call <vilib>:"compatOverwrite.vi"("overwrite (F)"=TRUE) -> ("overwrite?"=w1875:T8)
        n581 = Open/Create/Replace File(file path (use dialog)=w1905, error in=w1896, operation (0:open)=w1875) -> (refnum out=w1912:refnum<file>, error out=w1911:errorcluster)  [unwired: 3 in, 1 out]
        n582 = Transpose 2D Array(2D array=w1901) -> (transposed array=w1900:dbl[][])
        n583 = call "4155C Write array to file.vi"("Byte Stream File Refnum"=w1912, "Header"=string[] ["Time /s", "Vdg /V", "Idg /A", "Is /A"], "Data Array"=w1900, "error in (no error)"=w1911) -> ("dup refnum"=w1914:refnum<file>, "error out"=w1913:errorcluster)  [unwired: 1 in]
        n584 = Close File(refnum=w1914, error in=w1913) -> (error out=w1878:errorcluster)  [unwired: 1 out]
        n585 = VISA Write(VISA resource name=w1880, write buffer=";:PAGE:SCON:STAN OFF;:PAGE:CHAN:VSU2:DIS;" ("write buffer (\"\")"), error in (no error)=w1878) -> (VISA resource name out=w1876:refnum<visa-resource-name>, error out=w1877:errorcluster)  [unwired: 1 out]
      }
      frame "#" {
        n586 = VISA Write(VISA resource name=w1966, write buffer=":DISP ON" ("write buffer (\"\")"), error in (no error)=w1965) -> (VISA resource name out=w1964:refnum<visa-resource-name>, error out=w1963:errorcluster)  [unwired: 1 out]
      }
      frame "stressV" {
        n587 = Number To Decimal String(number=w2001) -> (decimal integer string=w2042:string)  [unwired: 1 in]
        n588 = Concatenate Strings(w2026, "-stressV-" ("Substring"), w2042, w2000, ".txt" ("Substring")) -> (w2040:string)
        n589 = Fract/Exp String To Number(string=w2039) -> (number=w2012:dbl[])  [unwired: 3 in, 1 out]
        n590 = local read "Stress V - Drain"() -> (w1979:u32)
        n591 = String To Path(string=w2040) -> (path=w2030:path)
        n592 = Index Array(array=w2012, index=3 ("Index")) -> (element=w2009:dbl)
        n593 = Index Array(array=w2012, index=1 ("Index")) -> (element=w2007:dbl)
        n594 = Index Array(array=w2012, index=0 ("Index")) -> (element=w2006:dbl)
        n595 = Index Array(array=w2012, index=4 ("Index")) -> (element=w2011:dbl)
        n596 = Index Array(array=w2012, index=2 ("Index")) -> (element=w2008:dbl)
        n597 = local read "Stress V - Gate"() -> (w1980:u32)
        n598 = local read "Stress V - Source/Common"() -> (w1981:u32)
        n599 = call "4155C Config V Stress v3.0.vi"("Display on/off"=TRUE, "Stress V - Gate"=w1980, "Stress V - Drain"=w1979, "Stress V - Source/Common"=w1981, "IG compliance"=w2008, "ID compliance"=w2009, "error in (no error)"=w2044, "VG"=w2006, "VD"=w2007, "VISA session"=w2045) -> ("error out"=w2046:errorcluster, "dup VISA resource name"=w2047:refnum<visa-resource-name>)
        n600 = call "4155C Apply Stress.vi"("error in (no error)"=w2046, "Duration"=w2011, "Emergency Stop"=w2025, "VISA resource name in"=w2047) -> ("error out"=w2023:errorcluster, "VISA Resource Name out"=w2021:refnum<visa-resource-name>)
        n601 = VISA Write(VISA resource name=w2021, write buffer=":DISP ON" ("write buffer (\"\")"), error in (no error)=w2023) -> (VISA resource name out=w2020:refnum<visa-resource-name>, error out=w2022:errorcluster)  [unwired: 1 out]
        n602 = call <vilib>:"compatOverwrite.vi"("overwrite (F)"=TRUE) -> ("overwrite?"=w2005:T8)
        n603 = Open/Create/Replace File(file path (use dialog)=w2030, error in=w2022, operation (0:open)=w2005) -> (refnum out=w2033:refnum<file>, error out=w2032:errorcluster)  [unwired: 3 in, 1 out]
        n604 = call "4155C Write array to file.vi"("Byte Stream File Refnum"=w2033, "Header"=string[] ["V stress completed successfully", ""], "error in (no error)"=w2032) -> ("dup refnum"=w2035:refnum<file>, "error out"=w2034:errorcluster)  [unwired: 2 in]
        n605 = Close File(refnum=w2035, error in=w2034) -> (error out=w2028:errorcluster)  [unwired: 1 out]
      }
      frame "stressI" {
        n606 = Number To Decimal String(number=w2073) -> (decimal integer string=w2110:string)  [unwired: 1 in]
        n607 = Concatenate Strings(w2094, "-stressI-" ("Substring"), w2110, w2072, ".txt" ("Substring")) -> (w2108:string)
        n608 = Fract/Exp String To Number(string=w2107) -> (number=w2082:dbl[])  [unwired: 3 in, 1 out]
        n609 = local read "Stress I - Source/Common"() -> (w2052:u32)
        n610 = Index Array(array=w2082, index=1 ("Index")) -> (element=w2078:dbl)
        n611 = Index Array(array=w2082, index=0 ("Index")) -> (element=w2079:dbl)
        n612 = Index Array(array=w2082, index=2 ("Index")) -> (element=w2080:dbl)
        n613 = String To Path(string=w2108) -> (path=w2098:path)
        n614 = local read "Stress I - Drain/Gate"() -> (w2053:u32)
        n615 = call "4155C Config I Stress v3.0.vi"("Stress I - Drain/Gate"=w2053, "Stress I - Source/Common"=w2052, "Display on/off"=TRUE, "error in (no error)"=w2112, "VDG compliance"=w2078, "IDG"=w2079, "VISA session"=w2113) -> ("error out"=w2114:errorcluster, "dup VISA resource name"=w2115:refnum<visa-resource-name>)  [unwired: 1 in]
        n616 = call "4155C Apply Stress.vi"("error in (no error)"=w2114, "Duration"=w2080, "Emergency Stop"=w2093, "VISA resource name in"=w2115) -> ("error out"=w2091:errorcluster, "VISA Resource Name out"=w2089:refnum<visa-resource-name>)
        n617 = VISA Write(VISA resource name=w2089, write buffer=":DISP ON" ("write buffer (\"\")"), error in (no error)=w2091) -> (VISA resource name out=w2088:refnum<visa-resource-name>, error out=w2090:errorcluster)  [unwired: 1 out]
        n618 = call <vilib>:"compatOverwrite.vi"("overwrite (F)"=TRUE) -> ("overwrite?"=w2077:T8)
        n619 = Open/Create/Replace File(file path (use dialog)=w2098, error in=w2090, operation (0:open)=w2077) -> (refnum out=w2101:refnum<file>, error out=w2100:errorcluster)  [unwired: 3 in, 1 out]
        n620 = call "4155C Write array to file.vi"("Byte Stream File Refnum"=w2101, "Header"=string[] ["I stress completed successfully", ""], "error in (no error)"=w2100) -> ("dup refnum"=w2103:refnum<file>, "error out"=w2102:errorcluster)  [unwired: 2 in]
        n621 = Close File(refnum=w2103, error in=w2102) -> (error out=w2096:errorcluster)  [unwired: 1 out]
      }
      frame "vsu2pulse" {
        n622 = Number To Decimal String(number=w2140) -> (decimal integer string=w2175:string)  [unwired: 1 in]
        n623 = Concatenate Strings(w2160, "-vsu2-" ("Substring"), w2175, w2139, ".txt" ("Substring")) -> (w2173:string)
        n624 = Fract/Exp String To Number(string=w2172) -> (number=w2148:dbl[])  [unwired: 3 in, 1 out]
        n625 = String To Path(string=w2173) -> (path=w2164:path)
        n626 = Index Array(array=w2148, index=1 ("Index")) -> (element=w2147:dbl)
        n627 = Index Array(array=w2148, index=0 ("Index")) -> (element=w2145:dbl)
        n628 = local read "VSU2 Stress - Source/Common"() -> (w2120:u32)
        n629 = call "4155C Config VSU2 Stress v3.0.vi"("VISA session"=w2178, "Display on/off"=TRUE, "VSU2"=w2145, "error in (no error)"=w2177, "VSU2 Stress - Source/Common"=w2120) -> ("dup VISA resource name"=w2180:refnum<visa-resource-name>, "error out"=w2179:errorcluster)
        n630 = call "4155C Apply Stress.vi"("error in (no error)"=w2179, "Duration"=w2147, "Emergency Stop"=w2159, "VISA resource name in"=w2180) -> ("error out"=w2157:errorcluster, "VISA Resource Name out"=w2155:refnum<visa-resource-name>)
        n631 = VISA Write(VISA resource name=w2155, write buffer=":DISP ON" ("write buffer (\"\")"), error in (no error)=w2157) -> (VISA resource name out=w2154:refnum<visa-resource-name>, error out=w2156:errorcluster)  [unwired: 1 out]
        n632 = call <vilib>:"compatOverwrite.vi"("overwrite (F)"=TRUE) -> ("overwrite?"=w2144:T8)
        n633 = Open/Create/Replace File(file path (use dialog)=w2164, error in=w2156, operation (0:open)=w2144) -> (refnum out=w2167:refnum<file>, error out=w2166:errorcluster)  [unwired: 3 in, 1 out]
        n634 = call "4155C Write array to file.vi"("Byte Stream File Refnum"=w2167, "Header"=string[] ["VSU2 pulse completed successfully", ""], "error in (no error)"=w2166) -> ("dup refnum"=w2169:refnum<file>, "error out"=w2168:errorcluster)  [unwired: 2 in]
        n635 = Close File(refnum=w2169, error in=w2168) -> (error out=w2162:errorcluster)  [unwired: 1 out]
      }
      frame "sample-fpp" {
        w2192 = 1
        w2250 = string[] ["Time /s", "Id VgVd /A", "Ig VgVd /A", "Vp1 VgVd /V", "Vp2 VgVd /V"] ("Header")
        w2254 = "%d" ("format string")
        # "Y1 = Y2 = ID\nY3 = IG"
        # "Y1 = Vp2\nY2 = Y3 = Vp1"
        # "Add a time offset (elapsed time) to the time axis."
        n636 = local read "FPP - Drain"() -> (w2227:u32)
        n637 = local read "FPP - Source"() -> (w2226:u32)
        n638 = local read "Plot sample extrema vs time"() -> (w2200:bool)
        n639 = Fract/Exp String To Number(string=w2293) -> (number=w2281:dbl[])  [unwired: 3 in, 1 out]
        n640 = local read "FPP - Probe 1"() -> (w2230:u32)
        n641 = Number To Decimal String(number=w2242) -> (decimal integer string=w2296:string)  [unwired: 1 in]
        n642 = local read "Plot sample extrema vs time"() -> (w2203:bool)
        n643 = Concatenate Strings(w2287, "-samplefpp-" ("Substring"), w2296, w2241, ".txt" ("Substring")) -> (w2294:string)
        n644 = local read "FPP - Gate"() -> (w2228:u32)
        n645 = local read "Time Units"() -> (w2218:u16)
        n646 = String To Path(string=w2294) -> (path=w2262:path)
        n647 = local read "FPP - Probe 2"() -> (w2229:u32)
        n648 = Index Array(array=w2281, index=0 ("Index")) -> (element=w2249:dbl)
        n649 = Index Array(array=w2281, index=1 ("Index")) -> (element=w2248:dbl)
        n650 = control-ref of="I vs time (Bias Stress)"() -> (w2220:refnum<vi>)
        n651 = Index Array(array=w2281, index=2 ("Index")) -> (element=w2289:dbl)
        n652 = Index Array(array=w2281, index=3 ("Index")) -> (element=w2279:dbl)
        n653 = call "4155C Config Sampling Measurements FPP v3.0.vi"("VISA session"=w2299, "Gate Compliance"=w2288, "FPP - Source"=w2226, "FPP - Drain"=w2227, "Drain Compliance"=w2297, "error in (no error)"=w2298, "Num Points"=w2289, "Timings"=w2286, "FPP - Gate"=w2228, "FPP - Probe 1"=w2230, "Vg"=w2249, "Vd"=w2248, "Display on/off"=TRUE, "Sample time"=w2279, "FPP - Probe 2"=w2229, "Standby"=w2231) -> ("dup VISA resource name"=w2264:refnum<visa-resource-name>, "error out"=w2263:errorcluster)  [unwired: 2 in]
        n654 = Number To Decimal String(number=w2249) -> (decimal integer string=w2270:string)  [unwired: 1 in]
        n655 = call "4155C Take Sample FPP.vi"("VISA resource name in"=w2264, "error in (no error)"=w2263, "Emergency Stop"=w2265) -> ("Time"=w2217:dbl[], "Vp1"=w2186:dbl[], "VISA Resource Name out"=w2246:refnum<visa-resource-name>, "Ig"=w2197:dbl[], "Id"=w2196:dbl[], "Vp2"=w2185:dbl[], "error out"=w2199:errorcluster)  [unwired: 10 in]
        n656 = Insert Into Array(array=w2224, new element=w2196) -> (w2183:dbl[])  [unwired: 1 in]
        n657 = Insert Into Array(array=w2225, new element=w2197) -> (w2222:dbl[])  [unwired: 1 in]
        n658 = case shown="0, Default" w2218 {
          tunnel: [w2339 w2340 w2343] -> w2219
          tunnel: w2217 -> [w2338 w2340 w2342]
          frame 2 {
            n659 = Divide(x=w2338, y=3600.0) -> (x/y=w2339:dbl[])
          }
          frame 0, Default {
          }
          frame 1 {
            n660 = Divide(x=w2342, y=60.0) -> (x/y=w2343:dbl[])
          }
        }
        n661 = Add(x=w2219, y=w2216) -> (x+y=w2190:dbl[])
        n662 = case shown="True" w2200 {
          tunnel: w2202 -> [w2300 w2302]
          tunnel: [w2300 w2303] -> w2201
          tunnel: w2190 -> [_ w2301]
          frame False {
          }
          frame True {
            n663 = Insert Into Array(array=w2302, new element=w2301) -> (w2303:i32[])  [unwired: 1 in]
          }
        }
        n664 = Insert Into Array(array=w2223, new element=w2190) -> (w2191:dbl[])  [unwired: 1 in]
        n665 = case shown="True" w2203 {
          tunnel: w2196 -> [_ w2328]
          tunnel: w2197 -> [_ w2329]
          tunnel: [w2310 w2320] -> w2198
          tunnel: w2199 -> [w2310 w2323]
          tunnel: w2215 -> [w2309 w2313]
          tunnel: w2214 -> [w2308 w2312]
          tunnel: w2213 -> [w2307 w2331]
          tunnel: w2212 -> [w2306 w2330]
          tunnel: w2211 -> [w2305 w2333]
          tunnel: w2210 -> [w2304 w2332]
          tunnel: [w2309 w2313] -> w2209
          tunnel: [w2308 w2312] -> w2208
          tunnel: [w2307 w2311] -> w2207
          tunnel: [w2306 w2334] -> w2206
          tunnel: [w2305 w2322] -> w2205
          tunnel: [w2304 w2317] -> w2204
          tunnel: w2201 -> [_ w2314]
          frame False {
          }
          frame True {
            w2318 = 1
            # "Y1 = Y2 = ID\nY3 = IG"
            # "Number of VAR2 steps is 1."
            # "abs(Ig)"
            # "abs(Id)"
            # "Adjusts graph colors."
            n666 = Absolute Value(x=w2329) -> (abs(x)=w2315:dbl[])
            n667 = Absolute Value(x=w2328) -> (abs(x)=w2316:dbl[])
            n668 = Array Max & Min(array=w2316) -> (max value=w2327:dbl, min value=w2325:dbl)  [unwired: 2 out]
            n669 = Array Max & Min(array=w2315) -> (max value=w2326:dbl, min value=w2324:dbl)  [unwired: 2 out]
            n670 = local write "Id max"(w2327) -> ()
            n671 = local write "Id min"(w2325) -> ()
            n672 = local write "Ig max"(w2326) -> ()
            n673 = local write "Ig min"(w2324) -> ()
            n674 = Insert Into Array(array=w2333, new element=w2315) -> (w2322:dbl[])  [unwired: 1 in]
            n675 = Insert Into Array(array=w2332, new element=w2315) -> (w2317:dbl[])  [unwired: 1 in]
            n676 = Insert Into Array(array=w2331, new element=w2316) -> (w2311:dbl[])  [unwired: 1 in]
            n677 = Insert Into Array(array=w2330, new element=w2316) -> (w2334:dbl[])  [unwired: 1 in]
            n678 = control-ref of="Imax vs time"() -> (w2335:refnum<vi>)
            n679 = call "4155C Config Chart Colours.vi"("Numeric"=w2318, "XY Graph 2"=w2335) -> ()  [unwired: 6 in]
            n680 = call "4155C Split array.vi"("Number of VAR2 steps"=w2318, "Y2 data in"=w2311, "X data in"=w2314, "Y1 data in"=w2311, "Y3 data in"=w2322, "error in (no error)"=w2323) -> ("Array of clusters"=w2336:cluster{"Y data in":dbl[], "X data in":dbl[]}[], "error out"=w2321:errorcluster)  [unwired: 1 in]
            n681 = call "4155C Split array.vi"("Number of VAR2 steps"=w2318, "Y2 data in"=w2311, "X data in"=w2314, "Y1 data in"=w2311, "Y3 data in"=w2317, "error in (no error)"=w2321) -> ("Array of clusters"=w2319:cluster{"Y data in":dbl[], "X data in":dbl[]}[], "error out"=w2320:errorcluster)  [unwired: 1 in]
            n682 = local write "Imax vs time"(w2336) -> ()
            n683 = local write "Imin vs time"(w2319) -> ()
          }
        }
        n684 = call "4155C Split array.vi"("Number of VAR2 steps"=w2192, "Y2 data in"=w2183, "X data in"=w2191, "Y1 data in"=w2183, "Y3 data in"=w2222) -> ("Array of clusters"=w2221:cluster{"Y data in":dbl[], "X data in":dbl[]}[])  [unwired: 2 in, 1 out]
        n685 = call "4155C Config Chart Colours.vi"("Numeric"=w2192, "XY Graph 2"=w2220) -> ()  [unwired: 6 in]
        n686 = local write "I vs time (Bias Stress)"(w2221) -> ()
        n687 = Number To Decimal String(number=w2248) -> (decimal integer string=w2268:string)  [unwired: 1 in]
        n688 = Insert Into Array(array=w2189, new element=w2186) -> (w2184:dbl[])  [unwired: 1 in]
        n689 = Concatenate Strings("(Vg = " ("Substring"), w2270, "V, Vd = " ("Substring"), w2268, "V)" ("Substring")) -> (w2266:string)
        n690 = Insert Into Array(array=dbl[][] [] ("Input Array"), new element=w2190) -> (w2277:dbl[][])  [unwired: 2 in]
        n691 = Insert Into Array(array=w2188, new element=w2185) -> (w2187:dbl[])  [unwired: 1 in]
        n692 = Insert Into Array(array=w2277, new element=w2196) -> (w2276:dbl[][])  [unwired: 2 in]
        n693 = control-ref of="Vp vs time (FPP Bias Stress)"() -> (w2193:refnum<vi>)
        n694 = Insert Into Array(array=w2276, new element=w2197) -> (w2275:dbl[][])  [unwired: 2 in]
        n695 = Insert Into Array(array=w2275, new element=w2186) -> (w2273:dbl[][])  [unwired: 2 in]
        n696 = call "4155C Config Chart Colours.vi"("Numeric"=w2192, "XY Graph 2"=w2193) -> ()  [unwired: 6 in]
        n697 = call "4155C Split array.vi"("Number of VAR2 steps"=w2192, "Y2 data in"=w2184, "X data in"=w2191, "Y1 data in"=w2187, "Y3 data in"=w2184) -> ("Array of clusters"=w2194:cluster{"Y data in":dbl[], "X data in":dbl[]}[])  [unwired: 2 in, 1 out]
        n698 = Array To Spreadsheet String(array=w2250, 3:w2254) -> (spreadsheet string=w2256:string)  [unwired: 1 in]
        n699 = Insert Into Array(array=w2273, new element=w2185) -> (w2247:dbl[][])  [unwired: 2 in]
        n700 = Search and Replace String(replace all?=TRUE ("replace all? (F)"), input string=w2256, search string="VgVd", replace string=w2266) -> (result string=w2252:string)  [unwired: 4 in, 3 out]
        n701 = local write "Vp vs time (FPP Bias Stress)"(w2194) -> ()
        n702 = Spreadsheet String To Array(format string=w2254, spreadsheet string=w2252, array type (2D Dbl)=w2250) -> (array=w2251:string[])  [unwired: 1 in]
        n703 = Transpose 2D Array(2D array=w2247) -> (transposed array=w2272:dbl[][])
        n704 = call <vilib>:"compatOverwrite.vi"("overwrite (F)"=TRUE) -> ("overwrite?"=w2244:T8)
        n705 = Open/Create/Replace File(file path (use dialog)=w2262, error in=w2198, operation (0:open)=w2244) -> (refnum out=w2259:refnum<file>, error out=w2260:errorcluster)  [unwired: 3 in, 1 out]
        n706 = call "4155C Write array to file.vi"("Byte Stream File Refnum"=w2259, "Header"=w2251, "Data Array"=w2272, "error in (no error)"=w2260) -> ("dup refnum"=w2257:refnum<file>, "error out"=w2258:errorcluster)  [unwired: 1 in]
        n707 = Close File(refnum=w2257, error in=w2258) -> (error out=w2245:errorcluster)  [unwired: 1 out]
      }
      frame "resample-fpp" {
        w2355 = 1
        w2410 = string[] ["Time /s", "Id VgVd /A", "Ig VgVd /A", "Vp1 VgVd /V", "Vp2 VgVd /V"] ("Header")
        w2414 = "%d" ("format string")
        # "Y1 = Y2 = ID\nY3 = IG"
        # "Y1 = Vp2\nY2 = Y3 = Vp1"
        # "Add a time offset (elapsed time) to the time axis."
        n708 = Number To Decimal String(number=w2398) -> (decimal integer string=w2448:string)  [unwired: 1 in]
        n709 = Fract/Exp String To Number(string=w2445) -> (number=w2403:dbl[])  [unwired: 3 in, 1 out]
        n710 = Concatenate Strings(w2441, "-resamplefpp-" ("Substring"), w2448, w2399, ".txt" ("Substring")) -> (w2446:string)
        n711 = local read "Time Units"() -> (w2379:u16)
        n712 = local read "Plot sample extrema vs time"() -> (w2377:bool)
        n713 = String To Path(string=w2446) -> (path=w2422:path)
        n714 = Index Array(array=w2403, index=0 ("Index")) -> (element=w2409:dbl)
        n715 = Index Array(array=w2403, index=1 ("Index")) -> (element=w2408:dbl)
        n716 = Number To Decimal String(number=w2409) -> (decimal integer string=w2428:string)  [unwired: 1 in]
        n717 = call "4155C Take Sample FPP.vi"("VISA resource name in"=w2405, "error in (no error)"=w2404, "Emergency Stop"=w2423) -> ("Time"=w2380:dbl[], "Vp1"=w2349:dbl[], "VISA Resource Name out"=w2407:refnum<visa-resource-name>, "Ig"=w2360:dbl[], "Id"=w2359:dbl[], "Vp2"=w2348:dbl[], "error out"=w2362:errorcluster)  [unwired: 10 in]
        n718 = Insert Into Array(array=w2387, new element=w2359) -> (w2346:dbl[])  [unwired: 1 in]
        n719 = case shown="0, Default" w2379 {
          tunnel: [w2489 w2490 w2493] -> w2381
          tunnel: w2380 -> [w2488 w2490 w2492]
          frame 2 {
            n720 = Divide(x=w2488, y=3600.0) -> (x/y=w2489:dbl[])
          }
          frame 0, Default {
          }
          frame 1 {
            n721 = Divide(x=w2492, y=60.0) -> (x/y=w2493:dbl[])
          }
        }
        n722 = Insert Into Array(array=w2388, new element=w2360) -> (w2385:dbl[])  [unwired: 1 in]
        n723 = control-ref of="I vs time (Bias Stress)"() -> (w2383:refnum<vi>)
        n724 = Number To Decimal String(number=w2408) -> (decimal integer string=w2426:string)  [unwired: 1 in]
        n725 = Add(x=w2381, y=w2382) -> (x+y=w2353:dbl[])
        n726 = Insert Into Array(array=w2386, new element=w2353) -> (w2354:dbl[])  [unwired: 1 in]
        n727 = call "4155C Split array.vi"("Number of VAR2 steps"=w2355, "Y2 data in"=w2346, "X data in"=w2354, "Y1 data in"=w2346, "Y3 data in"=w2385) -> ("Array of clusters"=w2384:cluster{"Y data in":dbl[], "X data in":dbl[]}[])  [unwired: 2 in, 1 out]
        n728 = Concatenate Strings("(Vg = " ("Substring"), w2428, "V, Vd = " ("Substring"), w2426, "V)" ("Substring")) -> (w2424:string)
        n729 = call "4155C Config Chart Colours.vi"("Numeric"=w2355, "XY Graph 2"=w2383) -> ()  [unwired: 6 in]
        n730 = local write "I vs time (Bias Stress)"(w2384) -> ()
        n731 = Insert Into Array(array=dbl[][] [] ("Input Array"), new element=w2353) -> (w2435:dbl[][])  [unwired: 2 in]
        n732 = Insert Into Array(array=w2435, new element=w2359) -> (w2434:dbl[][])  [unwired: 2 in]
        n733 = Insert Into Array(array=w2434, new element=w2360) -> (w2433:dbl[][])  [unwired: 2 in]
        n734 = Array To Spreadsheet String(array=w2410, 3:w2414) -> (spreadsheet string=w2416:string)  [unwired: 1 in]
        n735 = Insert Into Array(array=w2433, new element=w2349) -> (w2431:dbl[][])  [unwired: 2 in]
        n736 = Insert Into Array(array=w2352, new element=w2349) -> (w2347:dbl[])  [unwired: 1 in]
        n737 = Search and Replace String(replace all?=TRUE ("replace all? (F)"), input string=w2416, search string="VgVd", replace string=w2424) -> (result string=w2412:string)  [unwired: 4 in, 3 out]
        n738 = Insert Into Array(array=w2431, new element=w2348) -> (w2402:dbl[][])  [unwired: 2 in]
        n739 = Insert Into Array(array=w2351, new element=w2348) -> (w2350:dbl[])  [unwired: 1 in]
        n740 = Spreadsheet String To Array(format string=w2414, spreadsheet string=w2412, array type (2D Dbl)=w2410) -> (array=w2411:string[])  [unwired: 1 in]
        n741 = control-ref of="Vp vs time (FPP Bias Stress)"() -> (w2356:refnum<vi>)
        n742 = local read "Plot sample extrema vs time"() -> (w2364:bool)
        n743 = call <vilib>:"compatOverwrite.vi"("overwrite (F)"=TRUE) -> ("overwrite?"=w2401:T8)
        n744 = Transpose 2D Array(2D array=w2402) -> (transposed array=w2430:dbl[][])
        n745 = call "4155C Config Chart Colours.vi"("Numeric"=w2355, "XY Graph 2"=w2356) -> ()  [unwired: 6 in]
        n746 = call "4155C Split array.vi"("Number of VAR2 steps"=w2355, "Y2 data in"=w2347, "X data in"=w2354, "Y1 data in"=w2350, "Y3 data in"=w2347) -> ("Array of clusters"=w2357:cluster{"Y data in":dbl[], "X data in":dbl[]}[])  [unwired: 2 in, 1 out]
        n747 = case shown="True" w2364 {
          tunnel: w2365 -> [w2450 w2452]
          tunnel: [w2450 w2453] -> w2363
          tunnel: w2353 -> [_ w2451]
          frame False {
          }
          frame True {
            n748 = Insert Into Array(array=w2452, new element=w2451) -> (w2453:i32[])  [unwired: 1 in]
          }
        }
        n749 = case shown="True" w2377 {
          tunnel: w2359 -> [_ w2478]
          tunnel: w2360 -> [_ w2479]
          tunnel: [w2460 w2470] -> w2361
          tunnel: w2362 -> [w2460 w2473]
          tunnel: w2378 -> [w2459 w2463]
          tunnel: w2375 -> [w2458 w2462]
          tunnel: w2374 -> [w2457 w2481]
          tunnel: w2373 -> [w2456 w2480]
          tunnel: w2372 -> [w2455 w2483]
          tunnel: w2371 -> [w2454 w2482]
          tunnel: [w2459 w2463] -> w2376
          tunnel: [w2458 w2462] -> w2366
          tunnel: [w2457 w2461] -> w2368
          tunnel: [w2456 w2484] -> w2367
          tunnel: [w2455 w2472] -> w2370
          tunnel: [w2454 w2467] -> w2369
          tunnel: w2363 -> [_ w2464]
          frame False {
          }
          frame True {
            w2468 = 1
            # "Y1 = Y2 = ID\nY3 = IG"
            # "Number of VAR2 steps is 1."
            # "abs(Ig)"
            # "abs(Id)"
            # "Adjusts graph colors."
            n750 = Absolute Value(x=w2479) -> (abs(x)=w2465:dbl[])
            n751 = Absolute Value(x=w2478) -> (abs(x)=w2466:dbl[])
            n752 = Array Max & Min(array=w2466) -> (max value=w2477:dbl, min value=w2475:dbl)  [unwired: 2 out]
            n753 = Array Max & Min(array=w2465) -> (max value=w2476:dbl, min value=w2474:dbl)  [unwired: 2 out]
            n754 = local write "Id max"(w2477) -> ()
            n755 = local write "Id min"(w2475) -> ()
            n756 = local write "Ig max"(w2476) -> ()
            n757 = local write "Ig min"(w2474) -> ()
            n758 = Insert Into Array(array=w2483, new element=w2465) -> (w2472:dbl[])  [unwired: 1 in]
            n759 = Insert Into Array(array=w2482, new element=w2465) -> (w2467:dbl[])  [unwired: 1 in]
            n760 = Insert Into Array(array=w2481, new element=w2466) -> (w2461:dbl[])  [unwired: 1 in]
            n761 = Insert Into Array(array=w2480, new element=w2466) -> (w2484:dbl[])  [unwired: 1 in]
            n762 = control-ref of="Imax vs time"() -> (w2485:refnum<vi>)
            n763 = call "4155C Config Chart Colours.vi"("Numeric"=w2468, "XY Graph 2"=w2485) -> ()  [unwired: 6 in]
            n764 = call "4155C Split array.vi"("Number of VAR2 steps"=w2468, "Y2 data in"=w2461, "X data in"=w2464, "Y1 data in"=w2461, "Y3 data in"=w2472, "error in (no error)"=w2473) -> ("Array of clusters"=w2486:cluster{"Y data in":dbl[], "X data in":dbl[]}[], "error out"=w2471:errorcluster)  [unwired: 1 in]
            n765 = call "4155C Split array.vi"("Number of VAR2 steps"=w2468, "Y2 data in"=w2461, "X data in"=w2464, "Y1 data in"=w2461, "Y3 data in"=w2467, "error in (no error)"=w2471) -> ("Array of clusters"=w2469:cluster{"Y data in":dbl[], "X data in":dbl[]}[], "error out"=w2470:errorcluster)  [unwired: 1 in]
            n766 = local write "Imax vs time"(w2486) -> ()
            n767 = local write "Imin vs time"(w2469) -> ()
          }
        }
        n768 = Open/Create/Replace File(file path (use dialog)=w2422, error in=w2361, operation (0:open)=w2401) -> (refnum out=w2419:refnum<file>, error out=w2420:errorcluster)  [unwired: 3 in, 1 out]
        n769 = call "4155C Write array to file.vi"("Byte Stream File Refnum"=w2419, "Header"=w2411, "Data Array"=w2430, "error in (no error)"=w2420) -> ("dup refnum"=w2417:refnum<file>, "error out"=w2418:errorcluster)  [unwired: 1 in]
        n770 = local write "Vp vs time (FPP Bias Stress)"(w2357) -> ()
        n771 = Close File(refnum=w2417, error in=w2418) -> (error out=w2406:errorcluster)  [unwired: 1 out]
      }
      frame "serial" {
        n772 = local read "Termination char\n(0xA = '\\n' = LF)\n(0xD = '\\r' = CR)"() -> (w2523:u8)
        n773 = local read "Enable Termination\nChar (T)"() -> (w2524:bool)
        n774 = Index Array(array=w2531, index=0 ("Index")) -> (element=w2530:string)
        n775 = local read "parity"() -> (w2514:u16)
        n776 = local read "Delay before read (ms)"() -> (w2525:u32)
        n777 = local read "byte count"() -> (w2522:u32)
        n778 = local read "VISA resource name"() -> (w2518:refnum<visa-resource-name>)
        n779 = local read "baud rate"() -> (w2517:u32)
        n780 = local read "Serial End Mode for Reads"() -> (w2516:u16)
        n781 = local read "Timeout (ms)"() -> (w2521:u32)
        n782 = local read "data bits"() -> (w2515:u16)
        n783 = local read "stop bits"() -> (w2520:u16)
        n784 = local read "flow control"() -> (w2519:u16)
        n785 = call "Serial write and read v0.5.vi"("Delay before read (ms)"=w2525, "Termination char\n(0xA = '\\n' = LF)\n(0xD = '\\r' = CR)"=w2523, "Enable Termination\nChar (T)"=w2524, "parity"=w2514, "stop bits"=w2520, "string to write"=w2530, "flow control"=w2519, "byte count"=w2522, "Serial Settings:Serial End Mode for Reads"=w2516, "Timeout (ms)"=w2521, "error in (no error)"=w2536, "VISA resource name"=w2518, "baud rate"=w2517, "data bits"=w2515) -> ("Serial port output"=w2526:string, "error out"=w2535:errorcluster)
        n786 = Build Array (concatenate)(w2526, w2527) -> (w2528:string[])
      }
    }
    "Probe 4 Indicator" <- w71
    "Timings Indicator" <- w72
    n787 = local read "Time Units"() -> (w105:u16)
    n788 = case shown="0" w105 {
      tunnel: ["Time (Seconds)" ("element") "Time (Minutes)" ("element") "Time (Hours)" ("element")] -> w74
      frame 0 {
      }
      frame 1, Default {
      }
      frame 2 {
      }
    }
    n789 = Build Array(w154, w111, w121, w120, w119, w118, w117, w116, w115, w114, w113, w112, w110) -> (w175:dbl[][])
    n790 = Transpose 2D Array(2D array=w175) -> (transposed array=w174:dbl[][])
    n791 = Concatenate Strings(w80, "-I-vs-time.txt" ("Suffix (Imax,Imin,Ion,Ioff)")) -> (w185:string)
    n792 = Build Array(w74, "Is max (A)" ("VAR2 Name"), "Is min (A)" ("VAR2 Name"), "Id max (A)" ("VAR2 Name"), "Id min (A)" ("VAR2 Name"), "Ig max (A)" ("VAR2 Name"), "Ig min (A)" ("VAR2 Name"), "Is on (A)" ("VAR2 Name"), "Is off (A)" ("VAR2 Name"), "Id on (A)" ("VAR2 Name"), "Id off (A)" ("VAR2 Name"), "Ig on (A)" ("VAR2 Name"), "Ig off (A)" ("VAR2 Name")) -> (w180:string[])
    n793 = Array To Spreadsheet String(array=w174, 3:"%e" ("format string")) -> (spreadsheet string=w178:string)  [unwired: 1 in]
    n794 = Array To Spreadsheet String(array=w180, 3:"" ("format string")) -> (spreadsheet string=w179:string)  [unwired: 1 in]
    n795 = String To Path(string=w185) -> (path=w184:path)
    n796 = Build Array(w179, w178) -> (w177:string[])
    n797 = Write to Text File(file (use dialog)=w184, text=w177, error in=w153) -> (refnum out=w186:refnum<file>, error out=w176:errorcluster)  [unwired: 1 in, 1 out]
    n798 = Close File(refnum=w186, error in=w176) -> (error out=w108:errorcluster)  [unwired: 1 out]
    n799 = Concatenate Strings(w80, "-serial-port.txt" ("Suffix (serial port log)")) -> (w156:string)
    n800 = String To Path(string=w156) -> (path=w155:path)
    n801 = Build Array(w74, "Serial port input" ("VAR2 Name"), "Serial port output: ") -> (w146:string[])
    n802 = Array To Spreadsheet String(array=w150, 3:"" ("format string")) -> (spreadsheet string=w143:string)  [unwired: 1 in]
    n803 = Array To Spreadsheet String(array=w146, 3:"" ("format string")) -> (spreadsheet string=w144:string)  [unwired: 1 in]
    n804 = Build Array(w144, w143) -> (w145:string[])
    n805 = Array To Spreadsheet String(array=w149, 3:"" ("format string")) -> (spreadsheet string=w161:string)  [unwired: 1 in]
    n806 = Write to Text File(file (use dialog)=w155, text=w145, error in=w108) -> (refnum out=w157:refnum<file>, error out=w158:errorcluster)  [unwired: 1 in, 1 out]
    n807 = Close File(refnum=w157, error in=w158) -> (error out=w81:errorcluster)  [unwired: 1 out]
    n808 = local write "Serial port data"(w161) -> ()
    n809 = Build Array(w79, w78, w77, w76) -> (w90:dbl[][])
    n810 = Build Array(w74, "Is (A)" ("VAR2 Name"), "Id (A)" ("VAR2 Name"), "Ig (A)" ("VAR2 Name")) -> (w86:string[])
    n811 = Transpose 2D Array(2D array=w90) -> (transposed array=w89:dbl[][])
    n812 = Concatenate Strings(w80, "-sample.txt" ("Suffix (Imax,Imin,Ion,Ioff)")) -> (w96:string)
    n813 = Array To Spreadsheet String(array=w86, 3:"" ("format string")) -> (spreadsheet string=w85:string)  [unwired: 1 in]
    n814 = Array To Spreadsheet String(array=w89, 3:"%e" ("format string")) -> (spreadsheet string=w93:string)  [unwired: 1 in]
    n815 = String To Path(string=w96) -> (path=w95:path)
    n816 = Build Array(w85, w93) -> (w92:string[])
    n817 = Write to Text File(file (use dialog)=w95, text=w92, error in=w81) -> (refnum out=w97:refnum<file>, error out=w91:errorcluster)  [unwired: 1 in, 1 out]
    n818 = Close File(refnum=w97, error in=w91) -> (error out=w73:errorcluster)  [unwired: 1 out]
    "error out" <- w73
  }
  "Is max" <- w15
  "Id max" <- w15
  "Ig max" <- w15
  "Imax vs time" <- w4
  "I vs Vg" <- w4
  "Imin vs time" <- w4
  "I vs Vd" <- w4
  "Serial port data" <- "" ("Serial port data")
  "Is min" <- w14
  "Id min" <- w14
  "Ig min" <- w14
  "Ion vs time" <- w4
  "Ioff vs time" <- w4
  "Is on" <- w13
  "Id on" <- w13
  "Ig on" <- w13
  "Is off" <- w12
  "Id off" <- w12
  "Ig off" <- w12
  "I vs time (Bias Stress)" <- w4
  "Vp1" <- w5
  "Vp2" <- w5
  "Vp vs time (FPP Bias Stress)" <- w4
  "Vp vs Vg (FPP)" <- w4
  "Vdg vs time (Bias Stress)" <- w4
